vi "PLC_comm-Modified.vi"() -> ()   [LabVIEW 2017]
uses:
  <vilib>/Utility/error.llb/DialogType.ctl
  Control/PLC_Comm_State.ctl
  <vilib>/DATA AHEAD/SP7/typedefs/PLC Type.ctl
  <vilib>/DATA AHEAD/SP7/typedefs/S7 Connection.ctl
  f53d9a16-31ea-4c58-9ec6-4ab155e6634a.vi
  b767813d-b0bc-4642-82b7-59e8eeaf8486.vi
  cf2a4f70-d875-4391-b4be-4b1ea527ec99.vi
  ee8abbcb-1732-468d-97ec-3952c14652c8.vi
  b1e76c00-34b1-4c80-90c6-025f7ce7f41f.vi
  f2e501b8-8033-40fd-b99e-90a89dd29cf5.vi
  90770c14-337c-420b-89b5-e528e61782e2.vi
  a17ecfbb-e8aa-4e6f-9723-a9b27e8c0652.vi
  7947ba3e-47d3-4313-89af-b8503fb010f5.vi
  adc7d8b8-ea76-443b-992e-07ffa118bf03.vi
  515b9a70-e7fd-440a-92eb-3997303c16bf.vi
  5f64c4b0-8bc9-4820-bee4-0d99e36e3286.vi
  3deaaee4-0312-4209-8b7c-ccc637c44985.vi
  e6818258-ddc9-43a8-9628-6e9a25c2df97.vi
  <vilib>/addons/database/Connection.llb/DB Tools Open Connec (String).vi
  <vilib>/DATA AHEAD/SP7/functions/write/write Dint array.vi
  Global/DATA LOG.vi
  <vilib>/DATA AHEAD/SP7/functions/read/read String.vi
  <vilib>/DATA AHEAD/SP7/functions/read/read Dint array.vi
  Global/Global 1.vi
  <vilib>/DATA AHEAD/SP7/functions/write/writeString.vi
  <vilib>/DATA AHEAD/SP7/functions/read/read real array.vi
  <vilib>/addons/database/NI_Database_API.lvlib
  <vilib>/DATA AHEAD/SP7/SP7.lvlib
  84f8396c-11e3-4f6e-927f-d6cb52f8486f.vi
  edb3f7e3-deb4-4efd-b63a-82a20ab466dd.vi
  737c4a97-5810-4f09-bfe1-7e6a970161fd.vi
  98a23aa7-5d76-4ce5-89a1-7ffa2d6e86d6.vi
  065602cd-1ec6-46a4-aff5-3b00a0c776c3.vi
panel:
  out "error out 4":errorcluster
  out "error out 3":errorcluster
  out "IP1 8":string
  out "PLC 8":bool
  out "IP1 7":string
  out "PLC 7":bool
  out "IP1 6":string
  out "PLC 6":bool
  out "IP1 5":string
  out "PLC 5":bool
  out "PLC 4":bool
  out "PLC 3":bool
  out "PLC 1":bool
  out "IP1 4":string
  out "IP1 3":string
  out "IP1 2":string
  out "IP1":string
  in  "stop":bool
  out "error out":errorcluster
  in  "error in (no error)":errorcluster
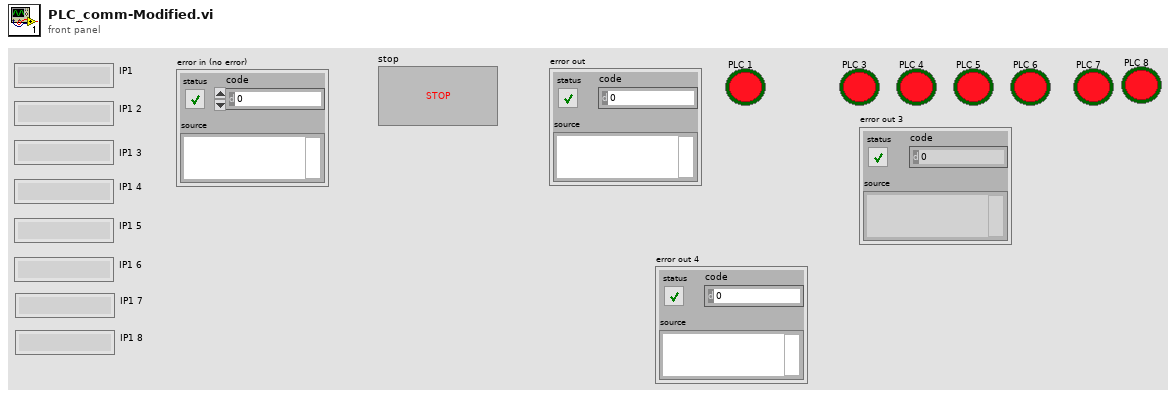
[diagram p1: front panel]
types:
  T1 = typedef "PLC_Comm_State.ctl" = enum16{"Int", "Connect", "Write", "Write2", "Write3", "Read", "Read2", "Read3", "Error", "Disconnect"}
  T2 = typedef "DialogType.ctl" = u16
  T3 = typedef "NI_Database_API.lvlib/Conn ObjectReference.ctl" = refnum<k1>
  T4 = typedef "SP7.lvlib/PLC Type.ctl" = enum16{"S7 200", "S7 300/400", "S7 1200", "S7 1500", "LOGO!8"}
  T5 = typedef "SP7.lvlib/S7 Connection.ctl" = cluster{"TCP Connection Ref":refnum<k5>, "IP address":string, "timeout ms":i32, "Connected?":bool, "PLC Type":T4, "Rack S7 400":u8, "Slot S7 400":u8, "PDU Size":u16, "connection semaphore":T6}
  T6 = typedef "Semaphore RefNum" = refnum<k1>
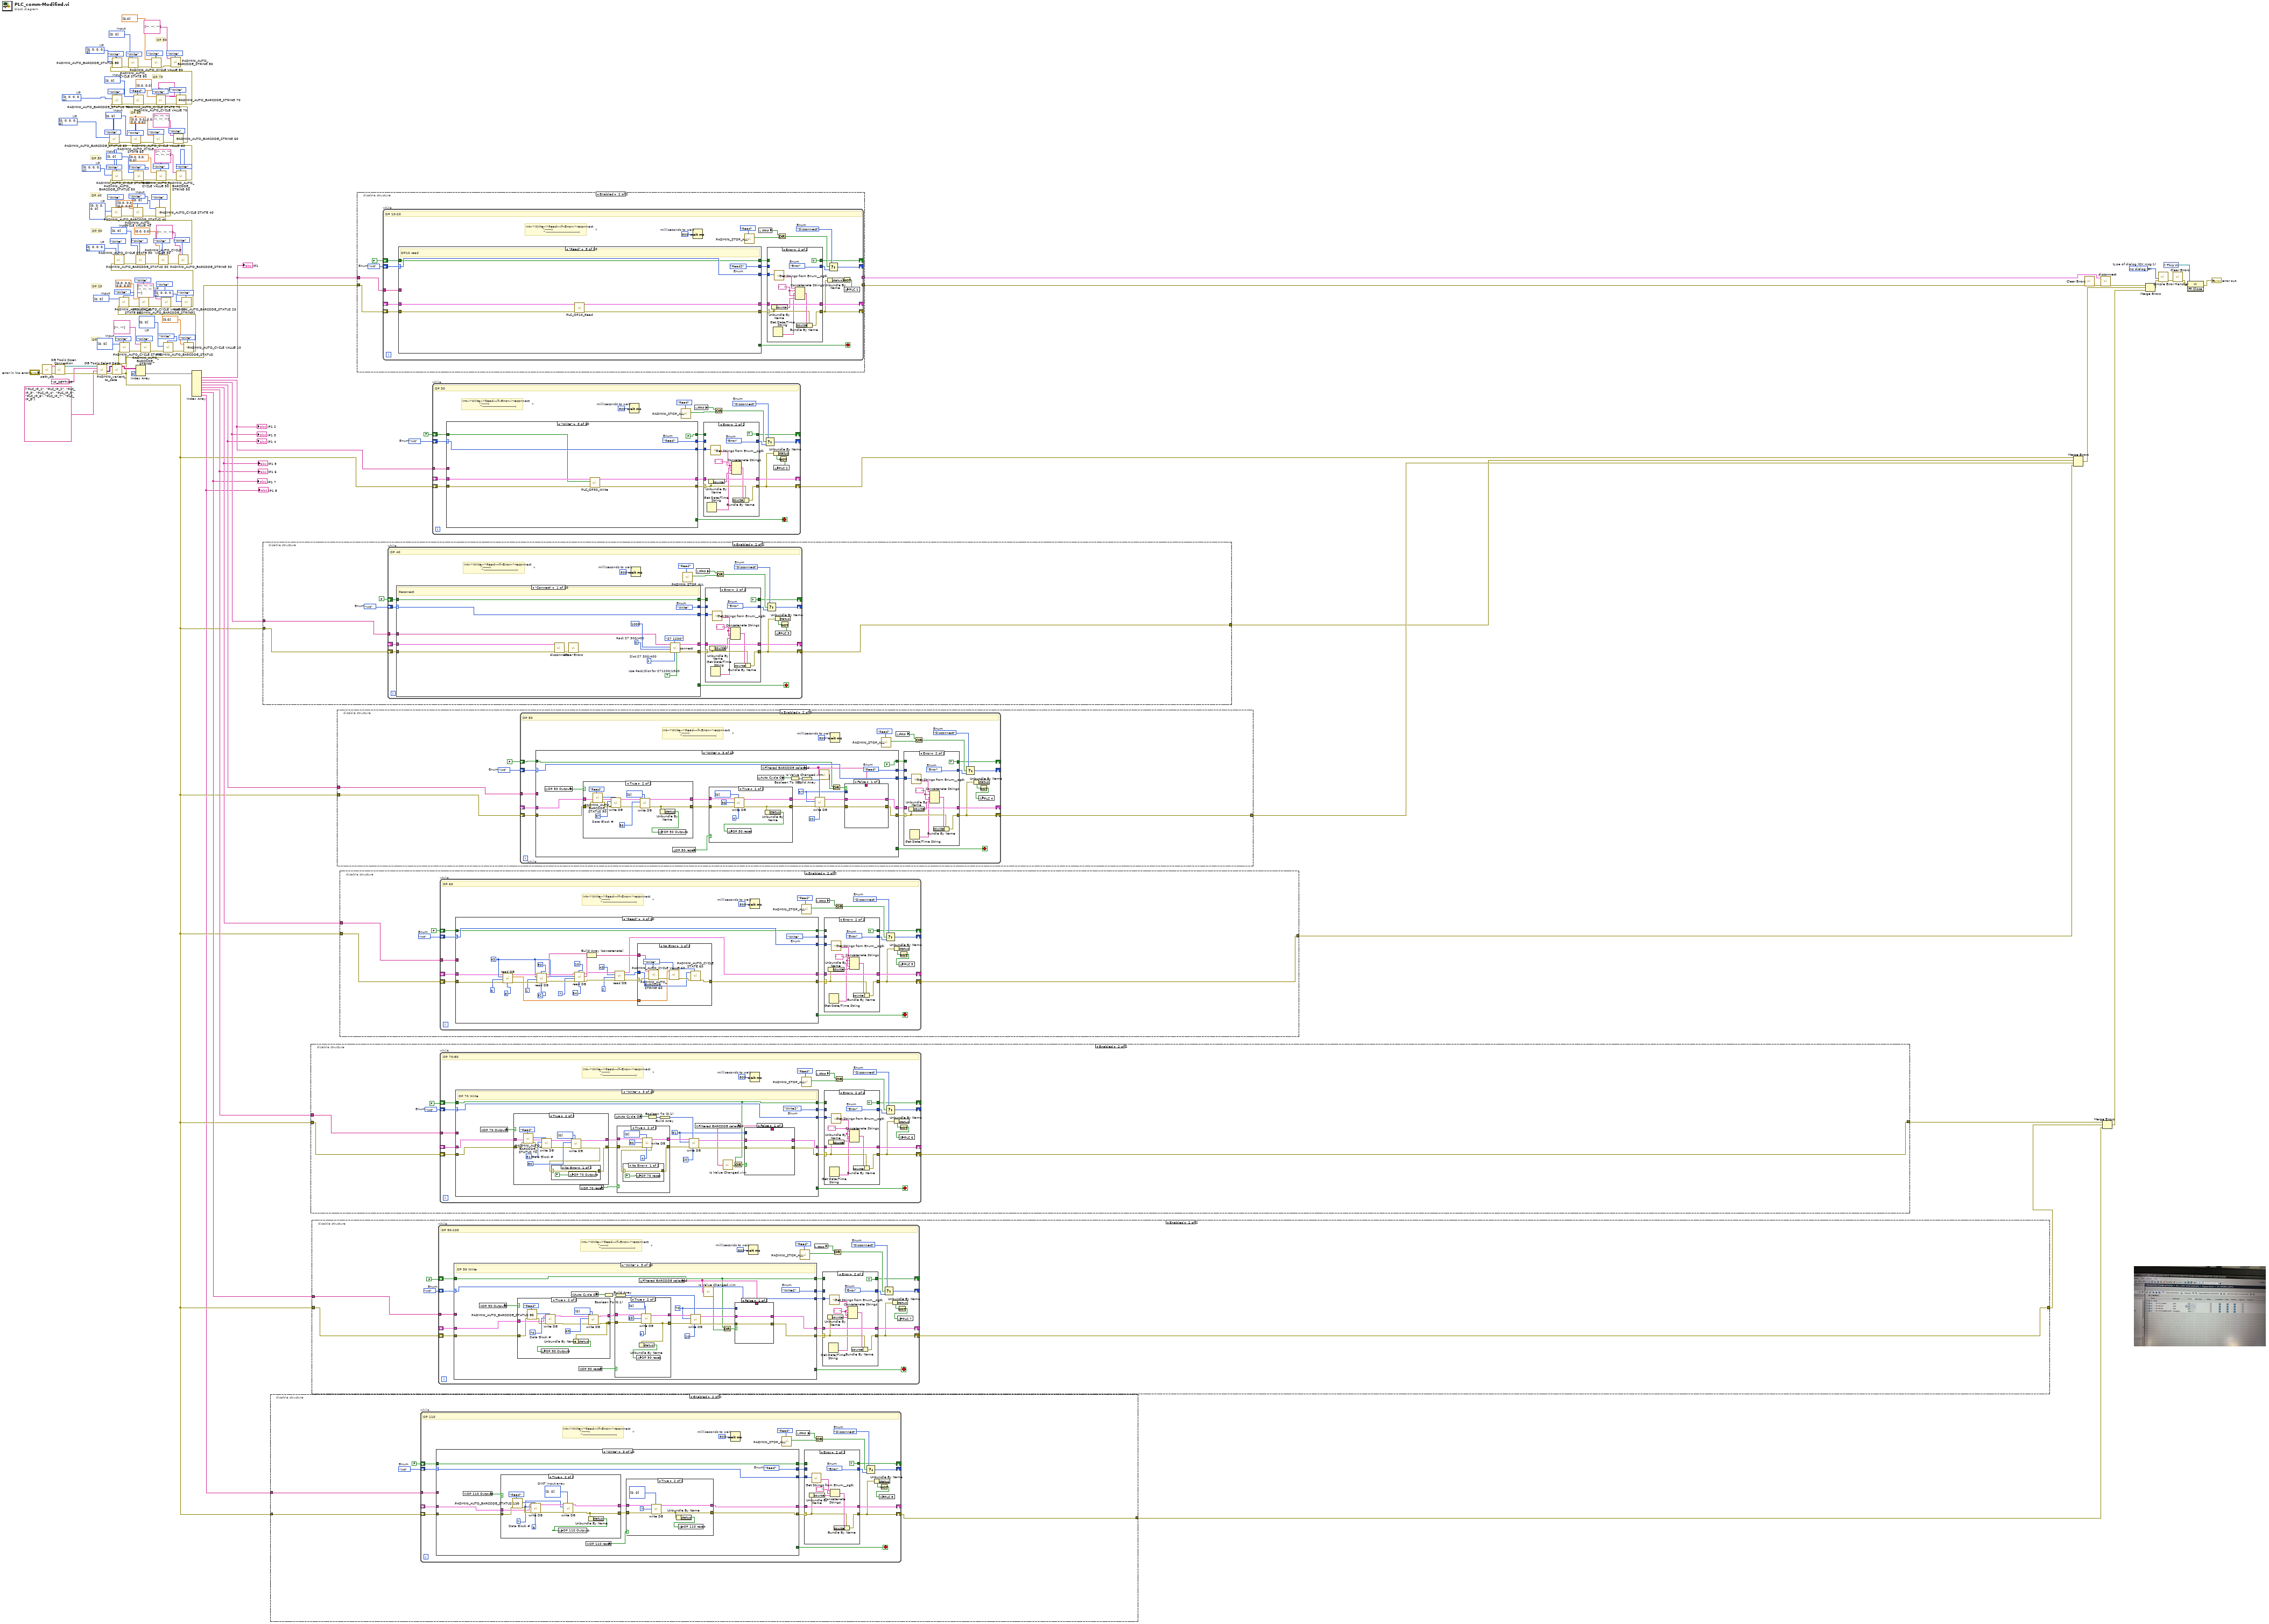
[diagram p0: block diagram]
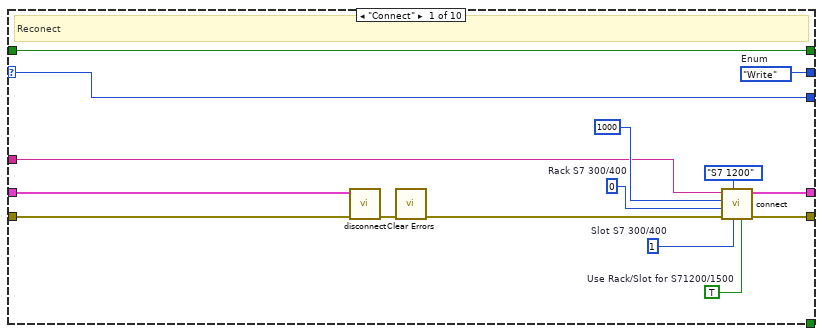
[diagram p3: hidden frame]
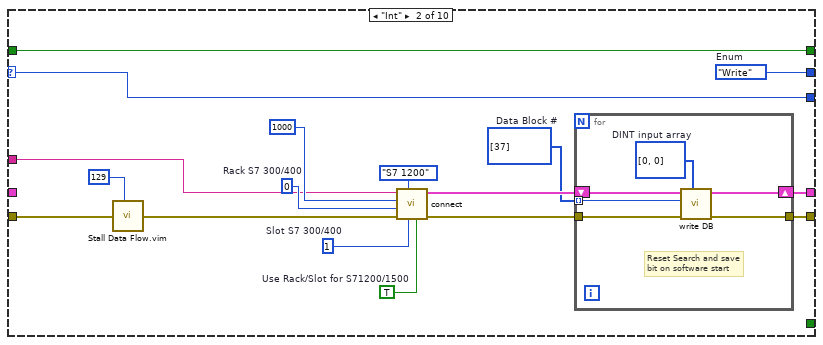
[diagram p4: hidden frame]
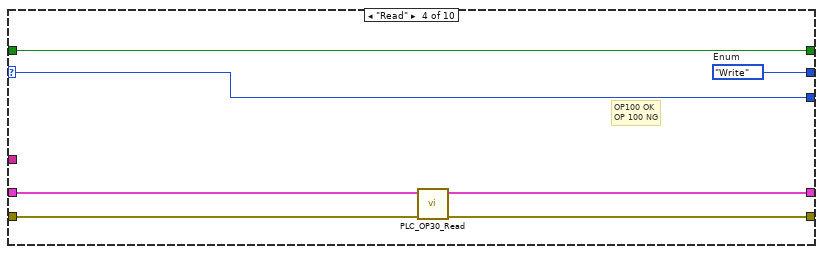
[diagram p5: hidden frame]
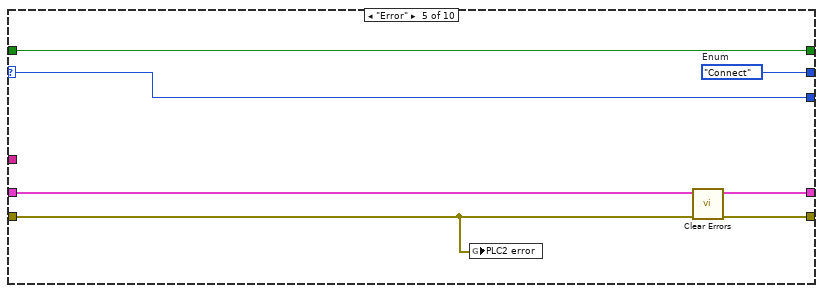
[diagram p6: hidden frame]
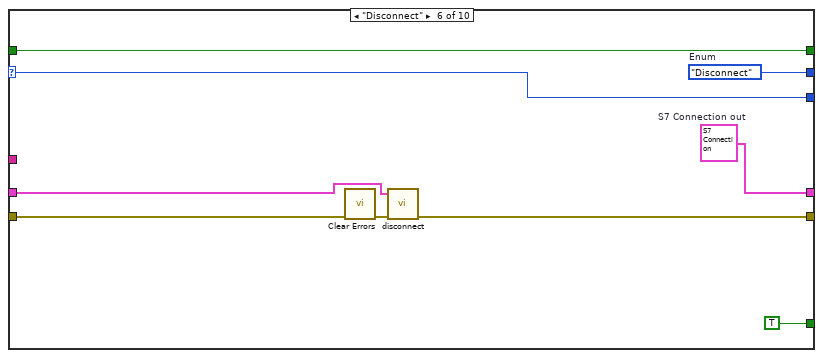
[diagram p7: hidden frame]
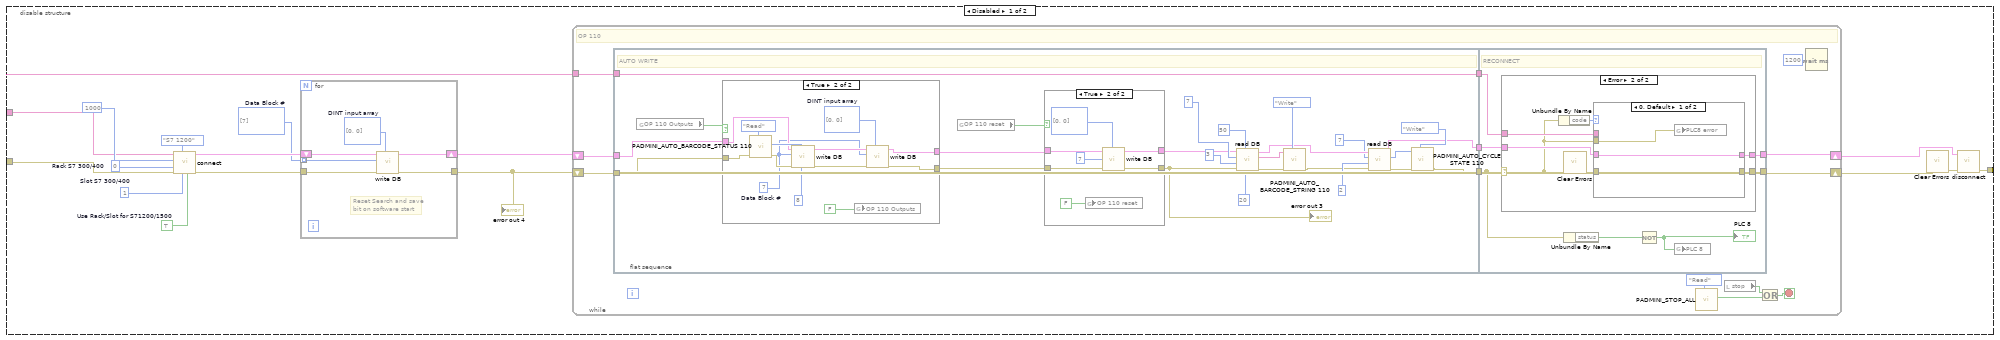
[diagram p12: hidden frame]
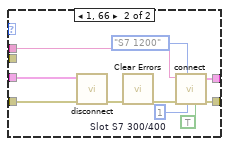
[diagram p16: hidden frame]
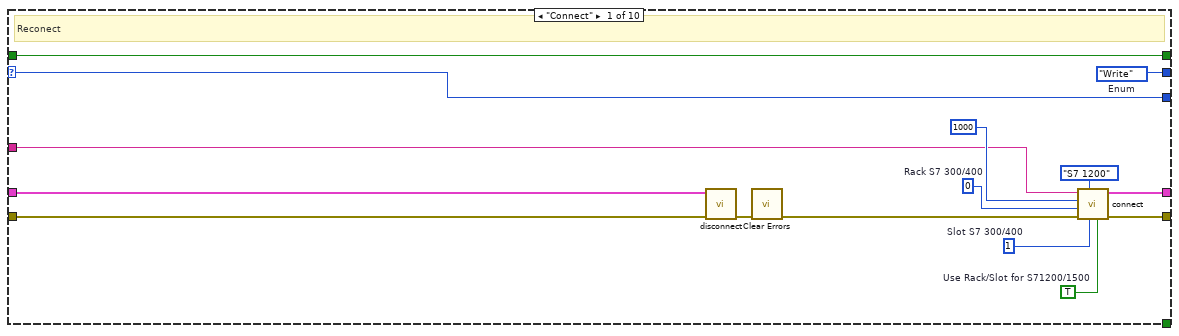
[diagram p18: hidden frame]
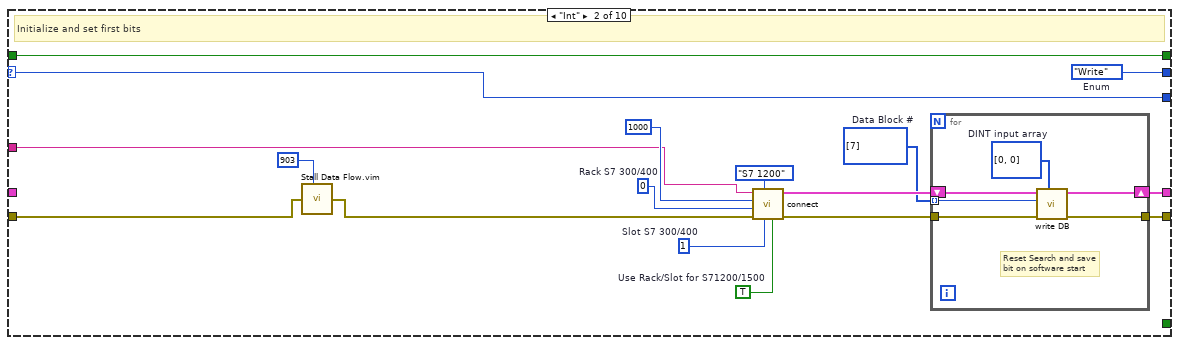
[diagram p19: hidden frame]
diagram:
  w2 = PLC_Comm_State."Int"  # Enum
  w11 = T2 0 items=["no dialog", "OK message", "continue or stop message", "OK message + warnings", "continue/stop + warnings"]  # type of dialog (OK msg:1)
  w13 = i32[] [0, 0, 0, 0, 0]  # I/P
  w14 = i32[] [0, 0]  # Input
  w16 = i32[] [0, 0]  # Input
  w17 = i32[] [0, 0]  # Input
  w19 = i32[] [0, 0]  # Input
  w15 = i32[] [0, 0, 0, 0, 0]  # I/P
  w18 = i32[] [0, 0, 0, 0, 0]  # I/P
  w20 = i32[] [0, 0, 0, 0, 0]  # I/P
  w21 = i32[] [0, 0, 0, 0, 0]  # I/P
  w22 = i32[] [0, 0]  # Input
  w23 = i32[] [0, 0]  # Input
  w24 = i32[] [0, 0, 0, 0, 0]  # I/P
  w25 = i32[] [0, 0, 0, 0, 0]  # I/P
  w26 = i32[] [0, 0]  # Input
  w27 = i32[] [0, 0]  # I/P
  w28 = i32[] [0, 0]  # Input
  # "OP 80"
  # "OP 70"
  # "OP 60"
  # "OP 50"
  # "OP 40"
  # "OP 30"
  # "OP 20"
  # "OP 10"
  n1 = call "path_db.vi"("error in"="error in (no error)") -> ("error out"=w129:errorcluster, "resulting string"=w134:string)  [unwired: 9 in]
  n2 = call-poly <vilib>:"DB Tools Open Connection.vi"("error in (no error)"=w129, "connection information"=w134) -> ("error out"=w133:errorcluster, "connection reference"=w132:T3)  [unwired: 6 in]
  n3 = call <vilib>:"DB Tools Select Data.vi"("error in (no error)"=w133, "columns"=string[] ["PLC_IP_1", "PLC_IP_2", "PLC_IP_3", "PLC_IP_4", "PLC_IP_5", "PLC_IP_6", "PLC_IP_7", "PLC_IP_8"], "table"="IP_SETTING", "connection reference"=w132) -> ("error out"=w131:errorcluster, "data"=w130:variant[][])  [unwired: 2 in, 1 out]
  n4 = call "PADMINI_varient_to_data.vi"("error in (no error)"=w131, "data"=w130) -> ("error out"=w10:errorcluster, "Array"=w125:string[][])  [unwired: 8 in]
  n5 = call "PADMINI_AUTO_CYCLE STATE.vi"("Enum"=enum16{"Read", "Write"}."Write", "error in (no error)"=w10, "Input"=w28) -> ("error out"=w115:errorcluster)  [unwired: 7 in, 1 out]
  n6 = Index Array(array=w125, index (row)=0) -> (element=w124:string[])  [unwired: 1 in]
  n7 = call "PADMINI_AUTO_BARCODE_STRING.vi"("Enum"=enum16{"Read", "Write"}."Write", "error in (no error)"=w115, "Input"=string[] ["", ""]) -> ("error out"=w112:errorcluster)  [unwired: 7 in, 1 out]
  n8 = call "PADMINI_AUTO_BARCODE_STATUS.vi"("Enum"=enum16{"Read", "Write"}."Write", "error in (no error)"=w112, "I/P"=w27) -> ("error out"=w110:errorcluster)  [unwired: 7 in, 1 out]
  n9 = call "PADMINI_AUTO_CYCLE VALUE 10.vi"("Enum"=enum16{"Read", "Write"}."Write", "error in (no error)"=w110, "Input"=dbl[] [0.0]) -> ("error out"=w104:errorcluster)  [unwired: 7 in, 1 out]
  n10 = call "PADMINI_AUTO_CYCLE STATE 20.vi"("Enum"=enum16{"Read", "Write"}."Write", "error in (no error)"=w104, "Input"=w14) -> ("error out"=w102:errorcluster)  [unwired: 7 in, 1 out]
  n11 = call "PADMINI_AUTO_CYCLE VALUE 20.vi"("Enum"=enum16{"Read", "Write"}."Write", "error in (no error)"=w102, "Input"=dbl[] [0.0, 0.0, 0.0, 0.0]) -> ("error out"=w98:errorcluster)  [unwired: 7 in, 1 out]
  n12 = call "PADMINI_AUTO_BARCODE_STRING2.vi"("Enum"=enum16{"Read", "Write"}."Write", "error in (no error)"=w98, "Input"=string[] ["", "", "", "", "", "", ""]) -> ("error out"=w96:errorcluster)  [unwired: 7 in, 1 out]
  n13 = call "PADMINI_AUTO_BARCODE_STATUS 20.vi"("Enum"=enum16{"Read", "Write"}."Write", "error in (no error)"=w96, "I/P"=w13) -> ("error out"=w94:errorcluster)  [unwired: 7 in, 1 out]
  n14 = call "PADMINI_AUTO_BARCODE_STATUS 30.vi"("Enum"=enum16{"Read", "Write"}."Write", "error in (no error)"=w94, "I/P"=w15) -> ("error out"=w91:errorcluster)  [unwired: 7 in, 1 out]
  n15 = call "PADMINI_AUTO_CYCLE STATE 30.vi"("Enum"=enum16{"Read", "Write"}."Write", "error in (no error)"=w91, "Input"=w16) -> ("error out"=w90:errorcluster)  [unwired: 7 in, 1 out]
  n16 = call "PADMINI_AUTO_CYCLE VALUE 30.vi"("Enum"=enum16{"Read", "Write"}."Write", "error in (no error)"=w90, "Input"=dbl[] [0.0, 0.0]) -> ("error out"=w87:errorcluster)  [unwired: 7 in, 1 out]
  n17 = call "PADMINI_AUTO_BARCODE_STRING 30.vi"("Enum"=enum16{"Read", "Write"}."Write", "error in (no error)"=w87, "Input"=string[] ["", "", ""]) -> ("error out"=w77:errorcluster)  [unwired: 7 in, 1 out]
  n18 = call "PADMINI_AUTO_BARCODE_STATUS 40.vi"("Enum"=enum16{"Read", "Write"}."Write", "error in (no error)"=w77, "I/P"=w18) -> ("error out"=w76:errorcluster)  [unwired: 7 in, 1 out]
  n19 = call "PADMINI_AUTO_CYCLE VALUE 40.vi"("Enum"=enum16{"Read", "Write"}."Write", "error in (no error)"=w76, "Input"=dbl[] [0.0, 0.0, 0.0, 0.0]) -> ("error out"=w75:errorcluster)  [unwired: 7 in, 1 out]
  n20 = call "PADMINI_AUTO_CYCLE STATE 40.vi"("Enum"=enum16{"Read", "Write"}."Write", "error in (no error)"=w75, "Input"=w17) -> ("error out"=w74:errorcluster)  [unwired: 7 in, 1 out]
  n21 = call "PADMINI_AUTO_BARCODE_STATUS 50.vi"("Enum"=enum16{"Read", "Write"}."Write", "error in (no error)"=w74, "I/P"=w20) -> ("error out"=w66:errorcluster)  [unwired: 7 in, 1 out]
  n22 = call "PADMINI_AUTO_CYCLE STATE 50.vi"("Enum"=enum16{"Read", "Write"}."Write", "error in (no error)"=w66, "Input"=w19) -> ("error out"=w70:errorcluster)  [unwired: 7 in, 1 out]
  n23 = call "PADMINI_AUTO_CYCLE VALUE 50.vi"("Enum"=enum16{"Read", "Write"}."Write", "error in (no error)"=w70, "Input"=dbl[] [0.0, 0.0, 0.0]) -> ("error out"=w67:errorcluster)  [unwired: 7 in, 1 out]
  n24 = call "PADMINI_AUTO_BARCODE_STRING 50.vi"("Enum"=enum16{"Read", "Write"}."Write", "error in (no error)"=w67, "Input"=string[] ["", "", "", "", "", ""]) -> ("error out"=w52:errorcluster)  [unwired: 7 in, 1 out]
  n25 = call "PADMINI_AUTO_BARCODE_STATUS 60.vi"("Enum"=enum16{"Read", "Write"}."Write", "error in (no error)"=w52, "I/P"=w21) -> ("error out"=w56:errorcluster)  [unwired: 7 in, 1 out]
  n26 = call "PADMINI_AUTO_CYCLE STATE 60.vi"("Enum"=enum16{"Read", "Write"}."Write", "error in (no error)"=w56, "Input"=w22) -> ("error out"=w58:errorcluster)  [unwired: 7 in, 1 out]
  n27 = call "PADMINI_AUTO_CYCLE VALUE 60.vi"("Enum"=enum16{"Read", "Write"}."Write", "error in (no error)"=w58, "Input"=dbl[] [0.0, 0.0, 0.0, 0.0, 0.0]) -> ("error out"=w61:errorcluster)  [unwired: 7 in, 1 out]
  n28 = call "PADMINI_AUTO_BARCODE_STRING 60.vi"("Enum"=enum16{"Read", "Write"}."Write", "error in (no error)"=w61, "Input"=string[] ["", "", "", "", "", ""]) -> ("error out"=w35:errorcluster)  [unwired: 7 in, 1 out]
  n29 = call "PADMINI_AUTO_BARCODE_STATUS 70.vi"("Enum"=enum16{"Read", "Write"}."Write", "error in (no error)"=w35, "I/P"=w24) -> ("error out"=w38:errorcluster)  [unwired: 7 in, 1 out]
  n30 = call "PADMINI_AUTO_CYCLE STATE 70.vi"("Enum"=enum16{"Read", "Write"}."Read", "error in (no error)"=w38, "Input"=w23) -> ("error out"=w50:errorcluster)  [unwired: 7 in, 1 out]
  n31 = call "PADMINI_AUTO_CYCLE VALUE 70.vi"("Enum"=enum16{"Read", "Write"}."Write", "error in (no error)"=w50, "Input"=dbl[] [0.0, 0.0]) -> ("error out"=w47:errorcluster)  [unwired: 7 in, 1 out]
  n32 = call "PADMINI_AUTO_BARCODE_STRING 70.vi"("Enum"=enum16{"Read", "Write"}."Write", "error in (no error)"=w47, "Input"=string[] ["", ""]) -> ("error out"=w32:errorcluster)  [unwired: 7 in, 1 out]
  n33 = call "PADMINI_AUTO_BARCODE_STATUS 80.vi"("Enum"=enum16{"Read", "Write"}."Write", "error in (no error)"=w32, "I/P"=w25) -> ("error out"=w39:errorcluster)  [unwired: 7 in, 1 out]
  n34 = call "PADMINI_AUTO_CYCLE STATE 80.vi"("Enum"=enum16{"Read", "Write"}."Write", "error in (no error)"=w39, "Input"=w26) -> ("error out"=w43:errorcluster)  [unwired: 7 in, 1 out]
  n35 = call "PADMINI_AUTO_CYCLE VALUE 80.vi"("Enum"=enum16{"Read", "Write"}."Write", "error in (no error)"=w43, "Input"=sgl[] [0.0]) -> ("error out"=w46:errorcluster)  [unwired: 7 in, 1 out]
  n36 = call "PADMINI_AUTO_BARCODE_STRING 80.vi"("Enum"=enum16{"Read", "Write"}."Write", "error in (no error)"=w46, "Input"=string[] ["", "", ""]) -> ()  [unwired: 7 in, 2 out]
  n37 = Index Array(array=w124) -> (element #1=w83:string, element #2=w84:string, element #3=w82:string, element #4=w72:string, element #5=w62:string, element #6=w31:string, element #7=w30:string, element #8=w9:string)  [unwired: 8 in]
  "IP1" <- w83
  "IP1 2" <- w84
  "IP1 3" <- w82
  "IP1 4" <- w72
  "IP1 5" <- w62
  "IP1 6" <- w31
  "IP1 7" <- w30
  "IP1 8" <- w9
  n38 = disable-structure shown="Enabled" {
    disable-tunnel: w82 -> [w149 w272]
    disable-tunnel: w10 -> [w140 w271]
    disable-tunnel: [w135 w270] -> w4
    frame Disabled {
      w137 = TRUE  # Use Rack/Slot for S71200/1500
      w138 = u8 0  # Rack S7 300/400
      w139 = u8 1  # Slot S7 300/400
      w145 = i32[] [0, 0]  # DINT input array
      # "Reset Search and save \nbit on software start"
      n39 = call <vilib>:"connect.vi"("Use Rack/Slot for S71200/1500"=w137, "Slot S7 300/400"=w139, "PLC Type"=PLC_Type."S7 1200" ("PLC Type 2"), "error in (no error)"=w140, "Rack S7 300/400"=w138, "timeout [ms]"=1000 ("timeout [ms] 2"), "IP address"=w149) -> ("error out"=w142:errorcluster, "S7 Connection out"=w141:T5)  [unwired: 3 in]
      n40 = call-poly <vilib>:"write DB.vi"("DINT input array"=w145, "error in (no error)"=w142, "Data Block #"=u16 56, "S7 Connection in"=w141) -> ("error out"=w144:errorcluster, "S7 Connection out"=w143:T5)  [unwired: 4 in, 2 out]
      n41 = while {
        shift-right: [w154] -> w147
        shift-left: w143 -> [w164]
        shift-right: [w162] -> w148
        shift-left: w144 -> [w163]
        tunnel: w149 -> [w153]
        stop <- w156 stop-if-true
        # "OP 40"
        n42 = flat-sequence {
          tunnel: [w166] -> w160
          tunnel: [w169] -> w155
          tunnel: w163 -> [w214]
          tunnel: w164 -> [w213]
          tunnel: w153 -> [w201]
          tunnel: [w201] -> w152
          tunnel: [w242] -> w162
          tunnel: [w241] -> w154
          tunnel: w160 -> [w244]
          tunnel: w155 -> [w243]
          tunnel: w152 -> [w240]
          frame #0 {
            w194 = u16 57 ("Data Block #")
            w165 = u16 56 ("Data Block #")
            # "AUTO WRITE"
            n43 = global read "DATA LOG.vi" "OP 40 Outputs"() -> (w212:bool)
            n44 = case shown="True" w212 {
              tunnel: w213 -> [w225 w238]
              tunnel: [w226 w230] -> w199
              tunnel: [w225 w232] -> w200
              tunnel: w214 -> [w226 w235]
              frame False {
              }
              frame True {
                w239 = u16 57  # Data Block #
                n45 = call "PADMINI_AUTO_BARCODE_STATUS 40.vi"("Enum"=enum16{"Read", "Write"}."Read", "error in (no error)"=w235) -> ("error out"=w234:errorcluster, "O/P"=w236:i32[])  [unwired: 8 in]
                n46 = global write "DATA LOG.vi" "OP 40 Outputs"(FALSE) -> ()
                n47 = call-poly <vilib>:"write DB.vi"("DINT input array"=w236, "error in (no error)"=w234, "Data Block #"=w239, "S7 Connection in"=w238) -> ("error out"=w229:errorcluster, "S7 Connection out"=w231:T5)  [unwired: 4 in, 2 out]
                n48 = call-poly <vilib>:"write DB.vi"("DINT input array"=i32[] [0], "error in (no error)"=w229, "Data Block #"=u16 56, "S7 Connection in"=w231) -> ("error out"=w230:errorcluster, "S7 Connection out"=w232:T5)  [unwired: 4 in, 2 out]
              }
            }
            n49 = global read "DATA LOG.vi" "OP 40 reset"() -> (w198:bool)
            n50 = global read "DATA LOG.vi" "Auto Cycle On"() -> (w176:bool)
            n51 = case shown="True" w198 {
              tunnel: w199 -> [w215 w224]
              tunnel: [w215 w223] -> w187
              tunnel: w200 -> [w216 w222]
              tunnel: [w216 w221] -> w188
              frame False {
              }
              frame True {
                n52 = global write "DATA LOG.vi" "OP 40 reset"(FALSE) -> ()
                n53 = call-poly <vilib>:"write DB.vi"("Item offset [byte]"=u16 4 ("Data Block #"), "DINT input array"=i32[] [0], "error in (no error)"=w224, "Data Block #"=u16 56, "S7 Connection in"=w222) -> ("error out"=w223:errorcluster, "S7 Connection out"=w221:T5)  [unwired: 3 in, 2 out]
              }
            }
            n54 = Boolean To (0,1)(Boolean=w176) -> (0, 1=w175:i16)
            n55 = Build Array(w175) -> (w174:i16[])
            n56 = global read "Global 1.vi" "Filtered BARCODE selected"() -> (w197:string[])
            n57 = call-poly <vilib>:"write DB.vi"("Item offset [byte]"=u32 20, "DINT input array"=w174, "error in (no error)"=w187, "Data Block #"=w194, "S7 Connection in"=w188) -> ("error out"=w192:errorcluster, "S7 Connection out"=w191:T5)  [unwired: 3 in, 2 out]
            n58 = call-poly <vilib>:"write DB.vi"("Item offset [byte]"=u32 24, "Input STRINGS"=w197, "error in (no error)"=w192, "String length reserved in DB (default=254)"=u16 15, "Data Block #"=w194, "S7 Connection in"=w191) -> ("error out"=w189:errorcluster, "S7 Connection out"=w190:T5)  [unwired: 2 in, 2 out]
            n59 = call-poly <vilib>:"read DB.vi"("Item offset [byte]"=u32 8, "error in (no error)"=w189, "items #"=u16 4 ("Items # [byte]"), "Data Block #"=w165, "S7 Connection in"=w190) -> ("error out"=w204:errorcluster, "REAL result array"=w202:sgl[], "S7 Connection out"=w210:T5)  [unwired: 4 in]
            n60 = call "PADMINI_AUTO_CYCLE VALUE 40.vi"("Enum"=enum16{"Read", "Write"}."Write", "error in (no error)"=w204, "Input"=w202) -> ("error out"=w203:errorcluster)  [unwired: 7 in, 1 out]
            n61 = call-poly <vilib>:"read DB.vi"("Item offset [byte]"=u32 24, "String length reserved in DB (default=254)"=u16 50, "error in (no error)"=w203, "items #"=u16 1 ("Items # [byte]"), "Data Block #"=w165, "S7 Connection in"=w210) -> ("error out"=w186:errorcluster, "STRING result Array"=w179:string[], "S7 Connection out"=w184:T5)  [unwired: 2 in, 1 out]
            n62 = call-poly <vilib>:"read DB.vi"("Item offset [byte]"=u32 76, "String length reserved in DB (default=254)"=u16 10, "error in (no error)"=w186, "items #"=u16 4 ("Items # [byte]"), "Data Block #"=w165, "S7 Connection in"=w184) -> ("error out"=w185:errorcluster, "STRING result Array"=w178:string[], "S7 Connection out"=w167:T5)  [unwired: 2 in, 1 out]
            n63 = Build Array (concatenate)(w179, w178) -> (w177:string[])
            n64 = call "PADMINI_AUTO_BARCODE_STRING 40.vi"("Enum"=enum16{"Read", "Write"}."Write", "error in (no error)"=w185, "Input"=w177) -> ("error out"=w168:errorcluster)  [unwired: 7 in, 1 out]
            n65 = call-poly <vilib>:"read DB.vi"("error in (no error)"=w168, "items #"=u16 2 ("Items # [byte]"), "Data Block #"=w165, "S7 Connection in"=w167) -> ("error out"=w173:errorcluster, "DINT result array"=w172:i32[], "S7 Connection out"=w166:T5)  [unwired: 5 in]
            n66 = call "PADMINI_AUTO_CYCLE STATE 40.vi"("Enum"=enum16{"Read", "Write"}."Write", "error in (no error)"=w173, "Input"=w172) -> ("error out"=w169:errorcluster)  [unwired: 7 in, 1 out]
          }
          frame #1 {
            # "RECONNECT"
            n67 = case shown="Error" w243 {
              selector: w243 -> [w248 w249]
              tunnel: [w247 w253] -> w241
              tunnel: [w248 w254] -> w242
              tunnel: w244 -> [w247 w252]
              tunnel: w240 -> [_ w251]
              frame No Error {
              }
              frame Error {
                n68 = Unbundle By Name(w249) -> ("code"=w250:i32)
                n69 = call <vilib>:"Clear Errors.vi"("error in (no error)"=w249) -> ("error out"=w255:errorcluster)  [unwired: 5 in, 1 out]
                n70 = case shown="1" w250 {
                  tunnel: w255 -> [w257 w268]
                  tunnel: [w257 w266] -> w254
                  tunnel: [w258 w265] -> w253
                  tunnel: w252 -> [w258 w262]
                  tunnel: w251 -> [_ w261]
                  tunnel: w249 -> [w256 _]
                  frame 0, Default {
                    n71 = global write "Global 1.vi" "PLC3 error"(w256) -> ()
                  }
                  frame 1 {
                    n72 = call <vilib>:"disconnect.vi"("error in (no error)"=w268, "S7 Connection in"=w262) -> ("error out"=w267:errorcluster)  [unwired: 8 in, 1 out]
                    n73 = call <vilib>:"Clear Errors.vi"("error in (no error)"=w267) -> ("error out"=w264:errorcluster)  [unwired: 5 in, 1 out]
                    n74 = call <vilib>:"connect.vi"("Use Rack/Slot for S71200/1500"=TRUE, "Slot S7 300/400"=u8 1, "PLC Type"=PLC_Type."S7 1200" ("PLC Type 2"), "error in (no error)"=w264, "IP address"=w261) -> ("error out"=w266:errorcluster, "S7 Connection out"=w265:T5)  [unwired: 5 in]
                  }
                }
              }
            }
            n75 = Unbundle By Name(w243) -> ("status"=w246:bool)
            n76 = Not(x=w246) -> (.not. x?=w245:bool)
            "PLC 3" <- w245
            n77 = global write "Global 1.vi" "PLC 3"(w245) -> ()
          }
        }
        n78 = call "PADMINI_STOP_ALL.vi"("Enum"=enum16{"Read", "Write"}."Read") -> ("Boolean 2"=w158:bool)  [unwired: 9 in, 1 out]
        n79 = local read "stop"() -> (w157:bool)
        n80 = Or(x=w157, y=w158) -> (x .or. y?=w156:bool)
        n81 = Wait (ms)(milliseconds to wait=u32 1200) -> ()  [unwired: 1 out]
      }
      n82 = call <vilib>:"Clear Errors.vi"("error in (no error)"=w148) -> ("error out"=w136:errorcluster)  [unwired: 5 in, 1 out]
      n83 = call <vilib>:"disconnect.vi"("error in (no error)"=w136, "S7 Connection in"=w147) -> ("error out"=w135:errorcluster)  [unwired: 8 in, 1 out]
    }
    frame Enabled {
      w273 = PLC_Comm_State."Int"  # Enum
      n84 = while {
        shift-right: [w287] -> _
        shift-left: w273 -> [w296]
        shift-right: [w277] -> w270
        shift-left: w271 -> [w295]
        shift-right: [w290] -> _
        shift-left: _ -> [w294]
        tunnel: w272 -> [w293]
        shift-right: [w276] -> _
        shift-left: FALSE -> [w274]
        stop <- w288 stop-if-true
        w284 = PLC_Comm_State."Disconnect"  # Enum
        w292 = u32 800  # milliseconds to wait
        # "Int-->Write-->Read---if--Error-->reconnect\n               ^------v                                       v\n                ^------------------------------v"
        # "OP 40"
        n85 = case shown="\"Connect\"" w296 {
          selector: w296 -> [w315 w334 w374 w438 w451 w456 _ _ _ _]
          tunnel: [w320 w336 w358 w413 w452 w461 w464 w468 w471 w474] -> w297
          tunnel: [w321 w332 w356 w411 w453 w458 w465 w467 w470 w473] -> w289
          tunnel: w295 -> [w318 w330 w359 w414 w449 w459 w464 w468 w471 w474]
          tunnel: w294 -> [w316 _ w357 w412 w453 w460 w465 w467 w470 w473]
          tunnel: w293 -> [w322 w335 _ _ _ _ _ _ _ _]
          tunnel: [w314 w333 w373 w437 w450 w455 _ _ _ _] -> w291
          tunnel: [_ _ _ _ _ TRUE _ _ _ _] -> w288
          tunnel: [w315 w334 w374 w438 w451 w456 _ _ _ _] -> w285
          tunnel: [w313 w328 FALSE w410 w448 w454 w463 w466 w469 w472] -> w275
          tunnel: w274 -> [w313 w328 w352 w410 w448 w454 w463 w466 w469 w472]
          frame "Connect" {
            w314 = PLC_Comm_State."Write"  # Enum
            w327 = TRUE  # Use Rack/Slot for S71200/1500
            w326 = u8 1  # Slot S7 300/400
            w324 = u8 0  # Rack S7 300/400
            # "Reconect"
            n86 = call <vilib>:"disconnect.vi"("error in (no error)"=w318, "S7 Connection in"=w316) -> ("error out"=w319:errorcluster)  [unwired: 8 in, 1 out]
            n87 = call <vilib>:"Clear Errors.vi"("error in (no error)"=w319) -> ("error out"=w317:errorcluster)  [unwired: 5 in, 1 out]
            n88 = call <vilib>:"connect.vi"("Use Rack/Slot for S71200/1500"=w327, "Slot S7 300/400"=w326, "PLC Type"=PLC_Type."S7 1200" ("PLC Type 2"), "error in (no error)"=w317, "Rack S7 300/400"=w324, "timeout [ms]"=1000 ("timeout [ms] 2"), "IP address"=w322) -> ("error out"=w320:errorcluster, "S7 Connection out"=w321:T5)  [unwired: 3 in]
          }
          frame "Int" {
            w333 = PLC_Comm_State."Write"  # Enum
            w337 = TRUE  # Use Rack/Slot for S71200/1500
            w338 = u8 1  # Slot S7 300/400
            w339 = u8 0  # Rack S7 300/400
            w340 = u16[] [56]  # Data Block #
            n89 = call "Stall Data Flow.vim"("value in"=w330, "milliseconds to wait"=u32 258) -> ("value out"=w329:errorcluster)  [unwired: 1 out]
            n90 = call <vilib>:"connect.vi"("Use Rack/Slot for S71200/1500"=w337, "Slot S7 300/400"=w338, "PLC Type"=PLC_Type."S7 1200" ("PLC Type 2"), "error in (no error)"=w329, "Rack S7 300/400"=w339, "timeout [ms]"=1000 ("timeout [ms] 2"), "IP address"=w335) -> ("error out"=w342:errorcluster, "S7 Connection out"=w341:T5)  [unwired: 3 in]
            n91 = for {
              tunnel: w340 -> [w350] mode=indexing
              shift-right: [w348] -> w332
              shift-left: w341 -> [w346]
              tunnel: w342 -> [w347]
              tunnel: [w345] -> w336
              w349 = i32[] [0, 0]  # DINT input array
              # "Reset Search and save \nbit on software start"
              n92 = call-poly <vilib>:"write DB.vi"("DINT input array"=w349, "error in (no error)"=w347, "Data Block #"=w350, "S7 Connection in"=w346) -> ("error out"=w345:errorcluster, "S7 Connection out"=w348:T5)  [unwired: 4 in, 2 out]
            }
          }
          frame "Write" {
            w361 = u16 57 ("Data Block #")
            w373 = PLC_Comm_State."Read"  # Enum
            n93 = global read "DATA LOG.vi" "OP 40 Outputs"() -> (w372:bool)
            n94 = case shown="True" w372 {
              tunnel: w357 -> [w395 w397]
              tunnel: [w396 w399] -> w370
              tunnel: [w395 w404] -> w371
              tunnel: w359 -> [w396 w406]
              frame False {
              }
              frame True {
                w409 = u16 57  # Data Block #
                n95 = call "PADMINI_AUTO_BARCODE_STATUS 40.vi"("Enum"=enum16{"Read", "Write"}."Read", "error in (no error)"=w406) -> ("error out"=w405:errorcluster, "O/P"=w407:i32[])  [unwired: 8 in]
                n96 = call-poly <vilib>:"write DB.vi"("DINT input array"=w407, "error in (no error)"=w405, "Data Block #"=w409, "S7 Connection in"=w397) -> ("error out"=w402:errorcluster, "S7 Connection out"=w403:T5)  [unwired: 4 in, 2 out]
                n97 = call-poly <vilib>:"write DB.vi"("DINT input array"=i32[] [0], "error in (no error)"=w402, "Data Block #"=u16 56, "S7 Connection in"=w403) -> ("error out"=w399:errorcluster, "S7 Connection out"=w404:T5)  [unwired: 4 in, 2 out]
                n98 = Unbundle By Name(w399) -> ("status"=w398:bool)
                n99 = global write "DATA LOG.vi" "OP 40 Outputs"(w398) -> ()
              }
            }
            n100 = global read "DATA LOG.vi" "OP 40 reset"() -> (w369:bool)
            n101 = global read "DATA LOG.vi" "Auto Cycle On"() -> (w364:bool)
            n102 = case shown="True" w369 {
              tunnel: w370 -> [w385 w394]
              tunnel: [w385 w389] -> w365
              tunnel: w371 -> [w386 w393]
              tunnel: [w386 w387] -> w366
              frame False {
              }
              frame True {
                n103 = call-poly <vilib>:"write DB.vi"("Item offset [byte]"=u16 4 ("Data Block #"), "DINT input array"=i32[] [0], "error in (no error)"=w394, "Data Block #"=u16 56, "S7 Connection in"=w393) -> ("error out"=w389:errorcluster, "S7 Connection out"=w387:T5)  [unwired: 3 in, 2 out]
                n104 = Unbundle By Name(w389) -> ("status"=w388:bool)
                n105 = global write "DATA LOG.vi" "OP 40 reset"(w388) -> ()
              }
            }
            n106 = Boolean To (0,1)(Boolean=w364) -> (0, 1=w363:i16)
            n107 = global read "Global 1.vi" "Filtered BARCODE selected"() -> (w355:string[])
            n108 = Build Array(w363) -> (w362:i16[])
            n109 = call-poly <vilib>:"write DB.vi"("Item offset [byte]"=u32 20, "DINT input array"=w362, "error in (no error)"=w365, "Data Block #"=w361, "S7 Connection in"=w366) -> ("error out"=w368:errorcluster, "S7 Connection out"=w367:T5)  [unwired: 3 in, 2 out]
            n110 = call "Is Value Changed.vim"("value"=w355) -> ("changed or first call?"=w353:bool)
            n111 = Or(x=w352, y=w353) -> (x .or. y?=w354:bool)
            n112 = case shown="False" w354 {
              tunnel: w355 -> [_ w384]
              tunnel: w368 -> [w375 w383]
              tunnel: w367 -> [w376 w382]
              tunnel: w361 -> [_ w379]
              tunnel: [w375 w378] -> w358
              tunnel: [w376 w377] -> w356
              frame False {
              }
              frame True {
                n113 = call-poly <vilib>:"write DB.vi"("Item offset [byte]"=u32 24, "Input STRINGS"=w384, "error in (no error)"=w383, "String length reserved in DB (default=254)"=u16 15, "Data Block #"=w379, "S7 Connection in"=w382) -> ("error out"=w378:errorcluster, "S7 Connection out"=w377:T5)  [unwired: 2 in, 2 out]
              }
            }
          }
          frame "Read" {
            w423 = u16 56 ("Data Block #")
            w437 = PLC_Comm_State."Write"  # Enum
            n114 = call-poly <vilib>:"read DB.vi"("Item offset [byte]"=u32 8, "error in (no error)"=w414, "items #"=u16 4 ("Items # [byte]"), "Data Block #"=w423, "S7 Connection in"=w412) -> ("error out"=w433:errorcluster, "REAL result array"=w436:sgl[], "S7 Connection out"=w434:T5)  [unwired: 4 in]
            n115 = call-poly <vilib>:"read DB.vi"("Item offset [byte]"=u32 24, "String length reserved in DB (default=254)"=u16 50, "error in (no error)"=w433, "items #"=u16 1 ("Items # [byte]"), "Data Block #"=w423, "S7 Connection in"=w434) -> ("error out"=w432:errorcluster, "STRING result Array"=w429:string[], "S7 Connection out"=w430:T5)  [unwired: 2 in, 1 out]
            n116 = call-poly <vilib>:"read DB.vi"("Item offset [byte]"=u32 76, "String length reserved in DB (default=254)"=u16 10, "error in (no error)"=w432, "items #"=u16 4 ("Items # [byte]"), "Data Block #"=w423, "S7 Connection in"=w430) -> ("error out"=w431:errorcluster, "STRING result Array"=w428:string[], "S7 Connection out"=w425:T5)  [unwired: 2 in, 1 out]
            n117 = Build Array (concatenate)(w429, w428) -> (w435:string[])
            n118 = call-poly <vilib>:"read DB.vi"("error in (no error)"=w431, "items #"=u16 2 ("Items # [byte]"), "Data Block #"=w423, "S7 Connection in"=w425) -> ("error out"=w427:errorcluster, "DINT result array"=w426:i32[], "S7 Connection out"=w411:T5)  [unwired: 5 in]
            n119 = case shown="No Error" w427 {
              selector: w427 -> [w442 w447]
              tunnel: w426 -> [w446 _]
              tunnel: w435 -> [w444 _]
              tunnel: w436 -> [w440 _]
              tunnel: [w439 w447] -> w413
              frame No Error {
                w441 = enum16{"Read", "Write"}."Write" ("Enum")
                n120 = call "PADMINI_AUTO_CYCLE VALUE 40.vi"("Enum"=w441, "error in (no error)"=w442, "Input"=w440) -> ("error out"=w443:errorcluster)  [unwired: 7 in, 1 out]
                n121 = call "PADMINI_AUTO_BARCODE_STRING 40.vi"("Enum"=w441, "error in (no error)"=w443, "Input"=w444) -> ("error out"=w445:errorcluster)  [unwired: 7 in, 1 out]
                n122 = call "PADMINI_AUTO_CYCLE STATE 40.vi"("Enum"=w441, "error in (no error)"=w445, "Input"=w446) -> ("error out"=w439:errorcluster)  [unwired: 7 in, 1 out]
              }
              frame Error {
              }
            }
          }
          frame "Error" {
            w450 = PLC_Comm_State."Connect"  # Enum
            n123 = global write "Global 1.vi" "PLC3 error"(w449) -> ()
            n124 = call <vilib>:"Clear Errors.vi"("error in (no error)"=w449) -> ("error out"=w452:errorcluster)  [unwired: 5 in, 1 out]
          }
          frame "Disconnect" {
            w455 = PLC_Comm_State."Disconnect"  # Enum
            w458 = T5 {"TCP Connection Ref"=refnum, "IP address"="", "timeout ms"=5000, "Connected?"=FALSE, "PLC Type"=enum."S7 1200", "Rack S7 400"=0, "Slot S7 400"=0, "PDU Size"=0, "connection semaphore"=refnum}  # S7 Connection out
            n125 = call <vilib>:"Clear Errors.vi"("error in (no error)"=w459) -> ("error out"=w462:errorcluster)  [unwired: 5 in, 1 out]
            n126 = call <vilib>:"disconnect.vi"("error in (no error)"=w462, "S7 Connection in"=w460) -> ("error out"=w461:errorcluster)  [unwired: 8 in, 1 out]
          }
          frame "Write2" {
            # "No Use"
          }
          frame "Write3" {
            # "No Use"
          }
          frame "Read2" {
            # "No Use"
          }
          frame "Read3" {
            # "No Use"
          }
        }
        n127 = Wait (ms)(milliseconds to wait=w292) -> ()  [unwired: 1 out]
        n128 = call "PADMINI_STOP_ALL.vi"("Enum"=enum16{"Read", "Write"}."Read") -> ("Boolean 2"=w283:bool)  [unwired: 9 in, 1 out]
        n129 = local read "stop"() -> (w282:bool)
        n130 = case shown="Error" w297 {
          selector: w297 -> [w301 w308]
          tunnel: [w301 w307] -> w277
          tunnel: [w300 w306] -> w286
          tunnel: w291 -> [w300 _]
          tunnel: [w299 w312] -> w290
          tunnel: w289 -> [w299 w312]
          tunnel: w285 -> [_ w311]
          tunnel: [w298 TRUE] -> w276
          tunnel: w275 -> [w298 _]
          frame No Error {
          }
          frame Error {
            w306 = PLC_Comm_State."Error"  # Enum
            w303 = "    " ("string")
            n131 = Unbundle By Name(w308) -> ("source"=w304:string)
            n132 = Get Date/Time String() -> (time string=w302:string)  [unwired: 3 in, 1 out]
            n133 = call <userlib>:"Get Strings from Enum__ogtk.vi"("Enum"=w311) -> ("String Value"=w310:string)  [unwired: 7 in, 3 out]
            n134 = Concatenate Strings(w310, w303, w302, w303, w304) -> (w309:string)
            n135 = Bundle By Name(cluster=w308, "source"=w309) -> (w307:errorcluster)
          }
        }
        n136 = Or(x=w282, y=w283) -> (x .or. y?=w280:bool)
        n137 = Select(t=w284, s=w280, f=w286) -> (s? t:f=w287:T1)
        n138 = Unbundle By Name(w277) -> ("status"=w279:bool)
        n139 = Not(x=w279) -> (.not. x?=w278:bool)
        n140 = global write "Global 1.vi" "PLC 3"(w278) -> ()
      }
    }
  }
  n141 = disable-structure shown="Enabled" {
    disable-tunnel: w10 -> [w484 w590]
    disable-tunnel: w9 -> [w482 w591]
    disable-tunnel: [w478 w589] -> w8
    frame Disabled {
      w475 = TRUE  # Use Rack/Slot for S71200/1500
      w476 = u8 1  # Slot S7 300/400
      w477 = u8 0  # Rack S7 300/400
      w483 = u16[] [7]  # Data Block #
      n142 = call <vilib>:"connect.vi"("Use Rack/Slot for S71200/1500"=w475, "Slot S7 300/400"=w476, "PLC Type"=PLC_Type."S7 1200" ("PLC Type 2"), "error in (no error)"=w484, "Rack S7 300/400"=w477, "timeout [ms]"=1000 ("timeout [ms] 2"), "IP address"=w482) -> ("error out"=w486:errorcluster, "S7 Connection out"=w485:T5)  [unwired: 3 in]
      n143 = for {
        tunnel: w483 -> [w496] mode=indexing
        shift-right: [w494] -> w489
        shift-left: w485 -> [w491]
        tunnel: w486 -> [w492]
        tunnel: [w493] -> w490
        w495 = i32[] [0, 0]  # DINT input array
        # "Reset Search and save \nbit on software start"
        n144 = call-poly <vilib>:"write DB.vi"("DINT input array"=w495, "error in (no error)"=w492, "Data Block #"=w496, "S7 Connection in"=w491) -> ("error out"=w493:errorcluster, "S7 Connection out"=w494:T5)  [unwired: 4 in, 2 out]
      }
      "error out 4" <- w490
      n145 = while {
        shift-right: [w499] -> w479
        shift-left: w489 -> [w509]
        shift-right: [w507] -> w480
        shift-left: w490 -> [w508]
        tunnel: w482 -> [w498]
        stop <- w501 stop-if-true
        # "OP 110"
        n146 = flat-sequence {
          tunnel: [w513] -> w505
          tunnel: [w514] -> w500
          tunnel: w508 -> [w532]
          tunnel: w509 -> [w533]
          tunnel: w498 -> [w534]
          tunnel: [w534] -> w497
          tunnel: [w561] -> w507
          tunnel: [w560] -> w499
          tunnel: w505 -> [w563]
          tunnel: w500 -> [w562]
          tunnel: w497 -> [w559]
          frame #0 {
            # "AUTO WRITE"
            n147 = global read "DATA LOG.vi" "OP 110 Outputs"() -> (w531:bool)
            n148 = case shown="True" w531 {
              tunnel: [w544 w549] -> w523
              tunnel: [w545 w550] -> w522
              tunnel: w532 -> [w544 w554]
              tunnel: w533 -> [w545 w553]
              frame False {
              }
              frame True {
                w546 = i32[] [0, 0]  # DINT input array
                w547 = u16 7  # Data Block #
                n149 = call "PADMINI_AUTO_BARCODE_STATUS 110.vi"("Enum"=enum16{"Read", "Write"}."Read", "error in (no error)"=w554) -> ("error out"=w556:errorcluster, "O/P"=w557:i32[])  [unwired: 8 in]
                n150 = call-poly <vilib>:"write DB.vi"("Item offset [byte]"=u32 8, "DINT input array"=w557, "error in (no error)"=w556, "Data Block #"=w547, "S7 Connection in"=w553) -> ("error out"=w548:errorcluster, "S7 Connection out"=w551:T5)  [unwired: 3 in, 2 out]
                n151 = global write "DATA LOG.vi" "OP 110 Outputs"(FALSE) -> ()
                n152 = call-poly <vilib>:"write DB.vi"("DINT input array"=w546, "error in (no error)"=w548, "Data Block #"=w547, "S7 Connection in"=w551) -> ("error out"=w549:errorcluster, "S7 Connection out"=w550:T5)  [unwired: 4 in, 2 out]
              }
            }
            n153 = global read "DATA LOG.vi" "OP 110 reset"() -> (w520:bool)
            n154 = case shown="True" w520 {
              tunnel: w523 -> [w535 w543]
              tunnel: [w535 w542] -> w524
              tunnel: w522 -> [w536 w541]
              tunnel: [w536 w540] -> w521
              frame False {
              }
              frame True {
                n155 = global write "DATA LOG.vi" "OP 110 reset"(FALSE) -> ()
                n156 = call-poly <vilib>:"write DB.vi"("DINT input array"=i32[] [0, 0], "error in (no error)"=w543, "Data Block #"=u16 7, "S7 Connection in"=w541) -> ("error out"=w542:errorcluster, "S7 Connection out"=w540:T5)  [unwired: 4 in, 2 out]
              }
            }
            "error out 3" <- w524
            n157 = call-poly <vilib>:"read DB.vi"("Item offset [byte]"=u32 20, "String length reserved in DB (default=254)"=u16 50, "error in (no error)"=w524, "items #"=u16 3 ("Items # [byte]"), "Data Block #"=u16 7, "S7 Connection in"=w521) -> ("error out"=w526:errorcluster, "STRING result Array"=w527:string[], "S7 Connection out"=w512:T5)  [unwired: 2 in, 1 out]
            n158 = call "PADMINI_AUTO_BARCODE_STRING 110.vi"("Enum"=enum16{"Read", "Write"}."Write", "error in (no error)"=w526, "Input"=w527) -> ("error out"=w515:errorcluster)  [unwired: 7 in, 1 out]
            n159 = call-poly <vilib>:"read DB.vi"("error in (no error)"=w515, "items #"=u16 2 ("Items # [byte]"), "Data Block #"=u16 7, "S7 Connection in"=w512) -> ("error out"=w519:errorcluster, "DINT result array"=w518:i32[], "S7 Connection out"=w513:T5)  [unwired: 5 in]
            n160 = call "PADMINI_AUTO_CYCLE STATE 110.vi"("Enum"=enum16{"Read", "Write"}."Write", "error in (no error)"=w519, "Input"=w518) -> ("error out"=w514:errorcluster)  [unwired: 7 in, 1 out]
          }
          frame #1 {
            # "RECONNECT"
            n161 = case shown="Error" w562 {
              selector: w562 -> [w567 w568]
              tunnel: [w566 w572] -> w560
              tunnel: [w567 w573] -> w561
              tunnel: w563 -> [w566 w571]
              tunnel: w559 -> [_ w570]
              frame No Error {
              }
              frame Error {
                n162 = Unbundle By Name(w568) -> ("code"=w569:i32)
                n163 = call <vilib>:"Clear Errors.vi"("error in (no error)"=w568) -> ("error out"=w574:errorcluster)  [unwired: 5 in, 1 out]
                n164 = case shown="0, Default" w569 {
                  tunnel: w574 -> [w576 w587]
                  tunnel: [w576 w585] -> w573
                  tunnel: [w577 w584] -> w572
                  tunnel: w571 -> [w577 w581]
                  tunnel: w570 -> [_ w580]
                  tunnel: w568 -> [w575 _]
                  frame 0, Default {
                    n165 = global write "Global 1.vi" "PLC8 error"(w575) -> ()
                  }
                  frame 1, 66 {
                    w579 = u8 1  # Slot S7 300/400
                    n166 = call <vilib>:"disconnect.vi"("error in (no error)"=w587, "S7 Connection in"=w581) -> ("error out"=w586:errorcluster)  [unwired: 8 in, 1 out]
                    n167 = call <vilib>:"Clear Errors.vi"("error in (no error)"=w586) -> ("error out"=w583:errorcluster)  [unwired: 5 in, 1 out]
                    n168 = call <vilib>:"connect.vi"("Use Rack/Slot for S71200/1500"=TRUE, "Slot S7 300/400"=w579, "PLC Type"=PLC_Type."S7 1200" ("PLC Type 2"), "error in (no error)"=w583, "IP address"=w580) -> ("error out"=w585:errorcluster, "S7 Connection out"=w584:T5)  [unwired: 5 in]
                  }
                }
              }
            }
            n169 = Unbundle By Name(w562) -> ("status"=w565:bool)
            n170 = Not(x=w565) -> (.not. x?=w564:bool)
            "PLC 8" <- w564
            n171 = global write "Global 1.vi" "PLC 8"(w564) -> ()
          }
        }
        n172 = call "PADMINI_STOP_ALL.vi"("Enum"=enum16{"Read", "Write"}."Read") -> ("Boolean 2"=w503:bool)  [unwired: 9 in, 1 out]
        n173 = local read "stop"() -> (w502:bool)
        n174 = Or(x=w502, y=w503) -> (x .or. y?=w501:bool)
        n175 = Wait (ms)(milliseconds to wait=u32 1200) -> ()  [unwired: 1 out]
      }
      n176 = call <vilib>:"Clear Errors.vi"("error in (no error)"=w480) -> ("error out"=w481:errorcluster)  [unwired: 5 in, 1 out]
      n177 = call <vilib>:"disconnect.vi"("error in (no error)"=w481, "S7 Connection in"=w479) -> ("error out"=w478:errorcluster)  [unwired: 8 in, 1 out]
    }
    frame Enabled {
      w592 = PLC_Comm_State."Int"  # Enum
      n178 = while {
        shift-right: [w607] -> _
        shift-left: w592 -> [w615]
        shift-right: [w599] -> w589
        shift-left: w590 -> [w614]
        shift-right: [w610] -> _
        shift-left: _ -> [w613]
        tunnel: w591 -> [w596]
        shift-right: [w595] -> _
        shift-left: FALSE -> [w593]
        stop <- w608 stop-if-true
        w604 = PLC_Comm_State."Disconnect"  # Enum
        w612 = u32 800  # milliseconds to wait
        # "Int-->Write-->Read---if--Error-->reconnect\n               ^------v                                       v\n                ^------------------------------v"
        # "OP 110"
        n179 = case shown="\"Write\"" w615 {
          selector: w615 -> [w634 w652 w679 w721 w732 w737 _ _ _ _]
          tunnel: [w639 w654 w672 w707 w733 w742 w745 w749 w752 w755] -> w616
          tunnel: [w640 w653 w673 w708 w734 w739 w746 w748 w751 w754] -> w609
          tunnel: w614 -> [w637 w648 w670 w705 w730 w740 w745 w749 w752 w755]
          tunnel: w613 -> [w635 _ w671 w706 w734 w741 w746 w748 w751 w754]
          tunnel: [w633 w651 w678 w720 w731 w736 _ _ _ _] -> w611
          tunnel: [_ _ _ _ _ TRUE _ _ _ _] -> w608
          tunnel: [w634 w652 w679 w721 w732 w737 _ _ _ _] -> w605
          tunnel: w596 -> [w632 w650 _ _ _ _ _ _ _ _]
          tunnel: [w631 w646 w669 w704 w729 w735 w744 w747 w750 w753] -> w594
          tunnel: w593 -> [w631 w646 w669 w704 w729 w735 w744 w747 w750 w753]
          frame "Connect" {
            w633 = PLC_Comm_State."Write"  # Enum
            w645 = TRUE  # Use Rack/Slot for S71200/1500
            w644 = u8 1  # Slot S7 300/400
            w642 = u8 0  # Rack S7 300/400
            # "Reconect"
            n180 = call <vilib>:"disconnect.vi"("error in (no error)"=w637, "S7 Connection in"=w635) -> ("error out"=w638:errorcluster)  [unwired: 8 in, 1 out]
            n181 = call <vilib>:"Clear Errors.vi"("error in (no error)"=w638) -> ("error out"=w636:errorcluster)  [unwired: 5 in, 1 out]
            n182 = call <vilib>:"connect.vi"("Use Rack/Slot for S71200/1500"=w645, "Slot S7 300/400"=w644, "PLC Type"=PLC_Type."S7 1200" ("PLC Type 2"), "error in (no error)"=w636, "Rack S7 300/400"=w642, "timeout [ms]"=1000 ("timeout [ms] 2"), "IP address"=w632) -> ("error out"=w639:errorcluster, "S7 Connection out"=w640:T5)  [unwired: 3 in]
          }
          frame "Int" {
            w651 = PLC_Comm_State."Write"  # Enum
            w655 = TRUE  # Use Rack/Slot for S71200/1500
            w656 = u8 1  # Slot S7 300/400
            w657 = u8 0  # Rack S7 300/400
            w658 = u16[] [7]  # Data Block #
            # "Initialize and set first bits"
            n183 = call "Stall Data Flow.vim"("value in"=w648, "milliseconds to wait"=u32 903) -> ("value out"=w647:errorcluster)  [unwired: 1 out]
            n184 = call <vilib>:"connect.vi"("Use Rack/Slot for S71200/1500"=w655, "Slot S7 300/400"=w656, "PLC Type"=PLC_Type."S7 1200" ("PLC Type 2"), "error in (no error)"=w647, "Rack S7 300/400"=w657, "timeout [ms]"=1000 ("timeout [ms] 2"), "IP address"=w650) -> ("error out"=w660:errorcluster, "S7 Connection out"=w659:T5)  [unwired: 3 in]
            n185 = for {
              tunnel: w658 -> [w668] mode=indexing
              shift-right: [w666] -> w653
              shift-left: w659 -> [w664]
              tunnel: w660 -> [w665]
              tunnel: [w663] -> w654
              w667 = i32[] [0, 0]  # DINT input array
              # "Reset Search and save \nbit on software start"
              n186 = call-poly <vilib>:"write DB.vi"("DINT input array"=w667, "error in (no error)"=w665, "Data Block #"=w668, "S7 Connection in"=w664) -> ("error out"=w663:errorcluster, "S7 Connection out"=w666:T5)  [unwired: 4 in, 2 out]
            }
          }
          frame "Write" {
            w678 = PLC_Comm_State."Read"  # Enum
            n187 = global read "DATA LOG.vi" "OP 110 Outputs"() -> (w677:bool)
            n188 = case shown="True" w677 {
              tunnel: [w689 w694] -> w676
              tunnel: [w690 w698] -> w675
              tunnel: w671 -> [w690 w692]
              tunnel: w670 -> [w689 w691]
              frame False {
              }
              frame True {
                w695 = i32[] [0, 0]  # DINT input array
                w696 = u16 7  # Data Block #
                n189 = call "PADMINI_AUTO_BARCODE_STATUS 110.vi"("Enum"=enum16{"Read", "Write"}."Read", "error in (no error)"=w691) -> ("error out"=w701:errorcluster, "O/P"=w702:i32[])  [unwired: 8 in]
                n190 = call-poly <vilib>:"write DB.vi"("Item offset [byte]"=u32 8, "DINT input array"=w702, "error in (no error)"=w701, "Data Block #"=w696, "S7 Connection in"=w692) -> ("error out"=w697:errorcluster, "S7 Connection out"=w699:T5)  [unwired: 3 in, 2 out]
                n191 = call-poly <vilib>:"write DB.vi"("DINT input array"=w695, "error in (no error)"=w697, "Data Block #"=w696, "S7 Connection in"=w699) -> ("error out"=w694:errorcluster, "S7 Connection out"=w698:T5)  [unwired: 4 in, 2 out]
                n192 = Unbundle By Name(w694) -> ("status"=w693:bool)
                n193 = global write "DATA LOG.vi" "OP 110 Outputs"(w693) -> ()
              }
            }
            n194 = global read "DATA LOG.vi" "OP 110 reset"() -> (w674:bool)
            n195 = case shown="True" w674 {
              tunnel: w676 -> [w680 w688]
              tunnel: [w680 w683] -> w672
              tunnel: w675 -> [w681 w687]
              tunnel: [w681 w686] -> w673
              frame False {
              }
              frame True {
                n196 = call-poly <vilib>:"write DB.vi"("DINT input array"=i32[] [0, 0], "error in (no error)"=w688, "Data Block #"=u16 7, "S7 Connection in"=w687) -> ("error out"=w683:errorcluster, "S7 Connection out"=w686:T5)  [unwired: 4 in, 2 out]
                n197 = Unbundle By Name(w683) -> ("status"=w682:bool)
                n198 = global write "DATA LOG.vi" "OP 110 reset"(w682) -> ()
              }
            }
          }
          frame "Read" {
            w720 = PLC_Comm_State."Write"  # Enum
            n199 = call-poly <vilib>:"read DB.vi"("Item offset [byte]"=u32 20, "String length reserved in DB (default=254)"=u16 50, "error in (no error)"=w705, "items #"=u16 3 ("Items # [byte]"), "Data Block #"=u16 7, "S7 Connection in"=w706) -> ("error out"=w718:errorcluster, "STRING result Array"=w719:string[], "S7 Connection out"=w715:T5)  [unwired: 2 in, 1 out]
            n200 = call-poly <vilib>:"read DB.vi"("error in (no error)"=w718, "items #"=u16 2 ("Items # [byte]"), "Data Block #"=u16 7, "S7 Connection in"=w715) -> ("error out"=w717:errorcluster, "DINT result array"=w716:i32[], "S7 Connection out"=w708:T5)  [unwired: 5 in]
            n201 = case shown="No Error" w717 {
              selector: w717 -> [w726 w728]
              tunnel: w716 -> [w727 _]
              tunnel: w719 -> [w723 _]
              tunnel: [w722 w728] -> w707
              frame No Error {
                w724 = enum16{"Read", "Write"}."Write" ("Enum")
                n202 = call "PADMINI_AUTO_BARCODE_STRING 110.vi"("Enum"=w724, "error in (no error)"=w726, "Input"=w723) -> ("error out"=w725:errorcluster)  [unwired: 7 in, 1 out]
                n203 = call "PADMINI_AUTO_CYCLE STATE 110.vi"("Enum"=w724, "error in (no error)"=w725, "Input"=w727) -> ("error out"=w722:errorcluster)  [unwired: 7 in, 1 out]
              }
              frame Error {
              }
            }
          }
          frame "Error" {
            w731 = PLC_Comm_State."Connect"  # Enum
            n204 = global write "Global 1.vi" "PLC8 error"(w730) -> ()
            n205 = call <vilib>:"Clear Errors.vi"("error in (no error)"=w730) -> ("error out"=w733:errorcluster)  [unwired: 5 in, 1 out]
          }
          frame "Disconnect" {
            w736 = PLC_Comm_State."Disconnect"  # Enum
            w739 = T5 {"TCP Connection Ref"=refnum, "IP address"="", "timeout ms"=5000, "Connected?"=FALSE, "PLC Type"=enum."S7 1200", "Rack S7 400"=0, "Slot S7 400"=0, "PDU Size"=0, "connection semaphore"=refnum}  # S7 Connection out
            n206 = call <vilib>:"Clear Errors.vi"("error in (no error)"=w740) -> ("error out"=w743:errorcluster)  [unwired: 5 in, 1 out]
            n207 = call <vilib>:"disconnect.vi"("error in (no error)"=w743, "S7 Connection in"=w741) -> ("error out"=w742:errorcluster)  [unwired: 8 in, 1 out]
          }
          frame "Write2" {
            # "No Use"
          }
          frame "Write3" {
            # "No Use"
          }
          frame "Read2" {
            # "No Use"
          }
          frame "Read3" {
            # "No Use"
          }
        }
        n208 = Wait (ms)(milliseconds to wait=w612) -> ()  [unwired: 1 out]
        n209 = call "PADMINI_STOP_ALL.vi"("Enum"=enum16{"Read", "Write"}."Read") -> ("Boolean 2"=w603:bool)  [unwired: 9 in, 1 out]
        n210 = local read "stop"() -> (w598:bool)
        n211 = case shown="Error" w616 {
          selector: w616 -> [w620 w624]
          tunnel: [w620 w623] -> w599
          tunnel: [w619 w622] -> w606
          tunnel: w611 -> [w619 _]
          tunnel: [w618 w630] -> w610
          tunnel: w609 -> [w618 w630]
          tunnel: w605 -> [_ w628]
          tunnel: [w617 TRUE] -> w595
          tunnel: w594 -> [w617 _]
          frame No Error {
          }
          frame Error {
            w622 = PLC_Comm_State."Error"  # Enum
            n212 = Unbundle By Name(w624) -> ("source"=w629:string)
            n213 = call <userlib>:"Get Strings from Enum__ogtk.vi"("Enum"=w628) -> ("String Value"=w627:string)  [unwired: 7 in, 3 out]
            n214 = Concatenate Strings(w627, "    " ("string"), w629) -> (w625:string)
            n215 = Bundle By Name(cluster=w624, "source"=w625) -> (w623:errorcluster)
          }
        }
        n216 = Or(x=w598, y=w603) -> (x .or. y?=w601:bool)
        n217 = Select(t=w604, s=w601, f=w606) -> (s? t:f=w607:T1)
        n218 = Unbundle By Name(w599) -> ("status"=w600:bool)
        n219 = Not(x=w600) -> (.not. x?=w597:bool)
        n220 = global write "Global 1.vi" "PLC 8"(w597) -> ()
      }
    }
  }
  n221 = disable-structure shown="Enabled" {
    disable-tunnel: w31 -> [w767 w982]
    disable-tunnel: w10 -> [w761 w981]
    disable-tunnel: [w756 w979] -> w6
    frame Disabled {
      w758 = TRUE  # Use Rack/Slot for S71200/1500
      w759 = u8 1  # Slot S7 300/400
      w760 = u8 0  # Rack S7 300/400
      n222 = call <vilib>:"connect.vi"("Use Rack/Slot for S71200/1500"=w758, "Slot S7 300/400"=w759, "PLC Type"=PLC_Type."S7 1200" ("PLC Type 2"), "error in (no error)"=w761, "Rack S7 300/400"=w760, "timeout [ms]"=1000 ("timeout [ms] 2"), "IP address"=w767) -> ("error out"=w762:errorcluster, "S7 Connection out"=w763:T5)  [unwired: 3 in]
      n223 = for {
        tunnel: u16[] [80, 82] ("Data Block #") -> [w777] mode=indexing
        shift-right: [w775] -> w764
        shift-left: w763 -> [w772]
        tunnel: w762 -> [w773]
        tunnel: [w774] -> w765
        w776 = i32[] [0, 0]  # DINT input array
        # "Reset Search and save \nbit on software start"
        n224 = call-poly <vilib>:"write DB.vi"("DINT input array"=w776, "error in (no error)"=w773, "Data Block #"=w777, "S7 Connection in"=w772) -> ("error out"=w774:errorcluster, "S7 Connection out"=w775:T5)  [unwired: 4 in, 2 out]
      }
      n225 = while {
        shift-right: [w780] -> w768
        shift-left: w764 -> [w790]
        shift-right: [w788] -> w769
        shift-left: w765 -> [w789]
        tunnel: w767 -> [w779]
        stop <- w782 stop-if-true
        # "OP 70 - 80"
        n226 = flat-sequence {
          tunnel: [w792] -> w786
          tunnel: [w796] -> w781
          tunnel: w789 -> [w898]
          tunnel: w790 -> [w897]
          tunnel: w779 -> [w885]
          tunnel: [w885] -> w778
          tunnel: [w951] -> w788
          tunnel: [w950] -> w780
          tunnel: w786 -> [w953]
          tunnel: w781 -> [w952]
          tunnel: w778 -> [w949]
          frame #0 {
            w817 = u32 500  # milliseconds to wait
            w844 = u16 83 ("Data Block #")
            w867 = u16 81 ("Data Block #")
            w828 = u16 82 ("Data Block #")
            w804 = u16 80 ("Data Block #")
            # "AUTO WRITE"
            n227 = global read "DATA LOG.vi" "OP 70 Outputs"() -> (w896:bool)
            n228 = case shown="True" w896 {
              tunnel: w897 -> [w934 w947]
              tunnel: [w935 w938] -> w872
              tunnel: [w934 w939] -> w871
              tunnel: w898 -> [w935 w944]
              frame False {
              }
              frame True {
                w948 = u16 81  # Data Block #
                n229 = call "PADMINI_AUTO_BARCODE_STATUS 70.vi"("Enum"=enum16{"Read", "Write"}."Read", "error in (no error)"=w944) -> ("error out"=w943:errorcluster, "O/P"=w945:i32[])  [unwired: 8 in]
                n230 = global write "DATA LOG.vi" "OP 70 Outputs"(FALSE) -> ()
                n231 = call-poly <vilib>:"write DB.vi"("DINT input array"=w945, "error in (no error)"=w943, "Data Block #"=w948, "S7 Connection in"=w947) -> ("error out"=w936:errorcluster, "S7 Connection out"=w937:T5)  [unwired: 4 in, 2 out]
                n232 = call-poly <vilib>:"write DB.vi"("DINT input array"=i32[] [0] ("Data Byte"), "error in (no error)"=w936, "Data Block #"=u16 80, "S7 Connection in"=w937) -> ("error out"=w938:errorcluster, "S7 Connection out"=w939:T5)  [unwired: 4 in, 2 out]
              }
            }
            n233 = global read "DATA LOG.vi" "OP 70 reset"() -> (w873:bool)
            n234 = global read "DATA LOG.vi" "Auto Cycle On"() -> (w821:bool)
            n235 = case shown="True" w873 {
              tunnel: w872 -> [w909 w918]
              tunnel: [w909 w917] -> w862
              tunnel: w871 -> [w910 w916]
              tunnel: [w910 w915] -> w863
              frame False {
              }
              frame True {
                n236 = global write "DATA LOG.vi" "OP 70 reset"(FALSE) -> ()
                n237 = call-poly <vilib>:"write DB.vi"("Item offset [byte]"=u16 4 ("Data Block #"), "DINT input array"=i32[] [0], "error in (no error)"=w918, "Data Block #"=u16 80, "S7 Connection in"=w916) -> ("error out"=w917:errorcluster, "S7 Connection out"=w915:T5)  [unwired: 3 in, 2 out]
              }
            }
            n238 = Boolean To (0,1)(Boolean=w821) -> (0, 1=w820:i16)
            n239 = Build Array(w820) -> (w819:i16[])
            n240 = call "Stall Data Flow.vim"("value in"=w862, "milliseconds to wait"=w817) -> ("value out"=w818:errorcluster)  [unwired: 1 out]
            n241 = global read "Global 1.vi" "Filtered BARCODE selected"() -> (w864:string[])
            n242 = call-poly <vilib>:"write DB.vi"("Item offset [byte]"=u32 20, "DINT input array"=w819, "error in (no error)"=w818, "Data Block #"=w867, "S7 Connection in"=w863) -> ("error out"=w869:errorcluster, "S7 Connection out"=w870:T5)  [unwired: 3 in, 2 out]
            n243 = call-poly <vilib>:"write DB.vi"("Item offset [byte]"=u32 24, "Input STRINGS"=w864, "error in (no error)"=w869, "String length reserved in DB (default=254)"=u16 15, "Data Block #"=w867, "S7 Connection in"=w870) -> ("error out"=w860:errorcluster, "S7 Connection out"=w861:T5)  [unwired: 2 in, 2 out]
            n244 = call "Stall Data Flow.vim"("value in"=w860, "milliseconds to wait"=u32 300) -> ("value out"=w816:errorcluster)  [unwired: 1 out]
            n245 = call-poly <vilib>:"read DB.vi"("Item offset [byte]"=u32 8, "error in (no error)"=w816, "items #"=u16 2 ("Items # [byte]"), "Data Block #"=w804, "S7 Connection in"=w861) -> ("error out"=w888:errorcluster, "REAL result array"=w886:sgl[], "S7 Connection out"=w894:T5)  [unwired: 4 in]
            n246 = call "PADMINI_AUTO_CYCLE VALUE 70.vi"("Enum"=enum16{"Read", "Write"}."Write", "error in (no error)"=w888, "Input"=w886) -> ("error out"=w887:errorcluster)  [unwired: 7 in, 1 out]
            n247 = call "Stall Data Flow.vim"("value in"=w887, "milliseconds to wait"=u32 0) -> ("value out"=w814:errorcluster)  [unwired: 1 out]
            n248 = call-poly <vilib>:"read DB.vi"("Item offset [byte]"=u32 16, "String length reserved in DB (default=254)"=u16 50, "error in (no error)"=w814, "items #"=u16 1 ("Items # [byte]"), "Data Block #"=w804, "S7 Connection in"=w894) -> ("error out"=w853:errorcluster, "STRING result Array"=w852:string[], "S7 Connection out"=w854:T5)  [unwired: 2 in, 1 out]
            n249 = call-poly <vilib>:"read DB.vi"("Item offset [byte]"=u32 68, "String length reserved in DB (default=254)"=u16 10, "error in (no error)"=w853, "items #"=u16 1 ("Items # [byte]"), "Data Block #"=w804, "S7 Connection in"=w854) -> ("error out"=w855:errorcluster, "STRING result Array"=w856:string[], "S7 Connection out"=w803:T5)  [unwired: 2 in, 1 out]
            n250 = Build Array (concatenate)(w852, w856) -> (w850:string[])
            n251 = call "PADMINI_AUTO_BARCODE_STRING 70.vi"("Enum"=enum16{"Read", "Write"}."Write", "error in (no error)"=w855, "Input"=w850) -> ("error out"=w801:errorcluster)  [unwired: 7 in, 1 out]
            n252 = call-poly <vilib>:"read DB.vi"("error in (no error)"=w801, "items #"=u16 2 ("Items # [byte]"), "Data Block #"=w804, "S7 Connection in"=w803) -> ("error out"=w806:errorcluster, "DINT result array"=w808:i32[], "S7 Connection out"=w802:T5)  [unwired: 5 in]
            n253 = call "PADMINI_AUTO_CYCLE STATE 70.vi"("Enum"=enum16{"Read", "Write"}."Write", "error in (no error)"=w806, "Input"=w808) -> ("error out"=w791:errorcluster)  [unwired: 7 in, 1 out]
            n254 = global read "DATA LOG.vi" "OP 80 Outputs"() -> (w874:bool)
            n255 = case shown="True" w874 {
              tunnel: [w920 w923] -> w849
              tunnel: [w919 w924] -> w826
              tunnel: w791 -> [w920 w930]
              tunnel: w802 -> [w919 w927]
              frame False {
              }
              frame True {
                w933 = u16 83  # Data Block #
                n256 = call "PADMINI_AUTO_BARCODE_STATUS 80.vi"("Enum"=enum16{"Read", "Write"}."Read", "error in (no error)"=w930) -> ("error out"=w929:errorcluster, "O/P"=w931:i32[])  [unwired: 8 in]
                n257 = global write "DATA LOG.vi" "OP 80 Outputs"(FALSE) -> ()
                n258 = call-poly <vilib>:"write DB.vi"("DINT input array"=w931, "error in (no error)"=w929, "Data Block #"=w933, "S7 Connection in"=w927) -> ("error out"=w921:errorcluster, "S7 Connection out"=w922:T5)  [unwired: 4 in, 2 out]
                n259 = call-poly <vilib>:"write DB.vi"("DINT input array"=i32[] [0] ("Data Byte"), "error in (no error)"=w921, "Data Block #"=u16 82, "S7 Connection in"=w922) -> ("error out"=w923:errorcluster, "S7 Connection out"=w924:T5)  [unwired: 4 in, 2 out]
              }
            }
            n260 = global read "DATA LOG.vi" "OP 80 reset"() -> (w848:bool)
            n261 = global read "DATA LOG.vi" "Auto Cycle On"() -> (w824:bool)
            n262 = case shown="True" w848 {
              tunnel: w849 -> [w900 w908]
              tunnel: [w900 w903] -> _
              tunnel: [w900 w903] -> w838
              tunnel: w826 -> [w899 w902]
              tunnel: [w899 w901] -> w825
              frame False {
              }
              frame True {
                n263 = global write "DATA LOG.vi" "OP 80 reset"(FALSE) -> ()
                n264 = call-poly <vilib>:"write DB.vi"("Item offset [byte]"=u16 4 ("Data Block #"), "DINT input array"=i32[] [0], "error in (no error)"=w908, "Data Block #"=u16 82, "S7 Connection in"=w902) -> ("error out"=w903:errorcluster, "S7 Connection out"=w901:T5)  [unwired: 3 in, 2 out]
              }
            }
            n265 = Boolean To (0,1)(Boolean=w824) -> (0, 1=w823:i16)
            n266 = Build Array(w823) -> (w822:i16[])
            n267 = global read "Global 1.vi" "Filtered BARCODE selected"() -> (w841:string[])
            n268 = call-poly <vilib>:"write DB.vi"("Item offset [byte]"=u32 20, "DINT input array"=w822, "error in (no error)"=w838, "Data Block #"=w844, "S7 Connection in"=w825) -> ("error out"=w846:errorcluster, "S7 Connection out"=w847:T5)  [unwired: 3 in, 2 out]
            n269 = call-poly <vilib>:"write DB.vi"("Item offset [byte]"=u32 24, "Input STRINGS"=w841, "error in (no error)"=w846, "String length reserved in DB (default=254)"=u16 15, "Data Block #"=w844, "S7 Connection in"=w847) -> ("error out"=w839:errorcluster, "S7 Connection out"=w840:T5)  [unwired: 2 in, 2 out]
            n270 = call-poly <vilib>:"read DB.vi"("Item offset [byte]"=u32 8, "error in (no error)"=w839, "items #"=u16 1 ("Items # [byte]"), "Data Block #"=w828, "S7 Connection in"=w840) -> ("error out"=w882:errorcluster, "REAL result array"=w884:sgl[], "S7 Connection out"=w876:T5)  [unwired: 4 in]
            n271 = call "PADMINI_AUTO_CYCLE VALUE 80.vi"("Enum"=enum16{"Read", "Write"}."Write", "error in (no error)"=w882, "Input"=w884) -> ("error out"=w883:errorcluster)  [unwired: 7 in, 1 out]
            n272 = call "Stall Data Flow.vim"("value in"=w883, "milliseconds to wait"=u32 300) -> ("value out"=w812:errorcluster)  [unwired: 1 out]
            n273 = call-poly <vilib>:"read DB.vi"("Item offset [byte]"=u32 12, "String length reserved in DB (default=254)"=u16 50, "error in (no error)"=w812, "items #"=u16 1 ("Items # [byte]"), "Data Block #"=w828, "S7 Connection in"=w876) -> ("error out"=w833:errorcluster, "STRING result Array"=w831:string[], "S7 Connection out"=w829:T5)  [unwired: 2 in, 1 out]
            n274 = call "Stall Data Flow.vim"("value in"=w833, "milliseconds to wait"=u32 300) -> ("value out"=w810:errorcluster)  [unwired: 1 out]
            n275 = call-poly <vilib>:"read DB.vi"("Item offset [byte]"=u32 64, "String length reserved in DB (default=254)"=u16 10, "error in (no error)"=w810, "items #"=u16 2 ("Items # [byte]"), "Data Block #"=w828, "S7 Connection in"=w829) -> ("error out"=w832:errorcluster, "STRING result Array"=w837:string[], "S7 Connection out"=w793:T5)  [unwired: 2 in, 1 out]
            n276 = Build Array (concatenate)(w831, w837) -> (w830:string[])
            n277 = call "PADMINI_AUTO_BARCODE_STRING 80.vi"("Enum"=enum16{"Read", "Write"}."Write", "error in (no error)"=w832, "Input"=w830) -> ("error out"=w795:errorcluster)  [unwired: 7 in, 1 out]
            n278 = call-poly <vilib>:"read DB.vi"("error in (no error)"=w795, "items #"=u16 2 ("Items # [byte]"), "Data Block #"=u16 82, "S7 Connection in"=w793) -> ("error out"=w799:errorcluster, "DINT result array"=w797:i32[], "S7 Connection out"=w792:T5)  [unwired: 5 in]
            n279 = call "PADMINI_AUTO_CYCLE STATE 80.vi"("Enum"=enum16{"Read", "Write"}."Write", "error in (no error)"=w799, "Input"=w797) -> ("error out"=w796:errorcluster)  [unwired: 7 in, 1 out]
          }
          frame #1 {
            # "RECONNECT"
            n280 = case shown="Error" w952 {
              selector: w952 -> [w957 w958]
              tunnel: [w956 w962] -> w950
              tunnel: [w957 w963] -> w951
              tunnel: w953 -> [w956 w961]
              tunnel: w949 -> [_ w960]
              frame No Error {
              }
              frame Error {
                n281 = Unbundle By Name(w958) -> ("code"=w959:i32)
                n282 = call <vilib>:"Clear Errors.vi"("error in (no error)"=w958) -> ("error out"=w964:errorcluster)  [unwired: 5 in, 1 out]
                n283 = case shown="1, 66" w959 {
                  tunnel: w964 -> [w966 w977]
                  tunnel: [w966 w975] -> w963
                  tunnel: [w967 w974] -> w962
                  tunnel: w961 -> [w967 w971]
                  tunnel: w960 -> [_ w970]
                  tunnel: w958 -> [w965 _]
                  frame 0, Default {
                    n284 = global write "Global 1.vi" "PLC6 error"(w965) -> ()
                  }
                  frame 1, 66 {
                    n285 = call <vilib>:"disconnect.vi"("error in (no error)"=w977, "S7 Connection in"=w971) -> ("error out"=w976:errorcluster)  [unwired: 8 in, 1 out]
                    n286 = call <vilib>:"Clear Errors.vi"("error in (no error)"=w976) -> ("error out"=w973:errorcluster)  [unwired: 5 in, 1 out]
                    n287 = call <vilib>:"connect.vi"("Use Rack/Slot for S71200/1500"=TRUE, "Slot S7 300/400"=u8 1, "PLC Type"=PLC_Type."S7 1200" ("PLC Type 2"), "error in (no error)"=w973, "IP address"=w970) -> ("error out"=w975:errorcluster, "S7 Connection out"=w974:T5)  [unwired: 5 in]
                  }
                }
              }
            }
            n288 = Unbundle By Name(w952) -> ("status"=w955:bool)
            n289 = Not(x=w955) -> (.not. x?=w954:bool)
            "PLC 6" <- w954
            n290 = global write "Global 1.vi" "PLC 6"(w954) -> ()
          }
        }
        n291 = call "PADMINI_STOP_ALL.vi"("Enum"=enum16{"Read", "Write"}."Read") -> ("Boolean 2"=w784:bool)  [unwired: 9 in, 1 out]
        n292 = local read "stop"() -> (w783:bool)
        n293 = Or(x=w783, y=w784) -> (x .or. y?=w782:bool)
        n294 = Wait (ms)(milliseconds to wait=u32 1000) -> ()  [unwired: 1 out]
      }
      n295 = call <vilib>:"Clear Errors.vi"("error in (no error)"=w769) -> ("error out"=w757:errorcluster)  [unwired: 5 in, 1 out]
      n296 = call <vilib>:"disconnect.vi"("error in (no error)"=w757, "S7 Connection in"=w768) -> ("error out"=w756:errorcluster)  [unwired: 8 in, 1 out]
    }
    frame Enabled {
      w980 = PLC_Comm_State."Int"  # Enum
      n297 = while {
        shift-right: [w997] -> _
        shift-left: w980 -> [w1005]
        shift-right: [w989] -> w979
        shift-left: w981 -> [w1004]
        shift-right: [w1000] -> _
        shift-left: _ -> [w1003]
        tunnel: w982 -> [w986]
        shift-right: [w985] -> _
        shift-left: FALSE -> [w983]
        stop <- w998 stop-if-true
        w994 = PLC_Comm_State."Disconnect"  # Enum
        w1002 = u32 800  # milliseconds to wait
        # "Int-->Write-->Read---if--Error-->reconnect\n               ^------v                                       v\n                ^------------------------------v"
        # "OP 70-80"
        n298 = case shown="\"Write\"" w1005 {
          selector: w1005 -> [w1025 w1044 w1082 w1146 w1211 w1249 w1263 w1268 _ _]
          tunnel: [w1030 w1046 w1065 w1132 w1185 w1225 w1264 w1273 w1277 w1280] -> w1006
          tunnel: [w1031 w1045 w1064 w1133 w1184 w1224 w1265 w1270 w1276 w1279] -> w999
          tunnel: w1004 -> [w1028 w1040 w1066 w1131 w1186 w1222 w1261 w1271 w1277 w1280]
          tunnel: w1003 -> [w1026 _ w1067 w1130 w1187 w1223 w1265 w1272 w1276 w1279]
          tunnel: [w1024 w1043 w1081 w1147 w1210 w1250 w1262 w1267 _ _] -> w1001
          tunnel: [_ _ _ _ _ _ _ TRUE _ _] -> w998
          tunnel: [w1025 w1044 w1082 w1146 w1211 w1249 w1263 w1268 _ _] -> w995
          tunnel: w986 -> [w1023 w1042 _ _ _ _ _ _ _ _]
          tunnel: [w1022 w1037 w1060 FALSE w1183 w1221 w1260 w1266 w1275 w1278] -> w984
          tunnel: w983 -> [w1022 w1037 w1060 w1125 w1183 w1221 w1260 w1266 w1275 w1278]
          frame "Connect" {
            w1024 = PLC_Comm_State."Write"  # Enum
            w1036 = TRUE  # Use Rack/Slot for S71200/1500
            w1035 = u8 1  # Slot S7 300/400
            w1033 = u8 0  # Rack S7 300/400
            # "Reconect"
            n299 = call <vilib>:"disconnect.vi"("error in (no error)"=w1028, "S7 Connection in"=w1026) -> ("error out"=w1029:errorcluster)  [unwired: 8 in, 1 out]
            n300 = call <vilib>:"Clear Errors.vi"("error in (no error)"=w1029) -> ("error out"=w1027:errorcluster)  [unwired: 5 in, 1 out]
            n301 = call <vilib>:"connect.vi"("Use Rack/Slot for S71200/1500"=w1036, "Slot S7 300/400"=w1035, "PLC Type"=PLC_Type."S7 1200" ("PLC Type 2"), "error in (no error)"=w1027, "Rack S7 300/400"=w1033, "timeout [ms]"=1000 ("timeout [ms] 2"), "IP address"=w1023) -> ("error out"=w1030:errorcluster, "S7 Connection out"=w1031:T5)  [unwired: 3 in]
          }
          frame "Int" {
            w1043 = PLC_Comm_State."Write"  # Enum
            w1047 = TRUE  # Use Rack/Slot for S71200/1500
            w1048 = u8 1  # Slot S7 300/400
            w1049 = u8 0  # Rack S7 300/400
            # "Initialize and set first bits"
            n302 = call "Stall Data Flow.vim"("value in"=w1040, "milliseconds to wait"=u32 645) -> ("value out"=w1039:errorcluster)  [unwired: 1 out]
            n303 = call <vilib>:"connect.vi"("Use Rack/Slot for S71200/1500"=w1047, "Slot S7 300/400"=w1048, "PLC Type"=PLC_Type."S7 1200" ("PLC Type 2"), "error in (no error)"=w1039, "Rack S7 300/400"=w1049, "timeout [ms]"=1000 ("timeout [ms] 2"), "IP address"=w1042) -> ("error out"=w1051:errorcluster, "S7 Connection out"=w1050:T5)  [unwired: 3 in]
            n304 = for {
              tunnel: u16[] [80, 82] ("Data Block #") -> [w1059] mode=indexing
              shift-right: [w1057] -> w1045
              shift-left: w1050 -> [w1055]
              tunnel: w1051 -> [w1056]
              tunnel: [w1054] -> w1046
              w1058 = i32[] [0, 0]  # DINT input array
              # "Reset Search and save \nbit on software start"
              n305 = call-poly <vilib>:"write DB.vi"("DINT input array"=w1058, "error in (no error)"=w1056, "Data Block #"=w1059, "S7 Connection in"=w1055) -> ("error out"=w1054:errorcluster, "S7 Connection out"=w1057:T5)  [unwired: 4 in, 2 out]
            }
          }
          frame "Write" {
            w1069 = u16 81 ("Data Block #")
            w1081 = PLC_Comm_State."Write2"  # Enum
            # "OP 70 Write"
            n306 = global read "DATA LOG.vi" "OP 70 Outputs"() -> (w1080:bool)
            n307 = case shown="True" w1080 {
              tunnel: w1067 -> [w1106 w1119]
              tunnel: [w1107 w1108] -> w1078
              tunnel: [w1106 w1112] -> w1077
              tunnel: w1066 -> [w1107 w1116]
              frame False {
              }
              frame True {
                w1120 = u16 81  # Data Block #
                n308 = call "PADMINI_AUTO_BARCODE_STATUS 70.vi"("Enum"=enum16{"Read", "Write"}."Read", "error in (no error)"=w1116) -> ("error out"=w1115:errorcluster, "O/P"=w1117:i32[])  [unwired: 8 in]
                n309 = call-poly <vilib>:"write DB.vi"("DINT input array"=w1117, "error in (no error)"=w1115, "Data Block #"=w1120, "S7 Connection in"=w1119) -> ("error out"=w1110:errorcluster, "S7 Connection out"=w1111:T5)  [unwired: 4 in, 2 out]
                n310 = call-poly <vilib>:"write DB.vi"("DINT input array"=i32[] [0] ("Data Byte"), "error in (no error)"=w1110, "Data Block #"=u16 80, "S7 Connection in"=w1111) -> ("error out"=w1109:errorcluster, "S7 Connection out"=w1112:T5)  [unwired: 4 in, 2 out]
                n311 = case shown="No Error" w1109 {
                  selector: w1109 -> [w1121 w1123]
                  tunnel: [w1121 w1123] -> w1108
                  frame No Error {
                    n312 = global write "DATA LOG.vi" "OP 70 Outputs"(FALSE) -> ()
                  }
                  frame Error {
                  }
                }
              }
            }
            n313 = global read "DATA LOG.vi" "OP 70 reset"() -> (w1079:bool)
            n314 = global read "DATA LOG.vi" "Auto Cycle On"() -> (w1072:bool)
            n315 = case shown="True" w1079 {
              tunnel: w1078 -> [w1093 w1102]
              tunnel: [w1093 w1095] -> w1073
              tunnel: w1077 -> [w1094 w1101]
              tunnel: [w1094 w1100] -> w1074
              frame False {
              }
              frame True {
                n316 = call-poly <vilib>:"write DB.vi"("Item offset [byte]"=u16 4 ("Data Block #"), "DINT input array"=i32[] [0], "error in (no error)"=w1102, "Data Block #"=u16 80, "S7 Connection in"=w1101) -> ("error out"=w1096:errorcluster, "S7 Connection out"=w1100:T5)  [unwired: 3 in, 2 out]
                n317 = case shown="No Error" w1096 {
                  selector: w1096 -> [w1103 w1105]
                  tunnel: [w1103 w1105] -> w1095
                  frame No Error {
                    n318 = global write "DATA LOG.vi" "OP 70 reset"(FALSE) -> ()
                  }
                  frame Error {
                  }
                }
              }
            }
            n319 = Boolean To (0,1)(Boolean=w1072) -> (0, 1=w1071:i16)
            n320 = Build Array(w1071) -> (w1070:i16[])
            n321 = call-poly <vilib>:"write DB.vi"("Item offset [byte]"=u32 20, "DINT input array"=w1070, "error in (no error)"=w1073, "Data Block #"=w1069, "S7 Connection in"=w1074) -> ("error out"=w1075:errorcluster, "S7 Connection out"=w1076:T5)  [unwired: 3 in, 2 out]
            n322 = global read "Global 1.vi" "Filtered BARCODE selected"() -> (w1061:string[])
            n323 = call "Is Value Changed.vim"("value"=w1061) -> ("changed or first call?"=w1062:bool)
            n324 = Or(x=w1060, y=w1062) -> (x .or. y?=w1063:bool)
            n325 = case shown="False" w1063 {
              tunnel: w1076 -> [w1084 w1092]
              tunnel: w1075 -> [w1083 w1091]
              tunnel: w1061 -> [_ w1090]
              tunnel: w1069 -> [_ w1087]
              tunnel: [w1083 w1086] -> w1065
              tunnel: [w1084 w1085] -> w1064
              frame False {
              }
              frame True {
                n326 = call-poly <vilib>:"write DB.vi"("Item offset [byte]"=u32 24, "Input STRINGS"=w1090, "error in (no error)"=w1091, "String length reserved in DB (default=254)"=u16 15, "Data Block #"=w1087, "S7 Connection in"=w1092) -> ("error out"=w1086:errorcluster, "S7 Connection out"=w1085:T5)  [unwired: 2 in, 2 out]
              }
            }
          }
          frame "Write2" {
            w1135 = u16 83 ("Data Block #")
            w1147 = PLC_Comm_State."Read"  # Enum
            # "op 80 wirte 2"
            n327 = global read "DATA LOG.vi" "OP 80 Outputs"() -> (w1145:bool)
            n328 = case shown="True" w1145 {
              tunnel: [w1169 w1171] -> w1144
              tunnel: [w1168 w1174] -> w1140
              tunnel: w1131 -> [w1169 w1179]
              tunnel: w1130 -> [w1168 w1177]
              frame False {
              }
              frame True {
                w1182 = u16 83  # Data Block #
                n329 = call "PADMINI_AUTO_BARCODE_STATUS 80.vi"("Enum"=enum16{"Read", "Write"}."Read", "error in (no error)"=w1179) -> ("error out"=w1178:errorcluster, "O/P"=w1180:i32[])  [unwired: 8 in]
                n330 = call-poly <vilib>:"write DB.vi"("DINT input array"=w1180, "error in (no error)"=w1178, "Data Block #"=w1182, "S7 Connection in"=w1177) -> ("error out"=w1172:errorcluster, "S7 Connection out"=w1173:T5)  [unwired: 4 in, 2 out]
                n331 = call-poly <vilib>:"write DB.vi"("DINT input array"=i32[] [0] ("Data Byte"), "error in (no error)"=w1172, "Data Block #"=u16 82, "S7 Connection in"=w1173) -> ("error out"=w1171:errorcluster, "S7 Connection out"=w1174:T5)  [unwired: 4 in, 2 out]
                n332 = Unbundle By Name(w1171) -> ("status"=w1170:bool)
                n333 = global write "DATA LOG.vi" "OP 80 Outputs"(w1170) -> ()
              }
            }
            n334 = global read "DATA LOG.vi" "OP 80 reset"() -> (w1143:bool)
            n335 = case shown="True" w1143 {
              tunnel: w1144 -> [w1159 w1167]
              tunnel: [w1159 w1161] -> _
              tunnel: [w1159 w1161] -> w1141
              tunnel: w1140 -> [w1158 w1163]
              tunnel: [w1158 w1162] -> w1139
              frame False {
              }
              frame True {
                n336 = call-poly <vilib>:"write DB.vi"("Item offset [byte]"=u16 4 ("Data Block #"), "DINT input array"=i32[] [0], "error in (no error)"=w1167, "Data Block #"=u16 82, "S7 Connection in"=w1163) -> ("error out"=w1161:errorcluster, "S7 Connection out"=w1162:T5)  [unwired: 3 in, 2 out]
                n337 = Unbundle By Name(w1161) -> ("status"=w1160:bool)
                n338 = global write "DATA LOG.vi" "OP 80 reset"(w1160) -> ()
              }
            }
            n339 = global read "DATA LOG.vi" "Auto Cycle On"() -> (w1138:bool)
            n340 = Boolean To (0,1)(Boolean=w1138) -> (0, 1=w1137:i16)
            n341 = Build Array(w1137) -> (w1136:i16[])
            n342 = global read "Global 1.vi" "Filtered BARCODE selected"() -> (w1127:string[])
            n343 = call-poly <vilib>:"write DB.vi"("Item offset [byte]"=u32 20, "DINT input array"=w1136, "error in (no error)"=w1141, "Data Block #"=w1135, "S7 Connection in"=w1139) -> ("error out"=w1126:errorcluster, "S7 Connection out"=w1142:T5)  [unwired: 3 in, 2 out]
            n344 = call "Is Value Changed.vim"("value"=w1127) -> ("changed or first call?"=w1129:bool)
            n345 = Or(x=w1125, y=w1129) -> (x .or. y?=w1128:bool)
            n346 = case shown="False" w1128 {
              tunnel: w1142 -> [w1149 w1157]
              tunnel: w1126 -> [w1148 w1156]
              tunnel: w1127 -> [_ w1155]
              tunnel: w1135 -> [_ w1152]
              tunnel: [w1149 w1151] -> w1133
              tunnel: [w1148 w1150] -> w1132
              frame False {
              }
              frame True {
                n347 = call-poly <vilib>:"write DB.vi"("Item offset [byte]"=u32 24, "Input STRINGS"=w1155, "error in (no error)"=w1156, "String length reserved in DB (default=254)"=u16 15, "Data Block #"=w1152, "S7 Connection in"=w1157) -> ("error out"=w1150:errorcluster, "S7 Connection out"=w1151:T5)  [unwired: 2 in, 2 out]
              }
            }
          }
          frame "Read" {
            w1196 = u16 80 ("Data Block #")
            w1210 = PLC_Comm_State."Read2"  # Enum
            # "OP70 read"
            n348 = call-poly <vilib>:"read DB.vi"("Item offset [byte]"=u32 8, "error in (no error)"=w1186, "items #"=u16 2 ("Items # [byte]"), "Data Block #"=w1196, "S7 Connection in"=w1187) -> ("error out"=w1206:errorcluster, "REAL result array"=w1209:sgl[], "S7 Connection out"=w1207:T5)  [unwired: 4 in]
            n349 = call-poly <vilib>:"read DB.vi"("Item offset [byte]"=u32 16, "String length reserved in DB (default=254)"=u16 50, "error in (no error)"=w1206, "items #"=u16 1 ("Items # [byte]"), "Data Block #"=w1196, "S7 Connection in"=w1207) -> ("error out"=w1202:errorcluster, "STRING result Array"=w1201:string[], "S7 Connection out"=w1203:T5)  [unwired: 2 in, 1 out]
            n350 = call-poly <vilib>:"read DB.vi"("Item offset [byte]"=u32 68, "String length reserved in DB (default=254)"=u16 10, "error in (no error)"=w1202, "items #"=u16 1 ("Items # [byte]"), "Data Block #"=w1196, "S7 Connection in"=w1203) -> ("error out"=w1204:errorcluster, "STRING result Array"=w1205:string[], "S7 Connection out"=w1198:T5)  [unwired: 2 in, 1 out]
            n351 = Build Array (concatenate)(w1201, w1205) -> (w1208:string[])
            n352 = call-poly <vilib>:"read DB.vi"("error in (no error)"=w1204, "items #"=u16 2 ("Items # [byte]"), "Data Block #"=w1196, "S7 Connection in"=w1198) -> ("error out"=w1199:errorcluster, "DINT result array"=w1200:i32[], "S7 Connection out"=w1184:T5)  [unwired: 5 in]
            n353 = case shown="No Error" w1199 {
              selector: w1199 -> [w1214 w1220]
              tunnel: w1200 -> [w1219 _]
              tunnel: w1208 -> [w1218 _]
              tunnel: w1209 -> [w1215 _]
              tunnel: [w1213 w1220] -> w1185
              frame No Error {
                w1217 = enum16{"Read", "Write"}."Write" ("Enum")
                n354 = call "PADMINI_AUTO_BARCODE_STRING 70.vi"("Enum"=w1217, "error in (no error)"=w1214, "Input"=w1218) -> ("error out"=w1216:errorcluster)  [unwired: 7 in, 1 out]
                n355 = call "PADMINI_AUTO_CYCLE VALUE 70.vi"("Enum"=w1217, "error in (no error)"=w1216, "Input"=w1215) -> ("error out"=w1212:errorcluster)  [unwired: 7 in, 1 out]
                n356 = call "PADMINI_AUTO_CYCLE STATE 70.vi"("Enum"=w1217, "error in (no error)"=w1212, "Input"=w1219) -> ("error out"=w1213:errorcluster)  [unwired: 7 in, 1 out]
              }
              frame Error {
              }
            }
          }
          frame "Read2" {
            w1231 = u16 82 ("Data Block #")
            w1250 = PLC_Comm_State."Write"  # Enum
            # "Op80 Read2"
            n357 = call-poly <vilib>:"read DB.vi"("Item offset [byte]"=u32 8, "error in (no error)"=w1222, "items #"=u16 1 ("Items # [byte]"), "Data Block #"=w1231, "S7 Connection in"=w1223) -> ("error out"=w1237:errorcluster, "REAL result array"=w1248:sgl[], "S7 Connection out"=w1238:T5)  [unwired: 4 in]
            n358 = call-poly <vilib>:"read DB.vi"("Item offset [byte]"=u32 12, "String length reserved in DB (default=254)"=u16 50, "error in (no error)"=w1237, "items #"=u16 1 ("Items # [byte]"), "Data Block #"=w1231, "S7 Connection in"=w1238) -> ("error out"=w1240:errorcluster, "STRING result Array"=w1242:string[], "S7 Connection out"=w1243:T5)  [unwired: 2 in, 1 out]
            n359 = call-poly <vilib>:"read DB.vi"("Item offset [byte]"=u32 64, "String length reserved in DB (default=254)"=u16 10, "error in (no error)"=w1240, "items #"=u16 2 ("Items # [byte]"), "Data Block #"=w1231, "S7 Connection in"=w1243) -> ("error out"=w1241:errorcluster, "STRING result Array"=w1239:string[], "S7 Connection out"=w1246:T5)  [unwired: 2 in, 1 out]
            n360 = Build Array (concatenate)(w1242, w1239) -> (w1247:string[])
            n361 = call-poly <vilib>:"read DB.vi"("error in (no error)"=w1241, "items #"=u16 2 ("Items # [byte]"), "Data Block #"=u16 82, "S7 Connection in"=w1246) -> ("error out"=w1244:errorcluster, "DINT result array"=w1245:i32[], "S7 Connection out"=w1224:T5)  [unwired: 5 in]
            n362 = case shown="No Error" w1244 {
              selector: w1244 -> [w1253 w1259]
              tunnel: w1245 -> [w1258 _]
              tunnel: w1247 -> [w1256 _]
              tunnel: w1248 -> [w1255 _]
              tunnel: [w1251 w1259] -> w1225
              frame No Error {
                w1254 = enum16{"Read", "Write"}."Write" ("Enum")
                n363 = call "PADMINI_AUTO_CYCLE VALUE 80.vi"("Enum"=w1254, "error in (no error)"=w1253, "Input"=w1255) -> ("error out"=w1257:errorcluster)  [unwired: 7 in, 1 out]
                n364 = call "PADMINI_AUTO_BARCODE_STRING 80.vi"("Enum"=w1254, "error in (no error)"=w1257, "Input"=w1256) -> ("error out"=w1252:errorcluster)  [unwired: 7 in, 1 out]
                n365 = call "PADMINI_AUTO_CYCLE STATE 80.vi"("Enum"=w1254, "error in (no error)"=w1252, "Input"=w1258) -> ("error out"=w1251:errorcluster)  [unwired: 7 in, 1 out]
              }
              frame Error {
              }
            }
          }
          frame "Error" {
            w1262 = PLC_Comm_State."Connect"  # Enum
            n366 = global write "Global 1.vi" "PLC6 error"(w1261) -> ()
            n367 = call <vilib>:"Clear Errors.vi"("error in (no error)"=w1261) -> ("error out"=w1264:errorcluster)  [unwired: 5 in, 1 out]
          }
          frame "Disconnect" {
            w1267 = PLC_Comm_State."Disconnect"  # Enum
            w1270 = T5 {"TCP Connection Ref"=refnum, "IP address"="", "timeout ms"=5000, "Connected?"=FALSE, "PLC Type"=enum."S7 1200", "Rack S7 400"=0, "Slot S7 400"=0, "PDU Size"=0, "connection semaphore"=refnum}  # S7 Connection out
            n368 = call <vilib>:"Clear Errors.vi"("error in (no error)"=w1271) -> ("error out"=w1274:errorcluster)  [unwired: 5 in, 1 out]
            n369 = call <vilib>:"disconnect.vi"("error in (no error)"=w1274, "S7 Connection in"=w1272) -> ("error out"=w1273:errorcluster)  [unwired: 8 in, 1 out]
          }
          frame "Write3" {
            # "No Use"
          }
          frame "Read3" {
            # "No Use"
          }
        }
        n370 = Wait (ms)(milliseconds to wait=w1002) -> ()  [unwired: 1 out]
        n371 = call "PADMINI_STOP_ALL.vi"("Enum"=enum16{"Read", "Write"}."Read") -> ("Boolean 2"=w993:bool)  [unwired: 9 in, 1 out]
        n372 = local read "stop"() -> (w988:bool)
        n373 = case shown="Error" w1006 {
          selector: w1006 -> [w1010 w1017]
          tunnel: [w1010 w1016] -> w989
          tunnel: [w1009 w1015] -> w996
          tunnel: w1001 -> [w1009 _]
          tunnel: [w1008 w1021] -> w1000
          tunnel: w999 -> [w1008 w1021]
          tunnel: w995 -> [_ w1020]
          tunnel: [w1007 TRUE] -> w985
          tunnel: w984 -> [w1007 _]
          frame No Error {
          }
          frame Error {
            w1015 = PLC_Comm_State."Error"  # Enum
            w1012 = "    " ("string")
            n374 = Unbundle By Name(w1017) -> ("source"=w1013:string)
            n375 = Get Date/Time String() -> (time string=w1011:string)  [unwired: 3 in, 1 out]
            n376 = call <userlib>:"Get Strings from Enum__ogtk.vi"("Enum"=w1020) -> ("String Value"=w1019:string)  [unwired: 7 in, 3 out]
            n377 = Concatenate Strings(w1019, w1012, w1011, w1012, w1013) -> (w1018:string)
            n378 = Bundle By Name(cluster=w1017, "source"=w1018) -> (w1016:errorcluster)
          }
        }
        n379 = Or(x=w988, y=w993) -> (x .or. y?=w991:bool)
        n380 = Select(t=w994, s=w991, f=w996) -> (s? t:f=w997:T1)
        n381 = Unbundle By Name(w989) -> ("status"=w990:bool)
        n382 = Not(x=w990) -> (.not. x?=w987:bool)
        n383 = global write "Global 1.vi" "PLC 6"(w987) -> ()
      }
    }
  }
  n384 = disable-structure shown="Enabled" {
    disable-tunnel: w30 -> [w1293 w1494]
    disable-tunnel: [w1292 w1492] -> w3
    disable-tunnel: w10 -> [w1286 w1493]
    frame Disabled {
      w1283 = TRUE  # Use Rack/Slot for S71200/1500
      w1284 = u8 1  # Slot S7 300/400
      w1285 = u8 0  # Rack S7 300/400
      n385 = call <vilib>:"connect.vi"("Use Rack/Slot for S71200/1500"=w1283, "Slot S7 300/400"=w1284, "PLC Type"=PLC_Type."S7 1200" ("PLC Type 2"), "error in (no error)"=w1286, "Rack S7 300/400"=w1285, "timeout [ms]"=1000 ("timeout [ms] 2"), "IP address"=w1293) -> ("error out"=w1288:errorcluster, "S7 Connection out"=w1287:T5)  [unwired: 3 in]
      n386 = for {
        tunnel: u16[] [69, 71] ("Data Block #") -> [w1301] mode=indexing
        shift-right: [w1299] -> w1290
        shift-left: w1287 -> [w1296]
        tunnel: w1288 -> [w1297]
        tunnel: [w1298] -> w1289
        w1300 = i32[] [0, 0]  # DINT input array
        # "Reset Search and save \nbit on software start"
        n387 = call-poly <vilib>:"write DB.vi"("DINT input array"=w1300, "error in (no error)"=w1297, "Data Block #"=w1301, "S7 Connection in"=w1296) -> ("error out"=w1298:errorcluster, "S7 Connection out"=w1299:T5)  [unwired: 4 in, 2 out]
      }
      n388 = while {
        shift-right: [w1304] -> w1281
        shift-left: w1290 -> [w1314]
        shift-right: [w1312] -> w1292
        shift-left: w1289 -> [w1313]
        tunnel: w1293 -> [w1303]
        stop <- w1306 stop-if-true
        # "OP 90 - 100"
        n389 = flat-sequence {
          tunnel: [w1316] -> w1310
          tunnel: [w1386] -> w1305
          tunnel: w1313 -> [w1411]
          tunnel: w1314 -> [w1410]
          tunnel: w1303 -> [w1398]
          tunnel: [w1398] -> w1302
          tunnel: [w1464] -> w1312
          tunnel: [w1463] -> w1304
          tunnel: w1310 -> [w1466]
          tunnel: w1305 -> [w1465]
          tunnel: w1302 -> [w1462]
          frame #0 {
            w1355 = u16 72 ("Data Block #")
            w1379 = u16 70 ("Data Block #")
            w1315 = u16 71 ("Data Block #")
            w1323 = u16 69 ("Data Block #")
            # "AUTO WRITE"
            n390 = global read "DATA LOG.vi" "OP 90 Outputs"() -> (w1409:bool)
            n391 = case shown="True" w1409 {
              tunnel: w1410 -> [w1447 w1460]
              tunnel: [w1448 w1449] -> w1384
              tunnel: [w1447 w1450] -> w1385
              tunnel: w1411 -> [w1448 w1457]
              frame False {
              }
              frame True {
                w1461 = u16 70  # Data Block #
                n392 = call "PADMINI_AUTO_BARCODE_STATUS 90.vi"("Enum"=enum16{"Read", "Write"}."Read", "error in (no error)"=w1457) -> ("error out"=w1456:errorcluster, "O/P"=w1458:i32[])  [unwired: 8 in]
                n393 = global write "DATA LOG.vi" "OP 90 Outputs"(FALSE) -> ()
                n394 = call-poly <vilib>:"write DB.vi"("DINT input array"=w1458, "error in (no error)"=w1456, "Data Block #"=w1461, "S7 Connection in"=w1460) -> ("error out"=w1452:errorcluster, "S7 Connection out"=w1451:T5)  [unwired: 4 in, 2 out]
                n395 = call-poly <vilib>:"write DB.vi"("DINT input array"=i32[] [0] ("Data Byte"), "error in (no error)"=w1452, "Data Block #"=u16 69, "S7 Connection in"=w1451) -> ("error out"=w1449:errorcluster, "S7 Connection out"=w1450:T5)  [unwired: 4 in, 2 out]
              }
            }
            n396 = global read "DATA LOG.vi" "OP 90 reset"() -> (w1383:bool)
            n397 = case shown="True" w1383 {
              tunnel: w1384 -> [w1422 w1431]
              tunnel: [w1422 w1430] -> w1372
              tunnel: w1385 -> [w1423 w1429]
              tunnel: [w1423 w1428] -> w1373
              frame False {
              }
              frame True {
                n398 = global write "DATA LOG.vi" "OP 90 reset"(FALSE) -> ()
                n399 = call-poly <vilib>:"write DB.vi"("Item offset [byte]"=u16 4 ("Data Block #"), "DINT input array"=i32[] [0], "error in (no error)"=w1431, "Data Block #"=u16 69, "S7 Connection in"=w1429) -> ("error out"=w1430:errorcluster, "S7 Connection out"=w1428:T5)  [unwired: 3 in, 2 out]
              }
            }
            n400 = global read "DATA LOG.vi" "Auto Cycle On"() -> (w1338:bool)
            n401 = Boolean To (0,1)(Boolean=w1338) -> (0, 1=w1337:i16)
            n402 = Build Array(w1337) -> (w1336:i16[])
            n403 = global read "Global 1.vi" "Filtered BARCODE selected"() -> (w1382:string[])
            n404 = call-poly <vilib>:"write DB.vi"("Item offset [byte]"=u32 20, "DINT input array"=w1336, "error in (no error)"=w1372, "Data Block #"=w1379, "S7 Connection in"=w1373) -> ("error out"=w1377:errorcluster, "S7 Connection out"=w1376:T5)  [unwired: 3 in, 2 out]
            n405 = call-poly <vilib>:"write DB.vi"("Item offset [byte]"=u32 24, "Input STRINGS"=w1382, "error in (no error)"=w1377, "String length reserved in DB (default=254)"=u16 15, "Data Block #"=w1379, "S7 Connection in"=w1376) -> ("error out"=w1374:errorcluster, "S7 Connection out"=w1375:T5)  [unwired: 2 in, 2 out]
            n406 = call-poly <vilib>:"read DB.vi"("Item offset [byte]"=u32 8, "error in (no error)"=w1374, "items #"=u16 2 ("Items # [byte]"), "Data Block #"=w1323, "S7 Connection in"=w1375) -> ("error out"=w1401:errorcluster, "REAL result array"=w1399:sgl[], "S7 Connection out"=w1407:T5)  [unwired: 4 in]
            n407 = call "PADMINI_AUTO_CYCLE VALUE 90.vi"("Enum"=enum16{"Read", "Write"}."Write", "error in (no error)"=w1401, "Input"=w1399) -> ("error out"=w1400:errorcluster)  [unwired: 7 in, 1 out]
            n408 = call-poly <vilib>:"read DB.vi"("Item offset [byte]"=u32 16, "String length reserved in DB (default=254)"=u16 50, "error in (no error)"=w1400, "items #"=u16 1 ("Items # [byte]"), "Data Block #"=w1323, "S7 Connection in"=w1407) -> ("error out"=w1371:errorcluster, "STRING result Array"=w1364:string[], "S7 Connection out"=w1370:T5)  [unwired: 2 in, 1 out]
            n409 = call-poly <vilib>:"read DB.vi"("Item offset [byte]"=u32 68, "String length reserved in DB (default=254)"=u16 10, "error in (no error)"=w1371, "items #"=u16 3 ("Items # [byte]"), "Data Block #"=w1323, "S7 Connection in"=w1370) -> ("error out"=w1369:errorcluster, "STRING result Array"=w1363:string[], "S7 Connection out"=w1326:T5)  [unwired: 2 in, 1 out]
            n410 = Build Array (concatenate)(w1364, w1363) -> (w1362:string[])
            n411 = call "PADMINI_AUTO_BARCODE_STRING 90.vi"("Enum"=enum16{"Read", "Write"}."Write", "error in (no error)"=w1369, "Input"=w1362) -> ("error out"=w1325:errorcluster)  [unwired: 7 in, 1 out]
            n412 = call-poly <vilib>:"read DB.vi"("error in (no error)"=w1325, "items #"=u16 2 ("Items # [byte]"), "Data Block #"=w1323, "S7 Connection in"=w1326) -> ("error out"=w1329:errorcluster, "DINT result array"=w1331:i32[], "S7 Connection out"=w1327:T5)  [unwired: 5 in]
            n413 = call "PADMINI_AUTO_CYCLE STATE 90.vi"("Enum"=enum16{"Read", "Write"}."Write", "error in (no error)"=w1329, "Input"=w1331) -> ("error out"=w1324:errorcluster)  [unwired: 7 in, 1 out]
            n414 = global read "DATA LOG.vi" "OP 100 Outputs"() -> (w1387:bool)
            n415 = case shown="True" w1387 {
              tunnel: w1327 -> [w1432 w1445]
              tunnel: [w1433 w1436] -> w1360
              tunnel: [w1432 w1437] -> w1361
              tunnel: w1324 -> [w1433 w1442]
              frame False {
              }
              frame True {
                w1446 = u16 72  # Data Block #
                n416 = call "PADMINI_AUTO_BARCODE_STATUS 100.vi"("Enum"=enum16{"Read", "Write"}."Read", "error in (no error)"=w1442) -> ("error out"=w1441:errorcluster, "O/P"=w1443:i32[])  [unwired: 8 in]
                n417 = global write "DATA LOG.vi" "OP 100 Outputs"(FALSE) -> ()
                n418 = call-poly <vilib>:"write DB.vi"("DINT input array"=w1443, "error in (no error)"=w1441, "Data Block #"=w1446, "S7 Connection in"=w1445) -> ("error out"=w1435:errorcluster, "S7 Connection out"=w1434:T5)  [unwired: 4 in, 2 out]
                n419 = call-poly <vilib>:"write DB.vi"("DINT input array"=i32[] [0] ("Data Byte"), "error in (no error)"=w1435, "Data Block #"=u16 71, "S7 Connection in"=w1434) -> ("error out"=w1436:errorcluster, "S7 Connection out"=w1437:T5)  [unwired: 4 in, 2 out]
              }
            }
            n420 = global read "DATA LOG.vi" "OP 100 reset"() -> (w1359:bool)
            n421 = case shown="True" w1359 {
              tunnel: w1360 -> [w1412 w1421]
              tunnel: [w1412 w1420] -> w1351
              tunnel: w1361 -> [w1413 w1419]
              tunnel: [w1413 w1418] -> w1350
              frame False {
              }
              frame True {
                n422 = global write "DATA LOG.vi" "OP 100 reset"(FALSE) -> ()
                n423 = call-poly <vilib>:"write DB.vi"("Item offset [byte]"=u16 4 ("Data Block #"), "DINT input array"=i32[] [0], "error in (no error)"=w1421, "Data Block #"=u16 71, "S7 Connection in"=w1419) -> ("error out"=w1420:errorcluster, "S7 Connection out"=w1418:T5)  [unwired: 3 in, 2 out]
              }
            }
            n424 = global read "DATA LOG.vi" "Auto Cycle On"() -> (w1335:bool)
            n425 = Boolean To (0,1)(Boolean=w1335) -> (0, 1=w1334:i16)
            n426 = Build Array(w1334) -> (w1333:i16[])
            n427 = global read "Global 1.vi" "Filtered BARCODE selected"() -> (w1352:string[])
            n428 = call-poly <vilib>:"write DB.vi"("Item offset [byte]"=u32 20, "DINT input array"=w1333, "error in (no error)"=w1351, "Data Block #"=w1355, "S7 Connection in"=w1350) -> ("error out"=w1357:errorcluster, "S7 Connection out"=w1358:T5)  [unwired: 3 in, 2 out]
            n429 = call-poly <vilib>:"write DB.vi"("Item offset [byte]"=u32 24, "Input STRINGS"=w1352, "error in (no error)"=w1357, "String length reserved in DB (default=254)"=u16 15, "Data Block #"=w1355, "S7 Connection in"=w1358) -> ("error out"=w1348:errorcluster, "S7 Connection out"=w1349:T5)  [unwired: 2 in, 2 out]
            n430 = call-poly <vilib>:"read DB.vi"("Item offset [byte]"=u32 8, "error in (no error)"=w1348, "items #"=u16 11 ("Items # [byte]"), "Data Block #"=w1315, "S7 Connection in"=w1349) -> ("error out"=w1395:errorcluster, "REAL result array"=w1397:sgl[], "S7 Connection out"=w1389:T5)  [unwired: 4 in]
            n431 = call "PADMINI_AUTO_CYCLE VALUE 100.vi"("Enum"=enum16{"Read", "Write"}."Write", "error in (no error)"=w1395, "Input"=w1397) -> ("error out"=w1396:errorcluster)  [unwired: 7 in, 1 out]
            n432 = call-poly <vilib>:"read DB.vi"("Item offset [byte]"=u32 52, "String length reserved in DB (default=254)"=u16 50, "error in (no error)"=w1396, "items #"=u16 1 ("Items # [byte]"), "Data Block #"=w1315, "S7 Connection in"=w1389) -> ("error out"=w1345:errorcluster, "STRING result Array"=w1343:string[], "S7 Connection out"=w1344:T5)  [unwired: 2 in, 1 out]
            n433 = call-poly <vilib>:"read DB.vi"("Item offset [byte]"=u32 104, "String length reserved in DB (default=254)"=u16 10, "error in (no error)"=w1345, "items #"=u16 2 ("Items # [byte]"), "Data Block #"=w1315, "S7 Connection in"=w1344) -> ("error out"=w1346:errorcluster, "STRING result Array"=w1341:string[], "S7 Connection out"=w1317:T5)  [unwired: 2 in, 1 out]
            n434 = Build Array (concatenate)(w1343, w1341) -> (w1342:string[])
            n435 = call "PADMINI_AUTO_BARCODE_STRING 100.vi"("Enum"=enum16{"Read", "Write"}."Write", "error in (no error)"=w1346, "Input"=w1342) -> ("error out"=w1318:errorcluster)  [unwired: 7 in, 1 out]
            n436 = call-poly <vilib>:"read DB.vi"("error in (no error)"=w1318, "items #"=u16 2 ("Items # [byte]"), "Data Block #"=w1315, "S7 Connection in"=w1317) -> ("error out"=w1321:errorcluster, "DINT result array"=w1322:i32[], "S7 Connection out"=w1316:T5)  [unwired: 5 in]
            n437 = call "PADMINI_AUTO_CYCLE STATE 100.vi"("Enum"=enum16{"Read", "Write"}."Write", "error in (no error)"=w1321, "Input"=w1322) -> ("error out"=w1386:errorcluster)  [unwired: 7 in, 1 out]
          }
          frame #1 {
            # "RECONNECT"
            n438 = case shown="Error" w1465 {
              selector: w1465 -> [w1470 w1471]
              tunnel: [w1469 w1475] -> w1463
              tunnel: [w1470 w1476] -> w1464
              tunnel: w1466 -> [w1469 w1474]
              tunnel: w1462 -> [_ w1473]
              frame No Error {
              }
              frame Error {
                n439 = Unbundle By Name(w1471) -> ("code"=w1472:i32)
                n440 = call <vilib>:"Clear Errors.vi"("error in (no error)"=w1471) -> ("error out"=w1477:errorcluster)  [unwired: 5 in, 1 out]
                n441 = case shown="1, 66" w1472 {
                  tunnel: w1477 -> [w1479 w1490]
                  tunnel: [w1479 w1488] -> w1476
                  tunnel: [w1480 w1487] -> w1475
                  tunnel: w1474 -> [w1480 w1484]
                  tunnel: w1473 -> [_ w1483]
                  tunnel: w1471 -> [w1478 _]
                  frame 0, Default {
                    n442 = global write "Global 1.vi" "PLC7 error"(w1478) -> ()
                  }
                  frame 1, 66 {
                    n443 = call <vilib>:"disconnect.vi"("error in (no error)"=w1490, "S7 Connection in"=w1484) -> ("error out"=w1489:errorcluster)  [unwired: 8 in, 1 out]
                    n444 = call <vilib>:"Clear Errors.vi"("error in (no error)"=w1489) -> ("error out"=w1486:errorcluster)  [unwired: 5 in, 1 out]
                    n445 = call <vilib>:"connect.vi"("Use Rack/Slot for S71200/1500"=TRUE, "Slot S7 300/400"=u8 1, "PLC Type"=PLC_Type."S7 1200" ("PLC Type 2"), "error in (no error)"=w1486, "IP address"=w1483) -> ("error out"=w1488:errorcluster, "S7 Connection out"=w1487:T5)  [unwired: 5 in]
                  }
                }
              }
            }
            n446 = Unbundle By Name(w1465) -> ("status"=w1468:bool)
            n447 = Not(x=w1468) -> (.not. x?=w1467:bool)
            "PLC 7" <- w1467
            n448 = global write "Global 1.vi" "PLC 7"(w1467) -> ()
          }
        }
        n449 = call "PADMINI_STOP_ALL.vi"("Enum"=enum16{"Read", "Write"}."Read") -> ("Boolean 2"=w1308:bool)  [unwired: 9 in, 1 out]
        n450 = local read "stop"() -> (w1307:bool)
        n451 = Or(x=w1307, y=w1308) -> (x .or. y?=w1306:bool)
        n452 = Wait (ms)(milliseconds to wait=u32 1200) -> ()  [unwired: 1 out]
      }
      n453 = call <vilib>:"Clear Errors.vi"() -> ("error out"=w1282:errorcluster)  [unwired: 6 in, 1 out]
      n454 = call <vilib>:"disconnect.vi"("error in (no error)"=w1282, "S7 Connection in"=w1281) -> ()  [unwired: 8 in, 2 out]
    }
    frame Enabled {
      w1495 = PLC_Comm_State."Int"  # Enum
      n455 = while {
        shift-right: [w1510] -> _
        shift-left: w1495 -> [w1518]
        shift-right: [w1502] -> w1492
        shift-left: w1493 -> [w1517]
        shift-right: [w1513] -> _
        shift-left: _ -> [w1516]
        tunnel: w1494 -> [w1499]
        shift-right: [w1498] -> _
        shift-left: FALSE -> [w1496]
        stop <- w1511 stop-if-true
        w1507 = PLC_Comm_State."Disconnect"  # Enum
        w1515 = u32 800  # milliseconds to wait
        # "Int-->Write-->Read---if--Error-->reconnect\n               ^------v                                       v\n                ^------------------------------v"
        # "OP 90-100"
        n456 = case shown="\"Write\"" w1518 {
          selector: w1518 -> [w1538 w1557 w1595 w1653 w1718 w1755 w1769 w1774 _ _]
          tunnel: [w1543 w1559 w1580 w1637 w1694 w1731 w1770 w1779 w1783 w1786] -> w1519
          tunnel: [w1544 w1558 w1579 w1636 w1695 w1732 w1771 w1776 w1782 w1785] -> w1512
          tunnel: w1517 -> [w1541 w1553 w1577 w1639 w1698 w1730 w1767 w1777 w1783 w1786]
          tunnel: w1516 -> [w1539 _ w1578 w1638 w1699 w1729 w1771 w1778 w1782 w1785]
          tunnel: [w1537 w1556 w1594 w1654 w1717 w1756 w1768 w1773 _ _] -> w1514
          tunnel: [_ _ _ _ _ _ _ TRUE _ _] -> w1511
          tunnel: [w1538 w1557 w1595 w1653 w1718 w1755 w1769 w1774 _ _] -> w1508
          tunnel: w1499 -> [w1536 w1555 _ _ _ _ _ _ _ _]
          tunnel: [w1535 w1550 w1573 FALSE w1690 w1728 w1766 w1772 w1781 w1784] -> w1497
          tunnel: w1496 -> [w1535 w1550 w1573 w1632 w1690 w1728 w1766 w1772 w1781 w1784]
          frame "Connect" {
            w1537 = PLC_Comm_State."Write"  # Enum
            w1549 = TRUE  # Use Rack/Slot for S71200/1500
            w1548 = u8 1  # Slot S7 300/400
            w1546 = u8 0  # Rack S7 300/400
            # "Reconect"
            n457 = call <vilib>:"disconnect.vi"("error in (no error)"=w1541, "S7 Connection in"=w1539) -> ("error out"=w1542:errorcluster)  [unwired: 8 in, 1 out]
            n458 = call <vilib>:"Clear Errors.vi"("error in (no error)"=w1542) -> ("error out"=w1540:errorcluster)  [unwired: 5 in, 1 out]
            n459 = call <vilib>:"connect.vi"("Use Rack/Slot for S71200/1500"=w1549, "Slot S7 300/400"=w1548, "PLC Type"=PLC_Type."S7 1200" ("PLC Type 2"), "error in (no error)"=w1540, "Rack S7 300/400"=w1546, "timeout [ms]"=1000 ("timeout [ms] 2"), "IP address"=w1536) -> ("error out"=w1543:errorcluster, "S7 Connection out"=w1544:T5)  [unwired: 3 in]
          }
          frame "Int" {
            w1556 = PLC_Comm_State."Write"  # Enum
            w1560 = TRUE  # Use Rack/Slot for S71200/1500
            w1561 = u8 1  # Slot S7 300/400
            w1562 = u8 0  # Rack S7 300/400
            # "Initialize and set first bits"
            n460 = call "Stall Data Flow.vim"("value in"=w1553, "milliseconds to wait"=u32 774) -> ("value out"=w1552:errorcluster)  [unwired: 1 out]
            n461 = call <vilib>:"connect.vi"("Use Rack/Slot for S71200/1500"=w1560, "Slot S7 300/400"=w1561, "PLC Type"=PLC_Type."S7 1200" ("PLC Type 2"), "error in (no error)"=w1552, "Rack S7 300/400"=w1562, "timeout [ms]"=1000 ("timeout [ms] 2"), "IP address"=w1555) -> ("error out"=w1564:errorcluster, "S7 Connection out"=w1563:T5)  [unwired: 3 in]
            n462 = for {
              tunnel: u16[] [69, 71] ("Data Block #") -> [w1572] mode=indexing
              shift-right: [w1570] -> w1558
              shift-left: w1563 -> [w1568]
              tunnel: w1564 -> [w1569]
              tunnel: [w1567] -> w1559
              w1571 = i32[] [0, 0]  # DINT input array
              # "Reset Search and save \nbit on software start"
              n463 = call-poly <vilib>:"write DB.vi"("DINT input array"=w1571, "error in (no error)"=w1569, "Data Block #"=w1572, "S7 Connection in"=w1568) -> ("error out"=w1567:errorcluster, "S7 Connection out"=w1570:T5)  [unwired: 4 in, 2 out]
            }
          }
          frame "Write" {
            w1582 = u16 70 ("Data Block #")
            w1594 = PLC_Comm_State."Write2"  # Enum
            # "OP 90 Write"
            n464 = global read "DATA LOG.vi" "OP 90 Outputs"() -> (w1587:bool)
            n465 = case shown="True" w1587 {
              tunnel: [w1616 w1621] -> w1588
              tunnel: [w1617 w1622] -> w1589
              tunnel: w1578 -> [w1617 w1619]
              tunnel: w1577 -> [w1616 w1618]
              frame False {
              }
              frame True {
                w1630 = u16 70  # Data Block #
                n466 = call "PADMINI_AUTO_BARCODE_STATUS 90.vi"("Enum"=enum16{"Read", "Write"}."Read", "error in (no error)"=w1618) -> ("error out"=w1627:errorcluster, "O/P"=w1628:i32[])  [unwired: 8 in]
                n467 = call-poly <vilib>:"write DB.vi"("DINT input array"=w1628, "error in (no error)"=w1627, "Data Block #"=w1630, "S7 Connection in"=w1619) -> ("error out"=w1624:errorcluster, "S7 Connection out"=w1623:T5)  [unwired: 4 in, 2 out]
                n468 = call-poly <vilib>:"write DB.vi"("DINT input array"=i32[] [0] ("Data Byte"), "error in (no error)"=w1624, "Data Block #"=u16 69, "S7 Connection in"=w1623) -> ("error out"=w1621:errorcluster, "S7 Connection out"=w1622:T5)  [unwired: 4 in, 2 out]
                n469 = Unbundle By Name(w1621) -> ("status"=w1620:bool)
                n470 = global write "DATA LOG.vi" "OP 90 Outputs"(w1620) -> ()
              }
            }
            n471 = global read "DATA LOG.vi" "Auto Cycle On"() -> (w1584:bool)
            n472 = global read "DATA LOG.vi" "OP 90 reset"() -> (w1593:bool)
            n473 = Boolean To (0,1)(Boolean=w1584) -> (0, 1=w1583:i16)
            n474 = case shown="True" w1593 {
              tunnel: w1588 -> [w1606 w1612]
              tunnel: w1589 -> [w1607 w1611]
              tunnel: [w1607 w1610] -> w1590
              tunnel: [w1606 w1609] -> w1591
              frame False {
              }
              frame True {
                n475 = call-poly <vilib>:"write DB.vi"("Item offset [byte]"=u16 4 ("Data Block #"), "DINT input array"=i32[] [0], "error in (no error)"=w1612, "Data Block #"=u16 69, "S7 Connection in"=w1611) -> ("error out"=w1609:errorcluster, "S7 Connection out"=w1610:T5)  [unwired: 3 in, 2 out]
                n476 = Unbundle By Name(w1609) -> ("status"=w1608:bool)
                n477 = global write "DATA LOG.vi" "OP 90 reset"(w1608) -> ()
              }
            }
            n478 = Build Array(w1583) -> (w1592:i16[])
            n479 = global read "Global 1.vi" "Filtered BARCODE selected"() -> (w1576:string[])
            n480 = call-poly <vilib>:"write DB.vi"("Item offset [byte]"=u32 20, "DINT input array"=w1592, "error in (no error)"=w1591, "Data Block #"=w1582, "S7 Connection in"=w1590) -> ("error out"=w1586:errorcluster, "S7 Connection out"=w1585:T5)  [unwired: 3 in, 2 out]
            n481 = call "Is Value Changed.vim"("value"=w1576) -> ("changed or first call?"=w1574:bool)
            n482 = Or(x=w1573, y=w1574) -> (x .or. y?=w1575:bool)
            n483 = case shown="False" w1575 {
              tunnel: w1576 -> [_ w1605]
              tunnel: w1586 -> [w1596 w1604]
              tunnel: w1585 -> [w1597 w1603]
              tunnel: w1582 -> [_ w1600]
              tunnel: [w1596 w1599] -> w1580
              tunnel: [w1597 w1598] -> w1579
              frame False {
              }
              frame True {
                n484 = call-poly <vilib>:"write DB.vi"("Item offset [byte]"=u32 24, "Input STRINGS"=w1605, "error in (no error)"=w1604, "String length reserved in DB (default=254)"=u16 15, "Data Block #"=w1600, "S7 Connection in"=w1603) -> ("error out"=w1599:errorcluster, "S7 Connection out"=w1598:T5)  [unwired: 2 in, 2 out]
              }
            }
          }
          frame "Write2" {
            w1641 = u16 72 ("Data Block #")
            w1654 = PLC_Comm_State."Read"  # Enum
            # "op 100 wirte 2"
            n485 = global read "DATA LOG.vi" "OP 100 Outputs"() -> (w1652:bool)
            n486 = case shown="True" w1652 {
              tunnel: w1638 -> [w1675 w1688]
              tunnel: [w1676 w1678] -> w1650
              tunnel: [w1675 w1681] -> w1651
              tunnel: w1639 -> [w1676 w1685]
              frame False {
              }
              frame True {
                w1689 = u16 72  # Data Block #
                n487 = call "PADMINI_AUTO_BARCODE_STATUS 100.vi"("Enum"=enum16{"Read", "Write"}."Read", "error in (no error)"=w1685) -> ("error out"=w1684:errorcluster, "O/P"=w1686:i32[])  [unwired: 8 in]
                n488 = call-poly <vilib>:"write DB.vi"("DINT input array"=w1686, "error in (no error)"=w1684, "Data Block #"=w1689, "S7 Connection in"=w1688) -> ("error out"=w1680:errorcluster, "S7 Connection out"=w1679:T5)  [unwired: 4 in, 2 out]
                n489 = call-poly <vilib>:"write DB.vi"("DINT input array"=i32[] [0] ("Data Byte"), "error in (no error)"=w1680, "Data Block #"=u16 71, "S7 Connection in"=w1679) -> ("error out"=w1678:errorcluster, "S7 Connection out"=w1681:T5)  [unwired: 4 in, 2 out]
                n490 = Unbundle By Name(w1678) -> ("status"=w1677:bool)
                n491 = global write "DATA LOG.vi" "OP 100 Outputs"(w1677) -> ()
              }
            }
            n492 = global read "DATA LOG.vi" "OP 100 reset"() -> (w1649:bool)
            n493 = case shown="True" w1649 {
              tunnel: w1650 -> [w1665 w1674]
              tunnel: [w1665 w1668] -> w1646
              tunnel: w1651 -> [w1666 w1673]
              tunnel: [w1666 w1672] -> w1645
              frame False {
              }
              frame True {
                n494 = call-poly <vilib>:"write DB.vi"("Item offset [byte]"=u16 4 ("Data Block #"), "DINT input array"=i32[] [0], "error in (no error)"=w1674, "Data Block #"=u16 71, "S7 Connection in"=w1673) -> ("error out"=w1668:errorcluster, "S7 Connection out"=w1672:T5)  [unwired: 3 in, 2 out]
                n495 = Unbundle By Name(w1668) -> ("status"=w1667:bool)
                n496 = global write "DATA LOG.vi" "OP 100 reset"(w1667) -> ()
              }
            }
            n497 = global read "DATA LOG.vi" "Auto Cycle On"() -> (w1644:bool)
            n498 = global read "Global 1.vi" "Filtered BARCODE selected"() -> (w1635:string[])
            n499 = Boolean To (0,1)(Boolean=w1644) -> (0, 1=w1643:i16)
            n500 = Build Array(w1643) -> (w1642:i16[])
            n501 = call-poly <vilib>:"write DB.vi"("Item offset [byte]"=u32 20, "DINT input array"=w1642, "error in (no error)"=w1646, "Data Block #"=w1641, "S7 Connection in"=w1645) -> ("error out"=w1647:errorcluster, "S7 Connection out"=w1648:T5)  [unwired: 3 in, 2 out]
            n502 = call "Is Value Changed.vim"("value"=w1635) -> ("changed or first call?"=w1633:bool)
            n503 = Or(x=w1632, y=w1633) -> (x .or. y?=w1634:bool)
            n504 = case shown="True" w1634 {
              tunnel: w1648 -> [w1656 w1664]
              tunnel: w1647 -> [w1655 w1663]
              tunnel: w1635 -> [_ w1662]
              tunnel: w1641 -> [_ w1659]
              tunnel: [w1655 w1658] -> w1637
              tunnel: [w1656 w1657] -> w1636
              frame False {
              }
              frame True {
                n505 = call-poly <vilib>:"write DB.vi"("Item offset [byte]"=u32 24, "Input STRINGS"=w1662, "error in (no error)"=w1663, "String length reserved in DB (default=254)"=u16 15, "Data Block #"=w1659, "S7 Connection in"=w1664) -> ("error out"=w1658:errorcluster, "S7 Connection out"=w1657:T5)  [unwired: 2 in, 2 out]
              }
            }
          }
          frame "Read" {
            w1708 = u16 69 ("Data Block #")
            w1717 = PLC_Comm_State."Read2"  # Enum
            # "OP90 read"
            n506 = call-poly <vilib>:"read DB.vi"("Item offset [byte]"=u32 8, "error in (no error)"=w1698, "items #"=u16 2 ("Items # [byte]"), "Data Block #"=w1708, "S7 Connection in"=w1699) -> ("error out"=w1715:errorcluster, "REAL result array"=w1691:sgl[], "S7 Connection out"=w1716:T5)  [unwired: 4 in]
            n507 = call-poly <vilib>:"read DB.vi"("Item offset [byte]"=u32 16, "String length reserved in DB (default=254)"=u16 50, "error in (no error)"=w1715, "items #"=u16 1 ("Items # [byte]"), "Data Block #"=w1708, "S7 Connection in"=w1716) -> ("error out"=w1714:errorcluster, "STRING result Array"=w1712:string[], "S7 Connection out"=w1713:T5)  [unwired: 2 in, 1 out]
            n508 = call-poly <vilib>:"read DB.vi"("Item offset [byte]"=u32 68, "String length reserved in DB (default=254)"=u16 10, "error in (no error)"=w1714, "items #"=u16 3 ("Items # [byte]"), "Data Block #"=w1708, "S7 Connection in"=w1713) -> ("error out"=w1692:errorcluster, "STRING result Array"=w1711:string[], "S7 Connection out"=w1710:T5)  [unwired: 2 in, 1 out]
            n509 = Build Array (concatenate)(w1712, w1711) -> (w1697:string[])
            n510 = call-poly <vilib>:"read DB.vi"("error in (no error)"=w1692, "items #"=u16 2 ("Items # [byte]"), "Data Block #"=w1708, "S7 Connection in"=w1710) -> ("error out"=w1693:errorcluster, "DINT result array"=w1696:i32[], "S7 Connection out"=w1695:T5)  [unwired: 5 in]
            n511 = case shown="No Error" w1693 {
              selector: w1693 -> [w1721 w1727]
              tunnel: w1696 -> [w1726 _]
              tunnel: w1697 -> [w1725 _]
              tunnel: [w1720 w1727] -> w1694
              tunnel: w1691 -> [w1719 _]
              frame No Error {
                w1724 = enum16{"Read", "Write"}."Write" ("Enum")
                n512 = call "PADMINI_AUTO_CYCLE VALUE 90.vi"("Enum"=w1724, "error in (no error)"=w1721, "Input"=w1719) -> ("error out"=w1723:errorcluster)  [unwired: 7 in, 1 out]
                n513 = call "PADMINI_AUTO_BARCODE_STRING 90.vi"("Enum"=w1724, "error in (no error)"=w1723, "Input"=w1725) -> ("error out"=w1722:errorcluster)  [unwired: 7 in, 1 out]
                n514 = call "PADMINI_AUTO_CYCLE STATE 90.vi"("Enum"=w1724, "error in (no error)"=w1722, "Input"=w1726) -> ("error out"=w1720:errorcluster)  [unwired: 7 in, 1 out]
              }
              frame Error {
              }
            }
          }
          frame "Read2" {
            w1741 = u16 71 ("Data Block #")
            w1756 = PLC_Comm_State."Write"  # Enum
            # "Op100 Read2"
            n515 = call-poly <vilib>:"read DB.vi"("Item offset [byte]"=u32 8, "error in (no error)"=w1730, "items #"=u16 11 ("Items # [byte]"), "Data Block #"=w1741, "S7 Connection in"=w1729) -> ("error out"=w1752:errorcluster, "REAL result array"=w1754:sgl[], "S7 Connection out"=w1751:T5)  [unwired: 4 in]
            n516 = call-poly <vilib>:"read DB.vi"("Item offset [byte]"=u32 52, "String length reserved in DB (default=254)"=u16 50, "error in (no error)"=w1752, "items #"=u16 1 ("Items # [byte]"), "Data Block #"=w1741, "S7 Connection in"=w1751) -> ("error out"=w1749:errorcluster, "STRING result Array"=w1747:string[], "S7 Connection out"=w1748:T5)  [unwired: 2 in, 1 out]
            n517 = call-poly <vilib>:"read DB.vi"("Item offset [byte]"=u32 104, "String length reserved in DB (default=254)"=u16 10, "error in (no error)"=w1749, "items #"=u16 2 ("Items # [byte]"), "Data Block #"=w1741, "S7 Connection in"=w1748) -> ("error out"=w1750:errorcluster, "STRING result Array"=w1746:string[], "S7 Connection out"=w1743:T5)  [unwired: 2 in, 1 out]
            n518 = Build Array (concatenate)(w1747, w1746) -> (w1753:string[])
            n519 = call-poly <vilib>:"read DB.vi"("error in (no error)"=w1750, "items #"=u16 2 ("Items # [byte]"), "Data Block #"=w1741, "S7 Connection in"=w1743) -> ("error out"=w1744:errorcluster, "DINT result array"=w1745:i32[], "S7 Connection out"=w1732:T5)  [unwired: 5 in]
            n520 = case shown="No Error" w1744 {
              selector: w1744 -> [w1761 w1765]
              tunnel: w1745 -> [w1764 _]
              tunnel: w1753 -> [w1759 _]
              tunnel: w1754 -> [w1758 _]
              tunnel: [w1757 w1765] -> w1731
              frame No Error {
                w1760 = enum16{"Read", "Write"}."Write" ("Enum")
                n521 = call "PADMINI_AUTO_CYCLE VALUE 100.vi"("Enum"=w1760, "error in (no error)"=w1761, "Input"=w1758) -> ("error out"=w1762:errorcluster)  [unwired: 7 in, 1 out]
                n522 = call "PADMINI_AUTO_BARCODE_STRING 100.vi"("Enum"=w1760, "error in (no error)"=w1762, "Input"=w1759) -> ("error out"=w1763:errorcluster)  [unwired: 7 in, 1 out]
                n523 = call "PADMINI_AUTO_CYCLE STATE 100.vi"("Enum"=w1760, "error in (no error)"=w1763, "Input"=w1764) -> ("error out"=w1757:errorcluster)  [unwired: 7 in, 1 out]
              }
              frame Error {
              }
            }
          }
          frame "Error" {
            w1768 = PLC_Comm_State."Connect"  # Enum
            n524 = global write "Global 1.vi" "PLC7 error"(w1767) -> ()
            n525 = call <vilib>:"Clear Errors.vi"("error in (no error)"=w1767) -> ("error out"=w1770:errorcluster)  [unwired: 5 in, 1 out]
          }
          frame "Disconnect" {
            w1773 = PLC_Comm_State."Disconnect"  # Enum
            w1776 = T5 {"TCP Connection Ref"=refnum, "IP address"="", "timeout ms"=5000, "Connected?"=FALSE, "PLC Type"=enum."S7 1200", "Rack S7 400"=0, "Slot S7 400"=0, "PDU Size"=0, "connection semaphore"=refnum}  # S7 Connection out
            n526 = call <vilib>:"Clear Errors.vi"("error in (no error)"=w1777) -> ("error out"=w1780:errorcluster)  [unwired: 5 in, 1 out]
            n527 = call <vilib>:"disconnect.vi"("error in (no error)"=w1780, "S7 Connection in"=w1778) -> ("error out"=w1779:errorcluster)  [unwired: 8 in, 1 out]
          }
          frame "Write3" {
            # "No Use"
          }
          frame "Read3" {
            # "No Use"
          }
        }
        n528 = Wait (ms)(milliseconds to wait=w1515) -> ()  [unwired: 1 out]
        n529 = call "PADMINI_STOP_ALL.vi"("Enum"=enum16{"Read", "Write"}."Read") -> ("Boolean 2"=w1506:bool)  [unwired: 9 in, 1 out]
        n530 = local read "stop"() -> (w1501:bool)
        n531 = case shown="Error" w1519 {
          selector: w1519 -> [w1523 w1530]
          tunnel: [w1523 w1529] -> w1502
          tunnel: [w1522 w1528] -> w1509
          tunnel: w1514 -> [w1522 _]
          tunnel: [w1521 w1534] -> w1513
          tunnel: w1512 -> [w1521 w1534]
          tunnel: w1508 -> [_ w1532]
          tunnel: [w1520 TRUE] -> w1498
          tunnel: w1497 -> [w1520 _]
          frame No Error {
          }
          frame Error {
            w1528 = PLC_Comm_State."Error"  # Enum
            w1525 = "    " ("string")
            n532 = Unbundle By Name(w1530) -> ("source"=w1533:string)
            n533 = Get Date/Time String() -> (time string=w1524:string)  [unwired: 3 in, 1 out]
            n534 = call <userlib>:"Get Strings from Enum__ogtk.vi"("Enum"=w1532) -> ("String Value"=w1526:string)  [unwired: 7 in, 3 out]
            n535 = Concatenate Strings(w1526, w1525, w1524, w1525, w1533) -> (w1531:string)
            n536 = Bundle By Name(cluster=w1530, "source"=w1531) -> (w1529:errorcluster)
          }
        }
        n537 = Or(x=w1501, y=w1506) -> (x .or. y?=w1504:bool)
        n538 = Select(t=w1507, s=w1504, f=w1509) -> (s? t:f=w1510:T1)
        n539 = Unbundle By Name(w1502) -> ("status"=w1503:bool)
        n540 = Not(x=w1503) -> (.not. x?=w1500:bool)
        n541 = global write "Global 1.vi" "PLC 7"(w1500) -> ()
      }
    }
  }
  n542 = disable-structure shown="Enabled" {
    disable-tunnel: w72 -> [w1799 w1925]
    disable-tunnel: w10 -> [w1792 w1924]
    disable-tunnel: [w1787 w1923] -> w5
    frame Disabled {
      w1789 = TRUE  # Use Rack/Slot for S71200/1500
      w1790 = u8 1  # Slot S7 300/400
      w1791 = u8 0  # Rack S7 300/400
      w1798 = i32[] [0, 0]  # DINT input array
      # "Reset Search and save \nbit on software start"
      n543 = call <vilib>:"connect.vi"("Use Rack/Slot for S71200/1500"=w1789, "Slot S7 300/400"=w1790, "PLC Type"=PLC_Type."S7 1200" ("PLC Type 2"), "error in (no error)"=w1792, "Rack S7 300/400"=w1791, "timeout [ms]"=1000 ("timeout [ms] 2"), "IP address"=w1799) -> ("error out"=w1794:errorcluster, "S7 Connection out"=w1793:T5)  [unwired: 3 in]
      n544 = call-poly <vilib>:"write DB.vi"("DINT input array"=w1798, "error in (no error)"=w1794, "Data Block #"=u16 56, "S7 Connection in"=w1793) -> ("error out"=w1795:errorcluster, "S7 Connection out"=w1796:T5)  [unwired: 4 in, 2 out]
      n545 = while {
        shift-right: [w1806] -> w1803
        shift-left: w1796 -> [w1816]
        shift-right: [w1814] -> w1802
        shift-left: w1795 -> [w1815]
        tunnel: w1799 -> [w1805]
        stop <- w1808 stop-if-true
        # "OP 50"
        n546 = flat-sequence {
          tunnel: [w1819] -> w1812
          tunnel: [w1817] -> w1807
          tunnel: w1815 -> [w1867]
          tunnel: w1816 -> [w1866]
          tunnel: w1805 -> [w1854]
          tunnel: [w1854] -> w1804
          tunnel: [w1895] -> w1814
          tunnel: [w1894] -> w1806
          tunnel: w1812 -> [w1897]
          tunnel: w1807 -> [w1896]
          tunnel: w1804 -> [w1893]
          frame #0 {
            w1837 = u16 57 ("Data Block #")
            w1845 = u16 56 ("Data Block #")
            # "AUTO WRITE"
            n547 = global read "DATA LOG.vi" "OP 50 Outputs"() -> (w1865:bool)
            n548 = case shown="True" w1865 {
              tunnel: w1866 -> [w1878 w1891]
              tunnel: [w1879 w1880] -> w1853
              tunnel: [w1878 w1883] -> w1852
              tunnel: w1867 -> [w1879 w1888]
              frame False {
              }
              frame True {
                w1892 = u16 57  # Data Block #
                n549 = call "PADMINI_AUTO_BARCODE_STATUS 50.vi"("Enum"=enum16{"Read", "Write"}."Read", "error in (no error)"=w1888) -> ("error out"=w1887:errorcluster, "O/P"=w1889:i32[])  [unwired: 8 in]
                n550 = global write "DATA LOG.vi" "OP 50 Outputs"(FALSE) -> ()
                n551 = call-poly <vilib>:"write DB.vi"("DINT input array"=w1889, "error in (no error)"=w1887, "Data Block #"=w1892, "S7 Connection in"=w1891) -> ("error out"=w1881:errorcluster, "S7 Connection out"=w1882:T5)  [unwired: 4 in, 2 out]
                n552 = call-poly <vilib>:"write DB.vi"("DINT input array"=i32[] [0] ("Data Byte"), "error in (no error)"=w1881, "Data Block #"=u16 56, "S7 Connection in"=w1882) -> ("error out"=w1880:errorcluster, "S7 Connection out"=w1883:T5)  [unwired: 4 in, 2 out]
              }
            }
            n553 = global read "DATA LOG.vi" "OP 50 reset"() -> (w1851:bool)
            n554 = global read "DATA LOG.vi" "Auto Cycle On"() -> (w1828:bool)
            n555 = case shown="True" w1851 {
              tunnel: w1853 -> [w1868 w1877]
              tunnel: [w1868 w1876] -> w1830
              tunnel: w1852 -> [w1869 w1875]
              tunnel: [w1869 w1874] -> w1833
              frame False {
              }
              frame True {
                n556 = global write "DATA LOG.vi" "OP 50 reset"(FALSE) -> ()
                n557 = call-poly <vilib>:"write DB.vi"("Item offset [byte]"=u16 4 ("Data Block #"), "DINT input array"=i32[] [0], "error in (no error)"=w1877, "Data Block #"=u16 56, "S7 Connection in"=w1875) -> ("error out"=w1876:errorcluster, "S7 Connection out"=w1874:T5)  [unwired: 3 in, 2 out]
              }
            }
            n558 = Boolean To (0,1)(Boolean=w1828) -> (0, 1=w1827:i16)
            n559 = Build Array(w1827) -> (w1826:i16[])
            n560 = global read "Global 1.vi" "Filtered BARCODE selected"() -> (w1834:string[])
            n561 = call-poly <vilib>:"write DB.vi"("Item offset [byte]"=u32 20, "DINT input array"=w1826, "error in (no error)"=w1830, "Data Block #"=w1837, "S7 Connection in"=w1833) -> ("error out"=w1839:errorcluster, "S7 Connection out"=w1840:T5)  [unwired: 3 in, 2 out]
            n562 = call-poly <vilib>:"write DB.vi"("Item offset [byte]"=u32 24, "Input STRINGS"=w1834, "error in (no error)"=w1839, "String length reserved in DB (default=254)"=u16 15, "Data Block #"=w1837, "S7 Connection in"=w1840) -> ("error out"=w1831:errorcluster, "S7 Connection out"=w1832:T5)  [unwired: 2 in, 2 out]
            n563 = call-poly <vilib>:"read DB.vi"("Item offset [byte]"=u32 8, "error in (no error)"=w1831, "items #"=u16 3 ("Items # [byte]"), "Data Block #"=w1845, "S7 Connection in"=w1832) -> ("error out"=w1857:errorcluster, "REAL result array"=w1855:sgl[], "S7 Connection out"=w1863:T5)  [unwired: 4 in]
            n564 = call "PADMINI_AUTO_CYCLE VALUE 50.vi"("Enum"=enum16{"Read", "Write"}."Write", "error in (no error)"=w1857, "Input"=w1855) -> ("error out"=w1856:errorcluster)  [unwired: 7 in, 1 out]
            n565 = call-poly <vilib>:"read DB.vi"("Item offset [byte]"=u32 20, "String length reserved in DB (default=254)"=u16 50, "error in (no error)"=w1856, "items #"=u16 1 ("Items # [byte]"), "Data Block #"=w1845, "S7 Connection in"=w1863) -> ("error out"=w1847:errorcluster, "STRING result Array"=w1844:string[], "S7 Connection out"=w1846:T5)  [unwired: 2 in, 1 out]
            n566 = call-poly <vilib>:"read DB.vi"("Item offset [byte]"=u32 72, "String length reserved in DB (default=254)"=u16 10, "error in (no error)"=w1847, "items #"=u16 5 ("Items # [byte]"), "Data Block #"=w1845, "S7 Connection in"=w1846) -> ("error out"=w1848:errorcluster, "STRING result Array"=w1843:string[], "S7 Connection out"=w1820:T5)  [unwired: 2 in, 1 out]
            n567 = Build Array (concatenate)(w1844, w1843) -> (w1842:string[])
            n568 = call "PADMINI_AUTO_BARCODE_STRING 50.vi"("Enum"=enum16{"Read", "Write"}."Write", "error in (no error)"=w1848, "Input"=w1842) -> ("error out"=w1818:errorcluster)  [unwired: 7 in, 1 out]
            n569 = call-poly <vilib>:"read DB.vi"("error in (no error)"=w1818, "items #"=u16 2 ("Items # [byte]"), "Data Block #"=u16 56, "S7 Connection in"=w1820) -> ("error out"=w1822:errorcluster, "DINT result array"=w1824:i32[], "S7 Connection out"=w1819:T5)  [unwired: 5 in]
            n570 = call "PADMINI_AUTO_CYCLE STATE 50.vi"("Enum"=enum16{"Read", "Write"}."Write", "error in (no error)"=w1822, "Input"=w1824) -> ("error out"=w1817:errorcluster)  [unwired: 7 in, 1 out]
          }
          frame #1 {
            # "RECONNECT"
            n571 = case shown="Error" w1896 {
              selector: w1896 -> [w1901 w1902]
              tunnel: [w1900 w1906] -> w1894
              tunnel: [w1901 w1907] -> w1895
              tunnel: w1897 -> [w1900 w1905]
              tunnel: w1893 -> [_ w1904]
              frame No Error {
              }
              frame Error {
                n572 = Unbundle By Name(w1902) -> ("code"=w1903:i32)
                n573 = call <vilib>:"Clear Errors.vi"("error in (no error)"=w1902) -> ("error out"=w1908:errorcluster)  [unwired: 5 in, 1 out]
                n574 = case shown="1, 66" w1903 {
                  tunnel: w1908 -> [w1910 w1921]
                  tunnel: [w1910 w1919] -> w1907
                  tunnel: [w1911 w1918] -> w1906
                  tunnel: w1905 -> [w1911 w1915]
                  tunnel: w1904 -> [_ w1914]
                  tunnel: w1902 -> [w1909 _]
                  frame 0, Default {
                    n575 = global write "Global 1.vi" "PLC4 error"(w1909) -> ()
                  }
                  frame 1, 66 {
                    n576 = call <vilib>:"disconnect.vi"("error in (no error)"=w1921, "S7 Connection in"=w1915) -> ("error out"=w1920:errorcluster)  [unwired: 8 in, 1 out]
                    n577 = call <vilib>:"Clear Errors.vi"("error in (no error)"=w1920) -> ("error out"=w1917:errorcluster)  [unwired: 5 in, 1 out]
                    n578 = call <vilib>:"connect.vi"("Use Rack/Slot for S71200/1500"=TRUE, "Slot S7 300/400"=u8 1, "PLC Type"=PLC_Type."S7 1200" ("PLC Type 2"), "error in (no error)"=w1917, "IP address"=w1914) -> ("error out"=w1919:errorcluster, "S7 Connection out"=w1918:T5)  [unwired: 5 in]
                  }
                }
              }
            }
            n579 = Unbundle By Name(w1896) -> ("status"=w1899:bool)
            n580 = Not(x=w1899) -> (.not. x?=w1898:bool)
            "PLC 4" <- w1898
            n581 = global write "Global 1.vi" "PLC 4"(w1898) -> ()
          }
        }
        n582 = call "PADMINI_STOP_ALL.vi"("Enum"=enum16{"Read", "Write"}."Read") -> ("Boolean 2"=w1810:bool)  [unwired: 9 in, 1 out]
        n583 = local read "stop"() -> (w1809:bool)
        n584 = Or(x=w1809, y=w1810) -> (x .or. y?=w1808:bool)
        n585 = Wait (ms)(milliseconds to wait=u32 1200) -> ()  [unwired: 1 out]
      }
      n586 = call <vilib>:"Clear Errors.vi"("error in (no error)"=w1802) -> ("error out"=w1788:errorcluster)  [unwired: 5 in, 1 out]
      n587 = call <vilib>:"disconnect.vi"("error in (no error)"=w1788, "S7 Connection in"=w1803) -> ("error out"=w1787:errorcluster)  [unwired: 8 in, 1 out]
    }
    frame Enabled {
      w1926 = PLC_Comm_State."Int"  # Enum
      n588 = while {
        shift-right: [w1941] -> _
        shift-left: w1926 -> [w1949]
        shift-right: [w1933] -> w1923
        shift-left: w1924 -> [w1948]
        shift-right: [w1944] -> _
        shift-left: _ -> [w1947]
        tunnel: w1925 -> [w1930]
        shift-right: [w1929] -> _
        shift-left: FALSE -> [w1927]
        stop <- w1942 stop-if-true
        w1938 = PLC_Comm_State."Disconnect"  # Enum
        w1946 = u32 800  # milliseconds to wait
        # "Int-->Write-->Read---if--Error-->reconnect\n               ^------v                                       v\n                ^------------------------------v"
        # "OP 50"
        n589 = case shown="\"Write\"" w1949 {
          selector: w1949 -> [w1969 w1987 w2027 w2091 w2104 w2109 _ _ _ _]
          tunnel: [w1974 w1989 w2010 w2066 w2105 w2114 w2117 w2121 w2124 w2127] -> w1950
          tunnel: [w1975 w1988 w2009 w2065 w2106 w2111 w2118 w2120 w2123 w2126] -> w1943
          tunnel: w1948 -> [w1972 w1983 w2011 w2067 w2102 w2112 w2117 w2121 w2124 w2127]
          tunnel: w1947 -> [w1970 _ w2012 w2064 w2106 w2113 w2118 w2120 w2123 w2126]
          tunnel: [w1968 w1986 w2026 w2090 w2103 w2108 _ _ _ _] -> w1945
          tunnel: [_ _ _ _ _ TRUE _ _ _ _] -> w1942
          tunnel: [w1969 w1987 w2027 w2091 w2104 w2109 _ _ _ _] -> w1939
          tunnel: w1930 -> [w1967 w1985 _ _ _ _ _ _ _ _]
          tunnel: [w1966 w1981 FALSE w2063 w2101 w2107 w2116 w2119 w2122 w2125] -> w1928
          tunnel: w1927 -> [w1966 w1981 w2004 w2063 w2101 w2107 w2116 w2119 w2122 w2125]
          frame "Connect" {
            w1968 = PLC_Comm_State."Write"  # Enum
            w1980 = TRUE  # Use Rack/Slot for S71200/1500
            w1979 = u8 1  # Slot S7 300/400
            w1977 = u8 0  # Rack S7 300/400
            # "Reconect"
            n590 = call <vilib>:"disconnect.vi"("error in (no error)"=w1972, "S7 Connection in"=w1970) -> ("error out"=w1973:errorcluster)  [unwired: 8 in, 1 out]
            n591 = call <vilib>:"Clear Errors.vi"("error in (no error)"=w1973) -> ("error out"=w1971:errorcluster)  [unwired: 5 in, 1 out]
            n592 = call <vilib>:"connect.vi"("Use Rack/Slot for S71200/1500"=w1980, "Slot S7 300/400"=w1979, "PLC Type"=PLC_Type."S7 1200" ("PLC Type 2"), "error in (no error)"=w1971, "Rack S7 300/400"=w1977, "timeout [ms]"=1000 ("timeout [ms] 2"), "IP address"=w1967) -> ("error out"=w1974:errorcluster, "S7 Connection out"=w1975:T5)  [unwired: 3 in]
          }
          frame "Int" {
            w1986 = PLC_Comm_State."Write"  # Enum
            w1990 = TRUE  # Use Rack/Slot for S71200/1500
            w1991 = u8 1  # Slot S7 300/400
            w1992 = u8 0  # Rack S7 300/400
            w1993 = u16[] [56]  # Data Block #
            # "Initialize and set first bits"
            n593 = call "Stall Data Flow.vim"("value in"=w1983, "milliseconds to wait"=u32 387) -> ("value out"=w1982:errorcluster)  [unwired: 1 out]
            n594 = call <vilib>:"connect.vi"("Use Rack/Slot for S71200/1500"=w1990, "Slot S7 300/400"=w1991, "PLC Type"=PLC_Type."S7 1200" ("PLC Type 2"), "error in (no error)"=w1982, "Rack S7 300/400"=w1992, "timeout [ms]"=1000 ("timeout [ms] 2"), "IP address"=w1985) -> ("error out"=w1995:errorcluster, "S7 Connection out"=w1994:T5)  [unwired: 3 in]
            n595 = for {
              tunnel: w1993 -> [w2003] mode=indexing
              shift-right: [w2001] -> w1988
              shift-left: w1994 -> [w1999]
              tunnel: w1995 -> [w2000]
              tunnel: [w1998] -> w1989
              w2002 = i32[] [0, 0]  # DINT input array
              # "Reset Search and save \nbit on software start"
              n596 = call-poly <vilib>:"write DB.vi"("DINT input array"=w2002, "error in (no error)"=w2000, "Data Block #"=w2003, "S7 Connection in"=w1999) -> ("error out"=w1998:errorcluster, "S7 Connection out"=w2001:T5)  [unwired: 4 in, 2 out]
            }
          }
          frame "Write" {
            w2014 = u16 57 ("Data Block #")
            w2026 = PLC_Comm_State."Read"  # Enum
            n597 = global read "DATA LOG.vi" "OP 50 Outputs"() -> (w2025:bool)
            n598 = case shown="True" w2025 {
              tunnel: w2012 -> [w2048 w2061]
              tunnel: [w2049 w2051] -> w2024
              tunnel: [w2048 w2054] -> w2023
              tunnel: w2011 -> [w2049 w2058]
              frame False {
              }
              frame True {
                w2062 = u16 57  # Data Block #
                n599 = call "PADMINI_AUTO_BARCODE_STATUS 50.vi"("Enum"=enum16{"Read", "Write"}."Read", "error in (no error)"=w2058) -> ("error out"=w2057:errorcluster, "O/P"=w2059:i32[])  [unwired: 8 in]
                n600 = call-poly <vilib>:"write DB.vi"("DINT input array"=w2059, "error in (no error)"=w2057, "Data Block #"=w2062, "S7 Connection in"=w2061) -> ("error out"=w2052:errorcluster, "S7 Connection out"=w2053:T5)  [unwired: 4 in, 2 out]
                n601 = call-poly <vilib>:"write DB.vi"("DINT input array"=i32[] [0] ("Data Byte"), "error in (no error)"=w2052, "Data Block #"=u16 56, "S7 Connection in"=w2053) -> ("error out"=w2051:errorcluster, "S7 Connection out"=w2054:T5)  [unwired: 4 in, 2 out]
                n602 = Unbundle By Name(w2051) -> ("status"=w2050:bool)
                n603 = global write "DATA LOG.vi" "OP 50 Outputs"(w2050) -> ()
              }
            }
            n604 = global read "DATA LOG.vi" "OP 50 reset"() -> (w2022:bool)
            n605 = case shown="True" w2022 {
              tunnel: w2024 -> [w2038 w2047]
              tunnel: [w2038 w2041] -> w2018
              tunnel: w2023 -> [w2039 w2046]
              tunnel: [w2039 w2045] -> w2019
              frame False {
              }
              frame True {
                n606 = call-poly <vilib>:"write DB.vi"("Item offset [byte]"=u16 4 ("Data Block #"), "DINT input array"=i32[] [0], "error in (no error)"=w2047, "Data Block #"=u16 56, "S7 Connection in"=w2046) -> ("error out"=w2041:errorcluster, "S7 Connection out"=w2045:T5)  [unwired: 3 in, 2 out]
                n607 = Unbundle By Name(w2041) -> ("status"=w2040:bool)
                n608 = global write "DATA LOG.vi" "OP 50 reset"(w2040) -> ()
              }
            }
            n609 = global read "DATA LOG.vi" "Auto Cycle On"() -> (w2017:bool)
            n610 = global read "Global 1.vi" "Filtered BARCODE selected"() -> (w2007:string[])
            n611 = Boolean To (0,1)(Boolean=w2017) -> (0, 1=w2016:i16)
            n612 = Build Array(w2016) -> (w2015:i16[])
            n613 = call-poly <vilib>:"write DB.vi"("Item offset [byte]"=u32 20, "DINT input array"=w2015, "error in (no error)"=w2018, "Data Block #"=w2014, "S7 Connection in"=w2019) -> ("error out"=w2020:errorcluster, "S7 Connection out"=w2021:T5)  [unwired: 3 in, 2 out]
            n614 = call "Is Value Changed.vim"("value"=w2007) -> ("changed or first call?"=w2005:bool)
            n615 = Or(x=w2004, y=w2005) -> (x .or. y?=w2006:bool)
            n616 = case shown="False" w2006 {
              tunnel: w2021 -> [w2029 w2037]
              tunnel: w2020 -> [w2028 w2036]
              tunnel: w2007 -> [_ w2035]
              tunnel: w2014 -> [_ w2032]
              tunnel: [w2028 w2031] -> w2010
              tunnel: [w2029 w2030] -> w2009
              frame False {
              }
              frame True {
                n617 = call-poly <vilib>:"write DB.vi"("Item offset [byte]"=u32 24, "Input STRINGS"=w2035, "error in (no error)"=w2036, "String length reserved in DB (default=254)"=u16 15, "Data Block #"=w2032, "S7 Connection in"=w2037) -> ("error out"=w2031:errorcluster, "S7 Connection out"=w2030:T5)  [unwired: 2 in, 2 out]
              }
            }
          }
          frame "Read" {
            w2076 = u16 56 ("Data Block #")
            w2090 = PLC_Comm_State."Write"  # Enum
            # "OP 50 Read"
            n618 = call-poly <vilib>:"read DB.vi"("error in (no error)"=w2067, "items #"=u16 2 ("Items # [byte]"), "Data Block #"=w2076, "S7 Connection in"=w2064) -> ("error out"=w2088:errorcluster, "DINT result array"=w2084:i32[], "S7 Connection out"=w2087:T5)  [unwired: 5 in]
            n619 = call-poly <vilib>:"read DB.vi"("Item offset [byte]"=u32 8, "error in (no error)"=w2088, "items #"=u16 3 ("Items # [byte]"), "Data Block #"=w2076, "S7 Connection in"=w2087) -> ("error out"=w2082:errorcluster, "REAL result array"=w2086:sgl[], "S7 Connection out"=w2083:T5)  [unwired: 4 in]
            n620 = call-poly <vilib>:"read DB.vi"("Item offset [byte]"=u32 20, "String length reserved in DB (default=254)"=u16 50, "error in (no error)"=w2082, "items #"=u16 1 ("Items # [byte]"), "Data Block #"=w2076, "S7 Connection in"=w2083) -> ("error out"=w2081:errorcluster, "STRING result Array"=w2079:string[], "S7 Connection out"=w2080:T5)  [unwired: 2 in, 1 out]
            n621 = call-poly <vilib>:"read DB.vi"("Item offset [byte]"=u32 72, "String length reserved in DB (default=254)"=u16 10, "error in (no error)"=w2081, "items #"=u16 5 ("Items # [byte]"), "Data Block #"=w2076, "S7 Connection in"=w2080) -> ("error out"=w2089:errorcluster, "STRING result Array"=w2078:string[], "S7 Connection out"=w2065:T5)  [unwired: 2 in, 1 out]
            n622 = Build Array (concatenate)(w2079, w2078) -> (w2085:string[])
            n623 = case shown="No Error" w2089 {
              selector: w2089 -> [w2095 w2100]
              tunnel: w2084 -> [w2099 _]
              tunnel: w2085 -> [w2097 _]
              tunnel: w2086 -> [w2094 _]
              tunnel: [w2093 w2100] -> w2066
              frame No Error {
                w2092 = enum16{"Read", "Write"}."Write" ("Enum")
                n624 = call "PADMINI_AUTO_CYCLE VALUE 50.vi"("Enum"=w2092, "error in (no error)"=w2095, "Input"=w2094) -> ("error out"=w2096:errorcluster)  [unwired: 7 in, 1 out]
                n625 = call "PADMINI_AUTO_BARCODE_STRING 50.vi"("Enum"=w2092, "error in (no error)"=w2096, "Input"=w2097) -> ("error out"=w2098:errorcluster)  [unwired: 7 in, 1 out]
                n626 = call "PADMINI_AUTO_CYCLE STATE 50.vi"("Enum"=w2092, "error in (no error)"=w2098, "Input"=w2099) -> ("error out"=w2093:errorcluster)  [unwired: 7 in, 1 out]
              }
              frame Error {
              }
            }
          }
          frame "Error" {
            w2103 = PLC_Comm_State."Connect"  # Enum
            n627 = global write "Global 1.vi" "PLC4 error"(w2102) -> ()
            n628 = call <vilib>:"Clear Errors.vi"("error in (no error)"=w2102) -> ("error out"=w2105:errorcluster)  [unwired: 5 in, 1 out]
          }
          frame "Disconnect" {
            w2108 = PLC_Comm_State."Disconnect"  # Enum
            w2111 = T5 {"TCP Connection Ref"=refnum, "IP address"="", "timeout ms"=5000, "Connected?"=FALSE, "PLC Type"=enum."S7 1200", "Rack S7 400"=0, "Slot S7 400"=0, "PDU Size"=0, "connection semaphore"=refnum}  # S7 Connection out
            n629 = call <vilib>:"Clear Errors.vi"("error in (no error)"=w2112) -> ("error out"=w2115:errorcluster)  [unwired: 5 in, 1 out]
            n630 = call <vilib>:"disconnect.vi"("error in (no error)"=w2115, "S7 Connection in"=w2113) -> ("error out"=w2114:errorcluster)  [unwired: 8 in, 1 out]
          }
          frame "Write2" {
            # "No Use"
          }
          frame "Write3" {
            # "No Use"
          }
          frame "Read2" {
            # "No Use"
          }
          frame "Read3" {
            # "No Use"
          }
        }
        n631 = Wait (ms)(milliseconds to wait=w1946) -> ()  [unwired: 1 out]
        n632 = call "PADMINI_STOP_ALL.vi"("Enum"=enum16{"Read", "Write"}."Read") -> ("Boolean 2"=w1937:bool)  [unwired: 9 in, 1 out]
        n633 = local read "stop"() -> (w1932:bool)
        n634 = case shown="Error" w1950 {
          selector: w1950 -> [w1954 w1961]
          tunnel: [w1954 w1960] -> w1933
          tunnel: [w1953 w1959] -> w1940
          tunnel: w1945 -> [w1953 _]
          tunnel: [w1952 w1965] -> w1944
          tunnel: w1943 -> [w1952 w1965]
          tunnel: w1939 -> [_ w1964]
          tunnel: [w1951 TRUE] -> w1929
          tunnel: w1928 -> [w1951 _]
          frame No Error {
          }
          frame Error {
            w1959 = PLC_Comm_State."Error"  # Enum
            w1956 = "    " ("string")
            n635 = Unbundle By Name(w1961) -> ("source"=w1957:string)
            n636 = Get Date/Time String() -> (time string=w1955:string)  [unwired: 3 in, 1 out]
            n637 = call <userlib>:"Get Strings from Enum__ogtk.vi"("Enum"=w1964) -> ("String Value"=w1963:string)  [unwired: 7 in, 3 out]
            n638 = Concatenate Strings(w1963, w1956, w1955, w1956, w1957) -> (w1962:string)
            n639 = Bundle By Name(cluster=w1961, "source"=w1962) -> (w1960:errorcluster)
          }
        }
        n640 = Or(x=w1932, y=w1937) -> (x .or. y?=w1935:bool)
        n641 = Select(t=w1938, s=w1935, f=w1940) -> (s? t:f=w1941:T1)
        n642 = Unbundle By Name(w1933) -> ("status"=w1934:bool)
        n643 = Not(x=w1934) -> (.not. x?=w1931:bool)
        n644 = global write "Global 1.vi" "PLC 4"(w1931) -> ()
      }
    }
  }
  n645 = disable-structure shown="Enabled" {
    disable-tunnel: w62 -> [w2140 w2266]
    disable-tunnel: w10 -> [w2133 w2265]
    disable-tunnel: [w2128 w2264] -> w7
    frame Disabled {
      w2130 = TRUE  # Use Rack/Slot for S71200/1500
      w2131 = u8 1  # Slot S7 300/400
      w2132 = u8 0  # Rack S7 300/400
      w2138 = i32[] [0, 0]  # DINT input array
      # "Reset Search and save \nbit on software start"
      n646 = call <vilib>:"connect.vi"("Use Rack/Slot for S71200/1500"=w2130, "Slot S7 300/400"=w2131, "PLC Type"=PLC_Type."S7 1200" ("PLC Type 2"), "error in (no error)"=w2133, "Rack S7 300/400"=w2132, "timeout [ms]"=1000 ("timeout [ms] 2"), "IP address"=w2140) -> ("error out"=w2134:errorcluster, "S7 Connection out"=w2135:T5)  [unwired: 3 in]
      n647 = call-poly <vilib>:"write DB.vi"("DINT input array"=w2138, "error in (no error)"=w2134, "Data Block #"=u16 43, "S7 Connection in"=w2135) -> ("error out"=w2137:errorcluster, "S7 Connection out"=w2136:T5)  [unwired: 4 in, 2 out]
      n648 = while {
        shift-right: [w2147] -> w2141
        shift-left: w2136 -> [w2157]
        shift-right: [w2155] -> w2142
        shift-left: w2137 -> [w2156]
        tunnel: w2140 -> [w2146]
        stop <- w2149 stop-if-true
        # "OP 60"
        n649 = flat-sequence {
          tunnel: [w2160] -> w2153
          tunnel: [w2158] -> w2148
          tunnel: w2156 -> [w2208]
          tunnel: w2157 -> [w2207]
          tunnel: w2146 -> [w2195]
          tunnel: [w2195] -> w2145
          tunnel: [w2236] -> w2155
          tunnel: [w2235] -> w2147
          tunnel: w2153 -> [w2238]
          tunnel: w2148 -> [w2237]
          tunnel: w2145 -> [w2234]
          frame #0 {
            w2191 = u16 44 ("Data Block #")
            w2172 = u16 43 ("Data Block #")
            # "AUTO WRITE"
            n650 = global read "DATA LOG.vi" "OP 60 Outputs"() -> (w2206:bool)
            n651 = case shown="True" w2206 {
              tunnel: w2207 -> [w2219 w2232]
              tunnel: [w2220 w2221] -> w2183
              tunnel: [w2219 w2224] -> w2182
              tunnel: w2208 -> [w2220 w2229]
              frame False {
              }
              frame True {
                w2233 = u16 44  # Data Block #
                n652 = call "PADMINI_AUTO_BARCODE_STATUS 60.vi"("Enum"=enum16{"Read", "Write"}."Read", "error in (no error)"=w2229) -> ("error out"=w2228:errorcluster, "O/P"=w2230:i32[])  [unwired: 8 in]
                n653 = global write "DATA LOG.vi" "OP 60 Outputs"(FALSE) -> ()
                n654 = call-poly <vilib>:"write DB.vi"("DINT input array"=w2230, "error in (no error)"=w2228, "Data Block #"=w2233, "S7 Connection in"=w2232) -> ("error out"=w2222:errorcluster, "S7 Connection out"=w2223:T5)  [unwired: 4 in, 2 out]
                n655 = call-poly <vilib>:"write DB.vi"("DINT input array"=i32[] [0] ("Data Byte"), "error in (no error)"=w2222, "Data Block #"=u16 43, "S7 Connection in"=w2223) -> ("error out"=w2221:errorcluster, "S7 Connection out"=w2224:T5)  [unwired: 4 in, 2 out]
              }
            }
            n656 = global read "DATA LOG.vi" "OP 60 reset"() -> (w2181:bool)
            n657 = global read "DATA LOG.vi" "Auto Cycle On"() -> (w2169:bool)
            n658 = case shown="True" w2181 {
              tunnel: w2183 -> [w2209 w2218]
              tunnel: [w2209 w2217] -> w2184
              tunnel: w2182 -> [w2210 w2216]
              tunnel: [w2210 w2215] -> w2185
              frame False {
              }
              frame True {
                n659 = global write "DATA LOG.vi" "OP 60 reset"(FALSE) -> ()
                n660 = call-poly <vilib>:"write DB.vi"("Item offset [byte]"=u16 4 ("Data Block #"), "DINT input array"=i32[] [0], "error in (no error)"=w2218, "Data Block #"=u16 43, "S7 Connection in"=w2216) -> ("error out"=w2217:errorcluster, "S7 Connection out"=w2215:T5)  [unwired: 3 in, 2 out]
              }
            }
            n661 = Boolean To (0,1)(Boolean=w2169) -> (0, 1=w2168:i16)
            n662 = Build Array(w2168) -> (w2167:i16[])
            n663 = global read "Global 1.vi" "Filtered BARCODE selected"() -> (w2194:string[])
            n664 = call-poly <vilib>:"write DB.vi"("Item offset [byte]"=u32 20, "DINT input array"=w2167, "error in (no error)"=w2184, "Data Block #"=w2191, "S7 Connection in"=w2185) -> ("error out"=w2189:errorcluster, "S7 Connection out"=w2188:T5)  [unwired: 3 in, 2 out]
            n665 = call-poly <vilib>:"write DB.vi"("Item offset [byte]"=u32 24, "Input STRINGS"=w2194, "error in (no error)"=w2189, "String length reserved in DB (default=254)"=u16 15, "Data Block #"=w2191, "S7 Connection in"=w2188) -> ("error out"=w2186:errorcluster, "S7 Connection out"=w2187:T5)  [unwired: 2 in, 2 out]
            n666 = call-poly <vilib>:"read DB.vi"("Item offset [byte]"=u32 8, "error in (no error)"=w2186, "items #"=u16 6 ("Items # [byte]"), "Data Block #"=w2172, "S7 Connection in"=w2187) -> ("error out"=w2198:errorcluster, "REAL result array"=w2196:sgl[], "S7 Connection out"=w2204:T5)  [unwired: 4 in]
            n667 = call "PADMINI_AUTO_CYCLE VALUE 60.vi"("Enum"=enum16{"Read", "Write"}."Write", "error in (no error)"=w2198, "Input"=w2196) -> ("error out"=w2197:errorcluster)  [unwired: 7 in, 1 out]
            n668 = call-poly <vilib>:"read DB.vi"("Item offset [byte]"=u32 32, "String length reserved in DB (default=254)"=u16 50, "error in (no error)"=w2197, "items #"=u16 1 ("Items # [byte]"), "Data Block #"=w2172, "S7 Connection in"=w2204) -> ("error out"=w2176:errorcluster, "STRING result Array"=w2174:string[], "S7 Connection out"=w2175:T5)  [unwired: 2 in, 1 out]
            n669 = call-poly <vilib>:"read DB.vi"("Item offset [byte]"=u32 84, "String length reserved in DB (default=254)"=u16 10, "error in (no error)"=w2176, "items #"=u16 7 ("Items # [byte]"), "Data Block #"=w2172, "S7 Connection in"=w2175) -> ("error out"=w2177:errorcluster, "STRING result Array"=w2180:string[], "S7 Connection out"=w2161:T5)  [unwired: 2 in, 1 out]
            n670 = Build Array (concatenate)(w2174, w2180) -> (w2173:string[])
            n671 = call "PADMINI_AUTO_BARCODE_STRING 60.vi"("Enum"=enum16{"Read", "Write"}."Write", "error in (no error)"=w2177, "Input"=w2173) -> ("error out"=w2159:errorcluster)  [unwired: 7 in, 1 out]
            n672 = call-poly <vilib>:"read DB.vi"("error in (no error)"=w2159, "items #"=u16 2 ("Items # [byte]"), "Data Block #"=u16 43, "S7 Connection in"=w2161) -> ("error out"=w2166:errorcluster, "DINT result array"=w2164:i32[], "S7 Connection out"=w2160:T5)  [unwired: 5 in]
            n673 = call "PADMINI_AUTO_CYCLE STATE 60.vi"("Enum"=enum16{"Read", "Write"}."Write", "error in (no error)"=w2166, "Input"=w2164) -> ("error out"=w2158:errorcluster)  [unwired: 7 in, 1 out]
          }
          frame #1 {
            # "RECONNECT"
            n674 = case shown="Error" w2237 {
              selector: w2237 -> [w2242 w2243]
              tunnel: [w2241 w2247] -> w2235
              tunnel: [w2242 w2248] -> w2236
              tunnel: w2238 -> [w2241 w2246]
              tunnel: w2234 -> [_ w2245]
              frame No Error {
              }
              frame Error {
                n675 = Unbundle By Name(w2243) -> ("code"=w2244:i32)
                n676 = call <vilib>:"Clear Errors.vi"("error in (no error)"=w2243) -> ("error out"=w2249:errorcluster)  [unwired: 5 in, 1 out]
                n677 = case shown="0, Default" w2244 {
                  tunnel: w2249 -> [w2251 w2262]
                  tunnel: [w2251 w2260] -> w2248
                  tunnel: [w2252 w2259] -> w2247
                  tunnel: w2246 -> [w2252 w2256]
                  tunnel: w2245 -> [_ w2255]
                  tunnel: w2243 -> [w2250 _]
                  frame 0, Default {
                    n678 = global write "Global 1.vi" "PLC5 error"(w2250) -> ()
                  }
                  frame 1, 66 {
                    n679 = call <vilib>:"disconnect.vi"("error in (no error)"=w2262, "S7 Connection in"=w2256) -> ("error out"=w2261:errorcluster)  [unwired: 8 in, 1 out]
                    n680 = call <vilib>:"Clear Errors.vi"("error in (no error)"=w2261) -> ("error out"=w2258:errorcluster)  [unwired: 5 in, 1 out]
                    n681 = call <vilib>:"connect.vi"("Use Rack/Slot for S71200/1500"=TRUE, "Slot S7 300/400"=u8 1, "PLC Type"=PLC_Type."S7 1200" ("PLC Type 2"), "error in (no error)"=w2258, "IP address"=w2255) -> ("error out"=w2260:errorcluster, "S7 Connection out"=w2259:T5)  [unwired: 5 in]
                  }
                }
              }
            }
            n682 = Unbundle By Name(w2237) -> ("status"=w2240:bool)
            n683 = Not(x=w2240) -> (.not. x?=w2239:bool)
            "PLC 5" <- w2239
            n684 = global write "Global 1.vi" "PLC 5"(w2239) -> ()
          }
        }
        n685 = call "PADMINI_STOP_ALL.vi"("Enum"=enum16{"Read", "Write"}."Read") -> ("Boolean 2"=w2151:bool)  [unwired: 9 in, 1 out]
        n686 = local read "stop"() -> (w2150:bool)
        n687 = Or(x=w2150, y=w2151) -> (x .or. y?=w2149:bool)
        n688 = Wait (ms)(milliseconds to wait=u32 1200) -> ()  [unwired: 1 out]
      }
      n689 = call <vilib>:"Clear Errors.vi"("error in (no error)"=w2142) -> ("error out"=w2129:errorcluster)  [unwired: 5 in, 1 out]
      n690 = call <vilib>:"disconnect.vi"("error in (no error)"=w2129, "S7 Connection in"=w2141) -> ("error out"=w2128:errorcluster)  [unwired: 8 in, 1 out]
    }
    frame Enabled {
      w2267 = PLC_Comm_State."Int"  # Enum
      n691 = while {
        shift-right: [w2282] -> _
        shift-left: w2267 -> [w2290]
        shift-right: [w2274] -> w2264
        shift-left: w2265 -> [w2289]
        shift-right: [w2285] -> _
        shift-left: _ -> [w2288]
        tunnel: w2266 -> [w2271]
        shift-right: [w2269] -> _
        shift-left: FALSE -> [w2270]
        stop <- w2283 stop-if-true
        w2279 = PLC_Comm_State."Disconnect"  # Enum
        w2287 = u32 800  # milliseconds to wait
        # "Int-->Write-->Read---if--Error-->reconnect\n               ^------v                                       v\n                ^------------------------------v"
        # "OP 60"
        n692 = case shown="\"Read\"" w2290 {
          selector: w2290 -> [w2310 w2328 w2368 w2433 w2446 w2451 _ _ _ _]
          tunnel: [w2315 w2330 w2350 w2408 w2447 w2456 w2459 w2463 w2466 w2469] -> w2291
          tunnel: [w2316 w2329 w2353 w2405 w2448 w2453 w2460 w2462 w2465 w2468] -> w2284
          tunnel: w2289 -> [w2313 w2325 w2351 w2407 w2444 w2454 w2459 w2463 w2466 w2469]
          tunnel: w2288 -> [w2311 _ w2352 w2406 w2448 w2455 w2460 w2462 w2465 w2468]
          tunnel: [w2309 w2327 w2367 w2432 w2445 w2450 _ _ _ _] -> w2286
          tunnel: [_ _ _ _ _ TRUE _ _ _ _] -> w2283
          tunnel: [w2310 w2328 w2368 w2433 w2446 w2451 _ _ _ _] -> w2280
          tunnel: w2271 -> [w2308 w2326 _ _ _ _ _ _ _ _]
          tunnel: w2270 -> [w2307 w2322 w2347 w2404 w2443 w2449 w2458 w2461 w2464 w2467]
          tunnel: [w2307 w2322 FALSE w2404 w2443 w2449 w2458 w2461 w2464 w2467] -> w2268
          frame "Connect" {
            w2309 = PLC_Comm_State."Write"  # Enum
            w2321 = TRUE  # Use Rack/Slot for S71200/1500
            w2320 = u8 1  # Slot S7 300/400
            w2318 = u8 0  # Rack S7 300/400
            # "Reconect"
            n693 = call <vilib>:"disconnect.vi"("error in (no error)"=w2313, "S7 Connection in"=w2311) -> ("error out"=w2314:errorcluster)  [unwired: 8 in, 1 out]
            n694 = call <vilib>:"Clear Errors.vi"("error in (no error)"=w2314) -> ("error out"=w2312:errorcluster)  [unwired: 5 in, 1 out]
            n695 = call <vilib>:"connect.vi"("Use Rack/Slot for S71200/1500"=w2321, "Slot S7 300/400"=w2320, "PLC Type"=PLC_Type."S7 1200" ("PLC Type 2"), "error in (no error)"=w2312, "Rack S7 300/400"=w2318, "timeout [ms]"=1000 ("timeout [ms] 2"), "IP address"=w2308) -> ("error out"=w2315:errorcluster, "S7 Connection out"=w2316:T5)  [unwired: 3 in]
          }
          frame "Int" {
            w2327 = PLC_Comm_State."Write"  # Enum
            w2331 = TRUE  # Use Rack/Slot for S71200/1500
            w2332 = u8 1  # Slot S7 300/400
            w2333 = u8 0  # Rack S7 300/400
            w2334 = u16[] [43]  # Data Block #
            # "Initialize and set first bits"
            n696 = call "Stall Data Flow.vim"("value in"=w2325, "milliseconds to wait"=u32 516) -> ("value out"=w2324:errorcluster)  [unwired: 1 out]
            n697 = call <vilib>:"connect.vi"("Use Rack/Slot for S71200/1500"=w2331, "Slot S7 300/400"=w2332, "PLC Type"=PLC_Type."S7 1200" ("PLC Type 2"), "error in (no error)"=w2324, "Rack S7 300/400"=w2333, "timeout [ms]"=1000 ("timeout [ms] 2"), "IP address"=w2326) -> ("error out"=w2336:errorcluster, "S7 Connection out"=w2335:T5)  [unwired: 3 in]
            n698 = for {
              tunnel: w2334 -> [w2344] mode=indexing
              shift-right: [w2342] -> w2329
              shift-left: w2335 -> [w2340]
              tunnel: w2336 -> [w2341]
              tunnel: [w2339] -> w2330
              w2343 = i32[] [0, 0]  # DINT input array
              # "Reset Search and save \nbit on software start"
              n699 = call-poly <vilib>:"write DB.vi"("DINT input array"=w2343, "error in (no error)"=w2341, "Data Block #"=w2344, "S7 Connection in"=w2340) -> ("error out"=w2339:errorcluster, "S7 Connection out"=w2342:T5)  [unwired: 4 in, 2 out]
            }
          }
          frame "Write" {
            w2355 = u16 44 ("Data Block #")
            w2367 = PLC_Comm_State."Read"  # Enum
            n700 = global read "DATA LOG.vi" "OP 60 Outputs"() -> (w2366:bool)
            n701 = case shown="True" w2366 {
              tunnel: w2352 -> [w2389 w2402]
              tunnel: [w2390 w2392] -> w2361
              tunnel: [w2389 w2395] -> w2360
              tunnel: w2351 -> [w2390 w2399]
              frame False {
              }
              frame True {
                w2403 = u16 44  # Data Block #
                n702 = call "PADMINI_AUTO_BARCODE_STATUS 60.vi"("Enum"=enum16{"Read", "Write"}."Read", "error in (no error)"=w2399) -> ("error out"=w2398:errorcluster, "O/P"=w2400:i32[])  [unwired: 8 in]
                n703 = call-poly <vilib>:"write DB.vi"("DINT input array"=w2400, "error in (no error)"=w2398, "Data Block #"=w2403, "S7 Connection in"=w2402) -> ("error out"=w2393:errorcluster, "S7 Connection out"=w2394:T5)  [unwired: 4 in, 2 out]
                n704 = call-poly <vilib>:"write DB.vi"("DINT input array"=i32[] [0] ("Data Byte"), "error in (no error)"=w2393, "Data Block #"=u16 43, "S7 Connection in"=w2394) -> ("error out"=w2392:errorcluster, "S7 Connection out"=w2395:T5)  [unwired: 4 in, 2 out]
                n705 = Unbundle By Name(w2392) -> ("status"=w2391:bool)
                n706 = global write "DATA LOG.vi" "OP 60 Outputs"(w2391) -> ()
              }
            }
            n707 = global read "DATA LOG.vi" "OP 60 reset"() -> (w2359:bool)
            n708 = global read "DATA LOG.vi" "Auto Cycle On"() -> (w2358:bool)
            n709 = Boolean To (0,1)(Boolean=w2358) -> (0, 1=w2357:i16)
            n710 = case shown="True" w2359 {
              tunnel: w2361 -> [w2379 w2388]
              tunnel: [w2379 w2382] -> w2362
              tunnel: w2360 -> [w2380 w2387]
              tunnel: [w2380 w2386] -> w2363
              frame False {
              }
              frame True {
                n711 = call-poly <vilib>:"write DB.vi"("Item offset [byte]"=u16 4 ("Data Block #"), "DINT input array"=i32[] [0], "error in (no error)"=w2388, "Data Block #"=u16 43, "S7 Connection in"=w2387) -> ("error out"=w2382:errorcluster, "S7 Connection out"=w2386:T5)  [unwired: 3 in, 2 out]
                n712 = Unbundle By Name(w2382) -> ("status"=w2381:bool)
                n713 = global write "DATA LOG.vi" "OP 60 reset"(w2381) -> ()
              }
            }
            n714 = Build Array(w2357) -> (w2356:i16[])
            n715 = global read "Global 1.vi" "Filtered BARCODE selected"() -> (w2349:string[])
            n716 = call-poly <vilib>:"write DB.vi"("Item offset [byte]"=u32 20, "DINT input array"=w2356, "error in (no error)"=w2362, "Data Block #"=w2355, "S7 Connection in"=w2363) -> ("error out"=w2365:errorcluster, "S7 Connection out"=w2364:T5)  [unwired: 3 in, 2 out]
            n717 = call "Is Value Changed.vim"("value"=w2349) -> ("changed or first call?"=w2346:bool)
            n718 = Or(x=w2347, y=w2346) -> (x .or. y?=w2348:bool)
            n719 = case shown="False" w2348 {
              tunnel: w2349 -> [_ w2378]
              tunnel: w2365 -> [w2369 w2377]
              tunnel: w2364 -> [w2370 w2376]
              tunnel: w2355 -> [_ w2373]
              tunnel: [w2370 w2372] -> w2353
              tunnel: [w2369 w2371] -> w2350
              frame False {
              }
              frame True {
                n720 = call-poly <vilib>:"write DB.vi"("Item offset [byte]"=u32 24, "Input STRINGS"=w2378, "error in (no error)"=w2377, "String length reserved in DB (default=254)"=u16 15, "Data Block #"=w2373, "S7 Connection in"=w2376) -> ("error out"=w2371:errorcluster, "S7 Connection out"=w2372:T5)  [unwired: 2 in, 2 out]
              }
            }
          }
          frame "Read" {
            w2414 = u16 43 ("Data Block #")
            w2432 = PLC_Comm_State."Write"  # Enum
            n721 = call-poly <vilib>:"read DB.vi"("Item offset [byte]"=u32 8, "error in (no error)"=w2407, "items #"=u16 6 ("Items # [byte]"), "Data Block #"=w2414, "S7 Connection in"=w2406) -> ("error out"=w2428:errorcluster, "REAL result array"=w2431:sgl[], "S7 Connection out"=w2429:T5)  [unwired: 4 in]
            n722 = call-poly <vilib>:"read DB.vi"("Item offset [byte]"=u32 32, "String length reserved in DB (default=254)"=u16 50, "error in (no error)"=w2428, "items #"=u16 1 ("Items # [byte]"), "Data Block #"=w2414, "S7 Connection in"=w2429) -> ("error out"=w2425:errorcluster, "STRING result Array"=w2423:string[], "S7 Connection out"=w2424:T5)  [unwired: 2 in, 1 out]
            n723 = call-poly <vilib>:"read DB.vi"("Item offset [byte]"=u32 84, "String length reserved in DB (default=254)"=u16 10, "error in (no error)"=w2425, "items #"=u16 7 ("Items # [byte]"), "Data Block #"=w2414, "S7 Connection in"=w2424) -> ("error out"=w2426:errorcluster, "STRING result Array"=w2427:string[], "S7 Connection out"=w2420:T5)  [unwired: 2 in, 1 out]
            n724 = Build Array (concatenate)(w2423, w2427) -> (w2430:string[])
            n725 = call-poly <vilib>:"read DB.vi"("error in (no error)"=w2426, "items #"=u16 2 ("Items # [byte]"), "Data Block #"=u16 43, "S7 Connection in"=w2420) -> ("error out"=w2422:errorcluster, "DINT result array"=w2421:i32[], "S7 Connection out"=w2405:T5)  [unwired: 5 in]
            n726 = case shown="No Error" w2422 {
              selector: w2422 -> [w2435 w2442]
              tunnel: w2421 -> [w2434 _]
              tunnel: w2430 -> [w2441 _]
              tunnel: w2431 -> [w2439 _]
              tunnel: [w2436 w2442] -> w2408
              frame No Error {
                w2440 = enum16{"Read", "Write"}."Write" ("Enum")
                n727 = call "PADMINI_AUTO_BARCODE_STRING 60.vi"("Enum"=w2440, "error in (no error)"=w2435, "Input"=w2441) -> ("error out"=w2438:errorcluster)  [unwired: 7 in, 1 out]
                n728 = call "PADMINI_AUTO_CYCLE VALUE 60.vi"("Enum"=w2440, "error in (no error)"=w2438, "Input"=w2439) -> ("error out"=w2437:errorcluster)  [unwired: 7 in, 1 out]
                n729 = call "PADMINI_AUTO_CYCLE STATE 60.vi"("Enum"=w2440, "error in (no error)"=w2437, "Input"=w2434) -> ("error out"=w2436:errorcluster)  [unwired: 7 in, 1 out]
              }
              frame Error {
              }
            }
          }
          frame "Error" {
            w2445 = PLC_Comm_State."Connect"  # Enum
            n730 = global write "Global 1.vi" "PLC5 error"(w2444) -> ()
            n731 = call <vilib>:"Clear Errors.vi"("error in (no error)"=w2444) -> ("error out"=w2447:errorcluster)  [unwired: 5 in, 1 out]
          }
          frame "Disconnect" {
            w2450 = PLC_Comm_State."Disconnect"  # Enum
            w2453 = T5 {"TCP Connection Ref"=refnum, "IP address"="", "timeout ms"=5000, "Connected?"=FALSE, "PLC Type"=enum."S7 1200", "Rack S7 400"=0, "Slot S7 400"=0, "PDU Size"=0, "connection semaphore"=refnum}  # S7 Connection out
            n732 = call <vilib>:"Clear Errors.vi"("error in (no error)"=w2454) -> ("error out"=w2457:errorcluster)  [unwired: 5 in, 1 out]
            n733 = call <vilib>:"disconnect.vi"("error in (no error)"=w2457, "S7 Connection in"=w2455) -> ("error out"=w2456:errorcluster)  [unwired: 8 in, 1 out]
          }
          frame "Write2" {
            # "No Use"
          }
          frame "Write3" {
            # "No Use"
          }
          frame "Read2" {
            # "No Use"
          }
          frame "Read3" {
            # "No Use"
          }
        }
        n734 = Wait (ms)(milliseconds to wait=w2287) -> ()  [unwired: 1 out]
        n735 = call "PADMINI_STOP_ALL.vi"("Enum"=enum16{"Read", "Write"}."Read") -> ("Boolean 2"=w2278:bool)  [unwired: 9 in, 1 out]
        n736 = local read "stop"() -> (w2273:bool)
        n737 = case shown="Error" w2291 {
          selector: w2291 -> [w2295 w2302]
          tunnel: [w2295 w2301] -> w2274
          tunnel: [w2294 w2300] -> w2281
          tunnel: w2286 -> [w2294 _]
          tunnel: [w2293 w2306] -> w2285
          tunnel: w2284 -> [w2293 w2306]
          tunnel: w2280 -> [_ w2305]
          tunnel: [w2292 TRUE] -> w2269
          tunnel: w2268 -> [w2292 _]
          frame No Error {
          }
          frame Error {
            w2300 = PLC_Comm_State."Error"  # Enum
            w2297 = "    " ("string")
            n738 = Unbundle By Name(w2302) -> ("source"=w2298:string)
            n739 = Get Date/Time String() -> (time string=w2296:string)  [unwired: 3 in, 1 out]
            n740 = call <userlib>:"Get Strings from Enum__ogtk.vi"("Enum"=w2305) -> ("String Value"=w2304:string)  [unwired: 7 in, 3 out]
            n741 = Concatenate Strings(w2304, w2297, w2296, w2297, w2298) -> (w2303:string)
            n742 = Bundle By Name(cluster=w2302, "source"=w2303) -> (w2301:errorcluster)
          }
        }
        n743 = Or(x=w2273, y=w2278) -> (x .or. y?=w2276:bool)
        n744 = Select(t=w2279, s=w2276, f=w2281) -> (s? t:f=w2282:T1)
        n745 = Unbundle By Name(w2274) -> ("status"=w2275:bool)
        n746 = Not(x=w2275) -> (.not. x?=w2272:bool)
        n747 = global write "Global 1.vi" "PLC 5"(w2272) -> ()
      }
    }
  }
  n748 = disable-structure shown="Enabled" {
    disable-tunnel: [w2483 _] -> w118
    disable-tunnel: [w2480 _] -> w107
    disable-tunnel: w83 -> [w2479 w2546]
    disable-tunnel: w10 -> [w2473 w2545]
    frame Disabled {
      n749 = call <vilib>:"connect.vi"("Use Rack/Slot for S71200/1500"=TRUE, "Slot S7 300/400"=u8 1, "PLC Type"=PLC_Type."S7 1200" ("PLC Type 2"), "error in (no error)"=w2473, "Rack S7 300/400"=u8 0, "timeout [ms]"=1000, "IP address"=w2479) -> ("error out"=w2475:errorcluster, "S7 Connection out"=w2474:T5)  [unwired: 3 in]
      n750 = for {
        tunnel: u16[] [83, 94] ("Data Block #") -> [w2489] mode=indexing
        shift-right: [w2487] -> w2477
        shift-left: w2474 -> [w2484]
        tunnel: w2475 -> [w2485]
        tunnel: [w2486] -> w2476
        w2488 = i32[] [0, 0]  # DINT input array
        # "Reset Search and save \nbit on software start"
        n751 = call-poly <vilib>:"write DB.vi"("DINT input array"=w2488, "error in (no error)"=w2485, "Data Block #"=w2489, "S7 Connection in"=w2484) -> ("error out"=w2486:errorcluster, "S7 Connection out"=w2487:T5)  [unwired: 4 in, 2 out]
      }
      n752 = while {
        shift-right: [w2492] -> w2480
        shift-left: w2477 -> [w2502]
        shift-right: [w2500] -> w2483
        shift-left: w2476 -> [w2501]
        tunnel: w2479 -> [w2490]
        stop <- w2495 stop-if-true
        # "OP 10 AND 20"
        n753 = flat-sequence {
          tunnel: [w2505] -> w2494
          tunnel: [w2511] -> w2493
          tunnel: w2501 -> [w2512]
          tunnel: w2502 -> [w2513]
          tunnel: [w2510] -> w2491
          tunnel: w2490 -> [w2510]
          tunnel: [w2517] -> w2500
          tunnel: [w2516] -> w2492
          tunnel: w2494 -> [w2518]
          tunnel: w2493 -> [w2514]
          tunnel: w2491 -> [w2515]
          frame #0 {
            # "NEW CHANGES"
            n754 = call "PLC_OP10_Write.vi"("error in (no error)"=w2512, "S7 Connection in"=w2513) -> ("error out"=w2508:errorcluster, "S7 Connection out"=w2509:T5)  [unwired: 8 in]
            n755 = call "PLC_OP10_Read.vi"("error in (no error)"=w2508, "S7 Connection in"=w2509) -> ("error out"=w2507:errorcluster, "S7 Connection out"=w2506:T5)  [unwired: 8 in]
            n756 = call "PLC_OP20_Write.vi"("error in (no error)"=w2507, "S7 Connection in"=w2506) -> ("error out"=w2503:errorcluster, "S7 Connection out"=w2504:T5)  [unwired: 8 in]
            n757 = call "PLC_OP20_Read.vi"("error in (no error)"=w2503, "S7 Connection in"=w2504) -> ("error out"=w2511:errorcluster, "S7 Connection out 2"=w2505:T5)  [unwired: 8 in]
          }
          frame #1 {
            # "RECONNECT"
            n758 = case shown="Error" w2514 {
              selector: w2514 -> [w2522 w2524]
              tunnel: [w2521 w2527] -> w2516
              tunnel: [w2522 w2528] -> w2517
              tunnel: w2518 -> [w2521 w2526]
              tunnel: w2515 -> [_ w2525]
              frame No Error {
              }
              frame Error {
                n759 = Unbundle By Name(w2524) -> ("code"=w2523:i32)
                n760 = case shown="1, 66" w2523 {
                  tunnel: w2524 -> [w2529 w2542]
                  tunnel: [w2530 w2540] -> w2528
                  tunnel: [w2531 w2539] -> w2527
                  tunnel: w2526 -> [w2531 w2536]
                  tunnel: w2525 -> [_ w2535]
                  frame 0, Default {
                    n761 = call <vilib>:"Clear Errors.vi"("error in (no error)"=w2529) -> ("error out"=w2530:errorcluster)  [unwired: 5 in, 1 out]
                    n762 = global write "Global 1.vi" "PLC1 error"(w2529) -> ()
                  }
                  frame 1, 66 {
                    w2534 = 1000  # timeout [ms]
                    n763 = call <vilib>:"Clear Errors.vi"("error in (no error)"=w2542) -> ("error out"=w2543:errorcluster)  [unwired: 5 in, 1 out]
                    n764 = call <vilib>:"disconnect.vi"("error in (no error)"=w2543, "S7 Connection in"=w2536) -> ("error out"=w2541:errorcluster)  [unwired: 8 in, 1 out]
                    n765 = call <vilib>:"Clear Errors.vi"("error in (no error)"=w2541) -> ("error out"=w2538:errorcluster)  [unwired: 5 in, 1 out]
                    n766 = call <vilib>:"connect.vi"("Use Rack/Slot for S71200/1500"=TRUE, "Slot S7 300/400"=u8 1, "PLC Type"=PLC_Type."S7 1200" ("PLC Type 2"), "error in (no error)"=w2538, "timeout [ms]"=w2534, "IP address"=w2535) -> ("error out"=w2540:errorcluster, "S7 Connection out"=w2539:T5)  [unwired: 4 in]
                  }
                }
              }
            }
            n767 = Unbundle By Name(w2514) -> ("status"=w2520:bool)
            n768 = Not(x=w2520) -> (.not. x?=w2519:bool)
            "PLC 1" <- w2519
            n769 = global write "Global 1.vi" "PLC 1"(w2519) -> ()
          }
        }
        n770 = call "PADMINI_STOP_ALL.vi"("Enum"=enum16{"Read", "Write"}."Read") -> ("Boolean 2"=w2497:bool)  [unwired: 9 in, 1 out]
        n771 = Wait (ms)(milliseconds to wait=u32 1200) -> ()  [unwired: 1 out]
        n772 = Or(x="stop", y=w2497) -> (x .or. y?=w2495:bool)
      }
    }
    frame Enabled {
      w2547 = PLC_Comm_State."Int"  # Enum
      n773 = while {
        shift-right: [w2562] -> _
        shift-left: w2547 -> [w2570]
        shift-right: [w2554] -> _
        shift-left: w2545 -> [w2569]
        shift-right: [w2565] -> _
        shift-left: _ -> [w2568]
        tunnel: w2546 -> [w2551]
        shift-right: [w2548] -> _
        shift-left: FALSE -> [w2550]
        stop <- w2563 stop-if-true
        w2559 = PLC_Comm_State."Disconnect"  # Enum
        w2567 = u32 800  # milliseconds to wait
        # "Int-->Write-->Read---if--Error-->reconnect\n               ^------v                                       v\n                ^------------------------------v"
        # "OP 10-20"
        n774 = case shown="\"Read\"" w2570 {
          selector: w2570 -> [w2590 w2606 w2629 w2636 w2644 w2650 w2655 w2660 _ _]
          tunnel: [w2595 w2609 w2626 w2632 w2641 w2648 w2656 w2665 w2669 w2672] -> w2571
          tunnel: [w2596 w2608 w2624 w2634 w2639 w2646 w2657 w2662 w2668 w2671] -> w2564
          tunnel: w2569 -> [w2593 w2607 w2627 w2633 w2642 w2649 w2653 w2663 w2669 w2672]
          tunnel: w2568 -> [w2591 _ w2625 w2635 w2640 w2647 w2657 w2664 w2668 w2671]
          tunnel: [w2589 w2605 w2628 w2637 w2643 w2651 w2654 w2659 _ _] -> w2566
          tunnel: [_ _ _ _ _ _ _ TRUE _ _] -> w2563
          tunnel: [w2590 w2606 w2629 w2636 w2644 w2650 w2655 w2660 _ _] -> w2560
          tunnel: w2551 -> [w2588 w2604 _ _ _ _ _ _ _ _]
          tunnel: w2550 -> [w2587 w2602 w2623 w2631 w2638 w2645 w2652 w2658 w2667 w2670]
          tunnel: [w2587 w2602 w2623 FALSE w2638 w2645 w2652 w2658 w2667 w2670] -> w2549
          frame "Connect" {
            w2589 = PLC_Comm_State."Write"  # Enum
            w2601 = TRUE  # Use Rack/Slot for S71200/1500
            w2600 = u8 1  # Slot S7 300/400
            w2598 = u8 0  # Rack S7 300/400
            # "Reconect"
            n775 = call <vilib>:"disconnect.vi"("error in (no error)"=w2593, "S7 Connection in"=w2591) -> ("error out"=w2594:errorcluster)  [unwired: 8 in, 1 out]
            n776 = call <vilib>:"Clear Errors.vi"("error in (no error)"=w2594) -> ("error out"=w2592:errorcluster)  [unwired: 5 in, 1 out]
            n777 = call <vilib>:"connect.vi"("Use Rack/Slot for S71200/1500"=w2601, "Slot S7 300/400"=w2600, "PLC Type"=PLC_Type."S7 1200" ("PLC Type 2"), "error in (no error)"=w2592, "Rack S7 300/400"=w2598, "timeout [ms]"=1000 ("timeout [ms] 2"), "IP address"=w2588) -> ("error out"=w2595:errorcluster, "S7 Connection out"=w2596:T5)  [unwired: 3 in]
          }
          frame "Int" {
            w2605 = PLC_Comm_State."Write"  # Enum
            w2610 = TRUE  # Use Rack/Slot for S71200/1500
            w2611 = u8 1  # Slot S7 300/400
            w2612 = u8 0  # Rack S7 300/400
            # "Initialize and set first bits"
            n778 = call <vilib>:"connect.vi"("Use Rack/Slot for S71200/1500"=w2610, "Slot S7 300/400"=w2611, "PLC Type"=PLC_Type."S7 1200" ("PLC Type 2"), "error in (no error)"=w2607, "Rack S7 300/400"=w2612, "timeout [ms]"=1000 ("timeout [ms] 2"), "IP address"=w2604) -> ("error out"=w2614:errorcluster, "S7 Connection out"=w2613:T5)  [unwired: 3 in]
            n779 = for {
              tunnel: u16[] [83, 94] ("Data Block #") -> [w2622] mode=indexing
              shift-right: [w2620] -> w2608
              shift-left: w2613 -> [w2618]
              tunnel: w2614 -> [w2619]
              tunnel: [w2617] -> w2609
              w2621 = i32[] [0, 0]  # DINT input array
              # "Reset Search and save \nbit on software start"
              n780 = call-poly <vilib>:"write DB.vi"("DINT input array"=w2621, "error in (no error)"=w2619, "Data Block #"=w2622, "S7 Connection in"=w2618) -> ("error out"=w2617:errorcluster, "S7 Connection out"=w2620:T5)  [unwired: 4 in, 2 out]
            }
          }
          frame "Write" {
            w2628 = PLC_Comm_State."Write2"  # Enum
            # "OP 10 Write"
            n781 = call "PLC_OP10_Write.vi"("S7 Connection in"=w2625, "value change as error ?"=w2623, "error in (no error)"=w2627) -> ("S7 Connection out"=w2624:T5, "error out"=w2626:errorcluster)  [unwired: 11 in]
          }
          frame "Write2" {
            w2637 = PLC_Comm_State."Read"  # Enum
            # "op 20 wirte 2"
            n782 = call "PLC_OP20_Write.vi"("S7 Connection in"=w2635, "value change as error ?"=w2631, "error in (no error)"=w2633) -> ("S7 Connection out"=w2634:T5, "error out"=w2632:errorcluster)  [unwired: 6 in]
          }
          frame "Read" {
            w2643 = PLC_Comm_State."Read2"  # Enum
            # "OP10 read"
            n783 = call "PLC_OP10_Read.vi"("error in (no error)"=w2642, "S7 Connection in"=w2640) -> ("error out"=w2641:errorcluster, "S7 Connection out"=w2639:T5)  [unwired: 8 in]
          }
          frame "Read2" {
            w2651 = PLC_Comm_State."Write"  # Enum
            # "Op20 Read2"
            n784 = call "PLC_OP20_Read.vi"("error in (no error)"=w2649, "S7 Connection in"=w2647) -> ("error out"=w2648:errorcluster, "S7 Connection out 2"=w2646:T5)  [unwired: 8 in]
          }
          frame "Error" {
            w2654 = PLC_Comm_State."Connect"  # Enum
            n785 = global write "Global 1.vi" "PLC1 error"(w2653) -> ()
            n786 = call <vilib>:"Clear Errors.vi"("error in (no error)"=w2653) -> ("error out"=w2656:errorcluster)  [unwired: 5 in, 1 out]
          }
          frame "Disconnect" {
            w2659 = PLC_Comm_State."Disconnect"  # Enum
            w2662 = T5 {"TCP Connection Ref"=refnum, "IP address"="", "timeout ms"=5000, "Connected?"=FALSE, "PLC Type"=enum."S7 1200", "Rack S7 400"=0, "Slot S7 400"=0, "PDU Size"=0, "connection semaphore"=refnum}  # S7 Connection out
            n787 = call <vilib>:"Clear Errors.vi"("error in (no error)"=w2663) -> ("error out"=w2666:errorcluster)  [unwired: 5 in, 1 out]
            n788 = call <vilib>:"disconnect.vi"("error in (no error)"=w2666, "S7 Connection in"=w2664) -> ("error out"=w2665:errorcluster)  [unwired: 8 in, 1 out]
          }
          frame "Write3" {
            # "No Use"
          }
          frame "Read3" {
            # "No Use"
          }
        }
        n789 = Wait (ms)(milliseconds to wait=w2567) -> ()  [unwired: 1 out]
        n790 = call "PADMINI_STOP_ALL.vi"("Enum"=enum16{"Read", "Write"}."Read") -> ("Boolean 2"=w2558:bool)  [unwired: 9 in, 1 out]
        n791 = local read "stop"() -> (w2553:bool)
        n792 = case shown="Error" w2571 {
          selector: w2571 -> [w2575 w2582]
          tunnel: [w2575 w2581] -> w2554
          tunnel: [w2574 w2580] -> w2561
          tunnel: w2566 -> [w2574 _]
          tunnel: [w2573 w2586] -> w2565
          tunnel: w2564 -> [w2573 w2586]
          tunnel: w2560 -> [_ w2585]
          tunnel: w2549 -> [w2572 _]
          tunnel: [w2572 TRUE] -> w2548
          frame No Error {
          }
          frame Error {
            w2580 = PLC_Comm_State."Error"  # Enum
            w2577 = "    " ("string")
            n793 = Unbundle By Name(w2582) -> ("source"=w2578:string)
            n794 = Get Date/Time String() -> (time string=w2576:string)  [unwired: 3 in, 1 out]
            n795 = call <userlib>:"Get Strings from Enum__ogtk.vi"("Enum"=w2585) -> ("String Value"=w2584:string)  [unwired: 7 in, 3 out]
            n796 = Concatenate Strings(w2584, w2577, w2576, w2577, w2578) -> (w2583:string)
            n797 = Bundle By Name(cluster=w2582, "source"=w2583) -> (w2581:errorcluster)
          }
        }
        n798 = Or(x=w2553, y=w2558) -> (x .or. y?=w2556:bool)
        n799 = Unbundle By Name(w2554) -> ("status"=w2555:bool)
        n800 = Select(t=w2559, s=w2556, f=w2561) -> (s? t:f=w2562:T1)
        n801 = Not(x=w2555) -> (.not. x?=w2552:bool)
        n802 = global write "Global 1.vi" "PLC 1"(w2552) -> ()
      }
    }
  }
  n803 = while {
    shift-right: [w2686] -> _
    shift-left: w2 -> [w2695]
    shift-right: [w2676] -> w85
    shift-left: w10 -> [w2694]
    shift-right: [w2689] -> _
    shift-left: _ -> [w2693]
    tunnel: w84 -> [w2692]
    shift-right: [w2673] -> _
    shift-left: FALSE -> [w2675]
    stop <- w2687 stop-if-true
    w2683 = PLC_Comm_State."Disconnect"  # Enum
    w2691 = u32 800  # milliseconds to wait
    # "Int-->Write-->Read---if--Error-->reconnect\n               ^------v                                       v\n                ^------------------------------v"
    # "OP 30"
    n804 = case shown="\"Write\"" w2695 {
      selector: w2695 -> [w2714 w2731 w2757 w2764 w2768 w2773 _ _ _ _]
      tunnel: [w2719 w2735 w2752 w2760 w2769 w2778 w2781 w2785 w2788 w2791] -> w2696
      tunnel: [w2720 w2734 w2754 w2761 w2770 w2775 w2782 w2784 w2787 w2790] -> w2688
      tunnel: w2694 -> [w2717 w2733 w2753 w2759 w2766 w2776 w2781 w2785 w2788 w2791]
      tunnel: w2693 -> [w2715 _ w2755 w2762 w2770 w2777 w2782 w2784 w2787 w2790]
      tunnel: w2692 -> [w2721 w2732 _ _ _ _ _ _ _ _]
      tunnel: [w2713 w2730 w2756 w2763 w2767 w2772 _ _ _ _] -> w2690
      tunnel: [_ _ _ _ _ TRUE _ _ _ _] -> w2687
      tunnel: [w2714 w2731 w2757 w2764 w2768 w2773 _ _ _ _] -> w2684
      tunnel: w2675 -> [w2712 w2727 w2751 w2758 w2765 w2771 w2780 w2783 w2786 w2789]
      tunnel: [w2712 w2727 FALSE w2758 w2765 w2771 w2780 w2783 w2786 w2789] -> w2674
      frame "Connect" {
        w2713 = PLC_Comm_State."Write"  # Enum
        w2726 = TRUE  # Use Rack/Slot for S71200/1500
        w2725 = u8 1  # Slot S7 300/400
        w2723 = u8 0  # Rack S7 300/400
        # "Reconect"
        n805 = call <vilib>:"disconnect.vi"("error in (no error)"=w2717, "S7 Connection in"=w2715) -> ("error out"=w2718:errorcluster)  [unwired: 8 in, 1 out]
        n806 = call <vilib>:"Clear Errors.vi"("error in (no error)"=w2718) -> ("error out"=w2716:errorcluster)  [unwired: 5 in, 1 out]
        n807 = call <vilib>:"connect.vi"("Use Rack/Slot for S71200/1500"=w2726, "Slot S7 300/400"=w2725, "PLC Type"=PLC_Type."S7 1200" ("PLC Type 2"), "error in (no error)"=w2716, "Rack S7 300/400"=w2723, "timeout [ms]"=1000 ("timeout [ms] 2"), "IP address"=w2721) -> ("error out"=w2719:errorcluster, "S7 Connection out"=w2720:T5)  [unwired: 3 in]
      }
      frame "Int" {
        w2730 = PLC_Comm_State."Write"  # Enum
        w2736 = TRUE  # Use Rack/Slot for S71200/1500
        w2737 = u8 1  # Slot S7 300/400
        w2738 = u8 0  # Rack S7 300/400
        w2739 = u16[] [37]  # Data Block #
        n808 = call "Stall Data Flow.vim"("value in"=w2733, "milliseconds to wait"=u32 129) -> ("value out"=w2729:errorcluster)  [unwired: 1 out]
        n809 = call <vilib>:"connect.vi"("Use Rack/Slot for S71200/1500"=w2736, "Slot S7 300/400"=w2737, "PLC Type"=PLC_Type."S7 1200" ("PLC Type 2"), "error in (no error)"=w2729, "Rack S7 300/400"=w2738, "timeout [ms]"=1000 ("timeout [ms] 2"), "IP address"=w2732) -> ("error out"=w2741:errorcluster, "S7 Connection out"=w2740:T5)  [unwired: 3 in]
        n810 = for {
          tunnel: w2739 -> [w2749] mode=indexing
          shift-right: [w2747] -> w2734
          shift-left: w2740 -> [w2745]
          tunnel: w2741 -> [w2746]
          tunnel: [w2744] -> w2735
          w2748 = i32[] [0, 0]  # DINT input array
          # "Reset Search and save \nbit on software start"
          n811 = call-poly <vilib>:"write DB.vi"("DINT input array"=w2748, "error in (no error)"=w2746, "Data Block #"=w2749, "S7 Connection in"=w2745) -> ("error out"=w2744:errorcluster, "S7 Connection out"=w2747:T5)  [unwired: 4 in, 2 out]
        }
      }
      frame "Write" {
        w2756 = PLC_Comm_State."Read"  # Enum
        n812 = call "PLC_OP30_Write.vi"("error in (no error)"=w2753, "FIRST CALL AFTER ERROR"=w2751, "S7 Connection in"=w2755) -> ("error out"=w2752:errorcluster, "S7 Connection out"=w2754:T5)  [unwired: 7 in]
      }
      frame "Read" {
        w2763 = PLC_Comm_State."Write"  # Enum
        # "OP100 OK\nOP 100 NG"
        n813 = call "PLC_OP30_Read.vi"("error in (no error)"=w2759, "S7 Connection in"=w2762) -> ("error out"=w2760:errorcluster, "S7 Connection out 2"=w2761:T5)  [unwired: 8 in]
      }
      frame "Error" {
        w2767 = PLC_Comm_State."Connect"  # Enum
        n814 = global write "Global 1.vi" "PLC2 error"(w2766) -> ()
        n815 = call <vilib>:"Clear Errors.vi"("error in (no error)"=w2766) -> ("error out"=w2769:errorcluster)  [unwired: 5 in, 1 out]
      }
      frame "Disconnect" {
        w2772 = PLC_Comm_State."Disconnect"  # Enum
        w2775 = T5 {"TCP Connection Ref"=refnum, "IP address"="", "timeout ms"=5000, "Connected?"=FALSE, "PLC Type"=enum."S7 1200", "Rack S7 400"=0, "Slot S7 400"=0, "PDU Size"=0, "connection semaphore"=refnum}  # S7 Connection out
        n816 = call <vilib>:"Clear Errors.vi"("error in (no error)"=w2776) -> ("error out"=w2779:errorcluster)  [unwired: 5 in, 1 out]
        n817 = call <vilib>:"disconnect.vi"("error in (no error)"=w2779, "S7 Connection in"=w2777) -> ("error out"=w2778:errorcluster)  [unwired: 8 in, 1 out]
      }
      frame "Write2" {
        # "SPARE"
      }
      frame "Write3" {
        # "No Use"
      }
      frame "Read2" {
        # "No Use"
      }
      frame "Read3" {
        # "No Use"
      }
    }
    n818 = Wait (ms)(milliseconds to wait=w2691) -> ()  [unwired: 1 out]
    n819 = call "PADMINI_STOP_ALL.vi"("Enum"=enum16{"Read", "Write"}."Read") -> ("Boolean 2"=w2682:bool)  [unwired: 9 in, 1 out]
    n820 = local read "stop"() -> (w2681:bool)
    n821 = case shown="Error" w2696 {
      selector: w2696 -> [w2700 w2707]
      tunnel: [w2700 w2706] -> w2676
      tunnel: [w2699 w2705] -> w2685
      tunnel: w2690 -> [w2699 _]
      tunnel: [w2698 w2711] -> w2689
      tunnel: w2688 -> [w2698 w2711]
      tunnel: w2684 -> [_ w2710]
      tunnel: w2674 -> [w2697 _]
      tunnel: [w2697 TRUE] -> w2673
      frame No Error {
      }
      frame Error {
        w2705 = PLC_Comm_State."Error"  # Enum
        w2703 = "    " ("string")
        n822 = Get Date/Time String() -> (time string=w2701:string)  [unwired: 3 in, 1 out]
        n823 = Unbundle By Name(w2707) -> ("source"=w2702:string)
        n824 = call <userlib>:"Get Strings from Enum__ogtk.vi"("Enum"=w2710) -> ("String Value"=w2709:string)  [unwired: 7 in, 3 out]
        n825 = Concatenate Strings(w2709, w2703, w2701, w2703, w2702) -> (w2708:string)
        n826 = Bundle By Name(cluster=w2707, "source"=w2708) -> (w2706:errorcluster)
      }
    }
    n827 = Or(x=w2681, y=w2682) -> (x .or. y?=w2679:bool)
    n828 = Select(t=w2683, s=w2679, f=w2685) -> (s? t:f=w2686:T1)
    n829 = Unbundle By Name(w2676) -> ("status"=w2678:bool)
    n830 = Not(x=w2678) -> (.not. x?=w2677:bool)
    n831 = global write "Global 1.vi" "PLC 2"(w2677) -> ()
  }
  n832 = Merge Errors(w85, w4, w5, w7) -> (w81:errorcluster)
  n833 = call <vilib>:"Clear Errors.vi"("error in (no error)"=w118) -> ("error out"=w108:errorcluster)  [unwired: 5 in, 1 out]
  n834 = call <vilib>:"disconnect.vi"("error in (no error)"=w108, "S7 Connection in"=w107) -> ("error out"=w106:errorcluster)  [unwired: 8 in, 1 out]
  n835 = Merge Errors(w6, w3, w8) -> (w29:errorcluster)
  n836 = Merge Errors(w106, w81, w29) -> (w123:errorcluster)
  n837 = call <vilib>:"Simple Error Handler.vi"("type of dialog (OK msg:1)"=w11, "error in (no error)"=w123) -> ("error out"=w122:errorcluster)  [unwired: 3 in, 4 out]
  n838 = control-ref of="This VI"() -> (w12:refnum<vi>)
  n839 = call <vilib>:"Clear Errors.vi"("error in (no error)"=w122) -> ("error out"=w121:errorcluster)  [unwired: 5 in, 1 out]
  n840 = invoke class="VI" method="FP.Close"(reference=w12, error in=w121) -> (error out=→"error out":errorcluster)  [unwired: 1 in, 2 out]
